vi "Autonomous Independent.vi"   [LabVIEW 2017]
doc: "This VI is called when autonomous begins, and will automatically be terminated when autonomous ends. You can carry out timed or sensor driven robot movement independently without needing to return to the caller."
uses:
  <vilib>/Rock Robotics/WPI/Solenoid/WPI_SolenoidValue.ctl
  <vilib>/Rock Robotics/Network Tables/NT Read String.vi
  Globals/Robot Global Data.vi
  <vilib>/Rock Robotics/WPI/Utilities/WPI_GetSetVariantRefNum.vi
  <vilib>/Rock Robotics/Network Tables/NT Write String.vi
  <vilib>/Rock Robotics/WPI/RobotDrive/WPI_RobotDriveArcadeDrive_Standard(NoSaturation).vi
  <vilib>/addons/control/pid/pid.llb/PID (DBL).vi
  <vilib>/addons/control/pid/NI_PID_pid.lvlib
panel:
  # "Be sure to right-click and choose Data Operations>>Make Current Value default if you want to save the array values with the VI"
types:
  T1 = typedef "WPI_SolenoidValue.ctl" = enum16{"Off", "On", "Forward", "Reverse"}
  T2 = typedef "WPI_RobotDriveDevRef.ctl" = cluster{"DevStatus":errorcluster, "Motors[]":T3[], "Square Inputs":bool, "Max Output":dbl}
  T3 = typedef "WPI_MotorControlDeviceRef.ctl" = cluster{"DeviceStatus":errorcluster, "Type":T4, "PWM":cluster{"PWM Channel":T5, "DeadBand":T6}, "CAN":cluster{"Device Number":u8, "SetOutput VI Ref":variant, "GetOutput VI Ref":variant, "Enable VI Ref":variant, "Disable VI Ref":variant, "Data":variant}, "Invert":bool, "DIO PWM":cluster{"PWM \"Enable\" Channel":T5, "DIOChannel":T7, "PWM Rate":dbl}}
  T4 = typedef "WPI_MotorControlType.ctl" = enum16{"PWM", "CAN", "DIO PWM"}
  T5 = typedef "FPGA_DIOPWMChannel.ctl" = enum8{"PWM 0", "PWM 1", "PWM 2", "PWM 3", "PWM 4", "PWM 5", "PWM 6", "PWM 7", "PWM 8", "PWM 9", "PWM MXP 0", "PWM MXP 1", "PWM MXP 2", "PWM MXP 3", "PWM MXP 4", "PWM MXP 5", "PWM MXP 6", "PWM MXP 7", "PWM MXP 8", "PWM MXP 9", "Invalid"}
  T6 = typedef "WPI_PWMDeadband.ctl" = cluster{"Name":string, "maxPositivePwm":i32, "minPositivePwm":i32, "centerPwm":i32, "maxNegativePwm":i32, "minNegativePwm":i32, "angularRange":u16}
  T7 = typedef "FPGA_DIOChannel.ctl" = enum8{"DIO 0", "DIO 1", "DIO 2", "DIO 3", "DIO 4", "DIO 5", "DIO 6", "DIO 7", "DIO 8", "DIO 9", "DIO MXP 0", "DIO MXP 1", "DIO MXP 2", "DIO MXP 3", "DIO MXP 4", "DIO MXP 5", "DIO MXP 6", "DIO MXP 7", "DIO MXP 8", "DIO MXP 9", "DIO MXP 10", "DIO MXP 11", "DIO MXP 12", "DIO MXP 13", "DIO MXP 14", "DIO MXP 15", "SPI Port CS1", "SPI Port CS2", "SPI Port CS3", "SPI Port MISO", "SPI Port MOSI", "Invalid"}
  T8 = cluster{"proportional gain (Kc)":dbl, "integral time (Ti, min)":dbl, "derivative time (Td, min)":dbl}
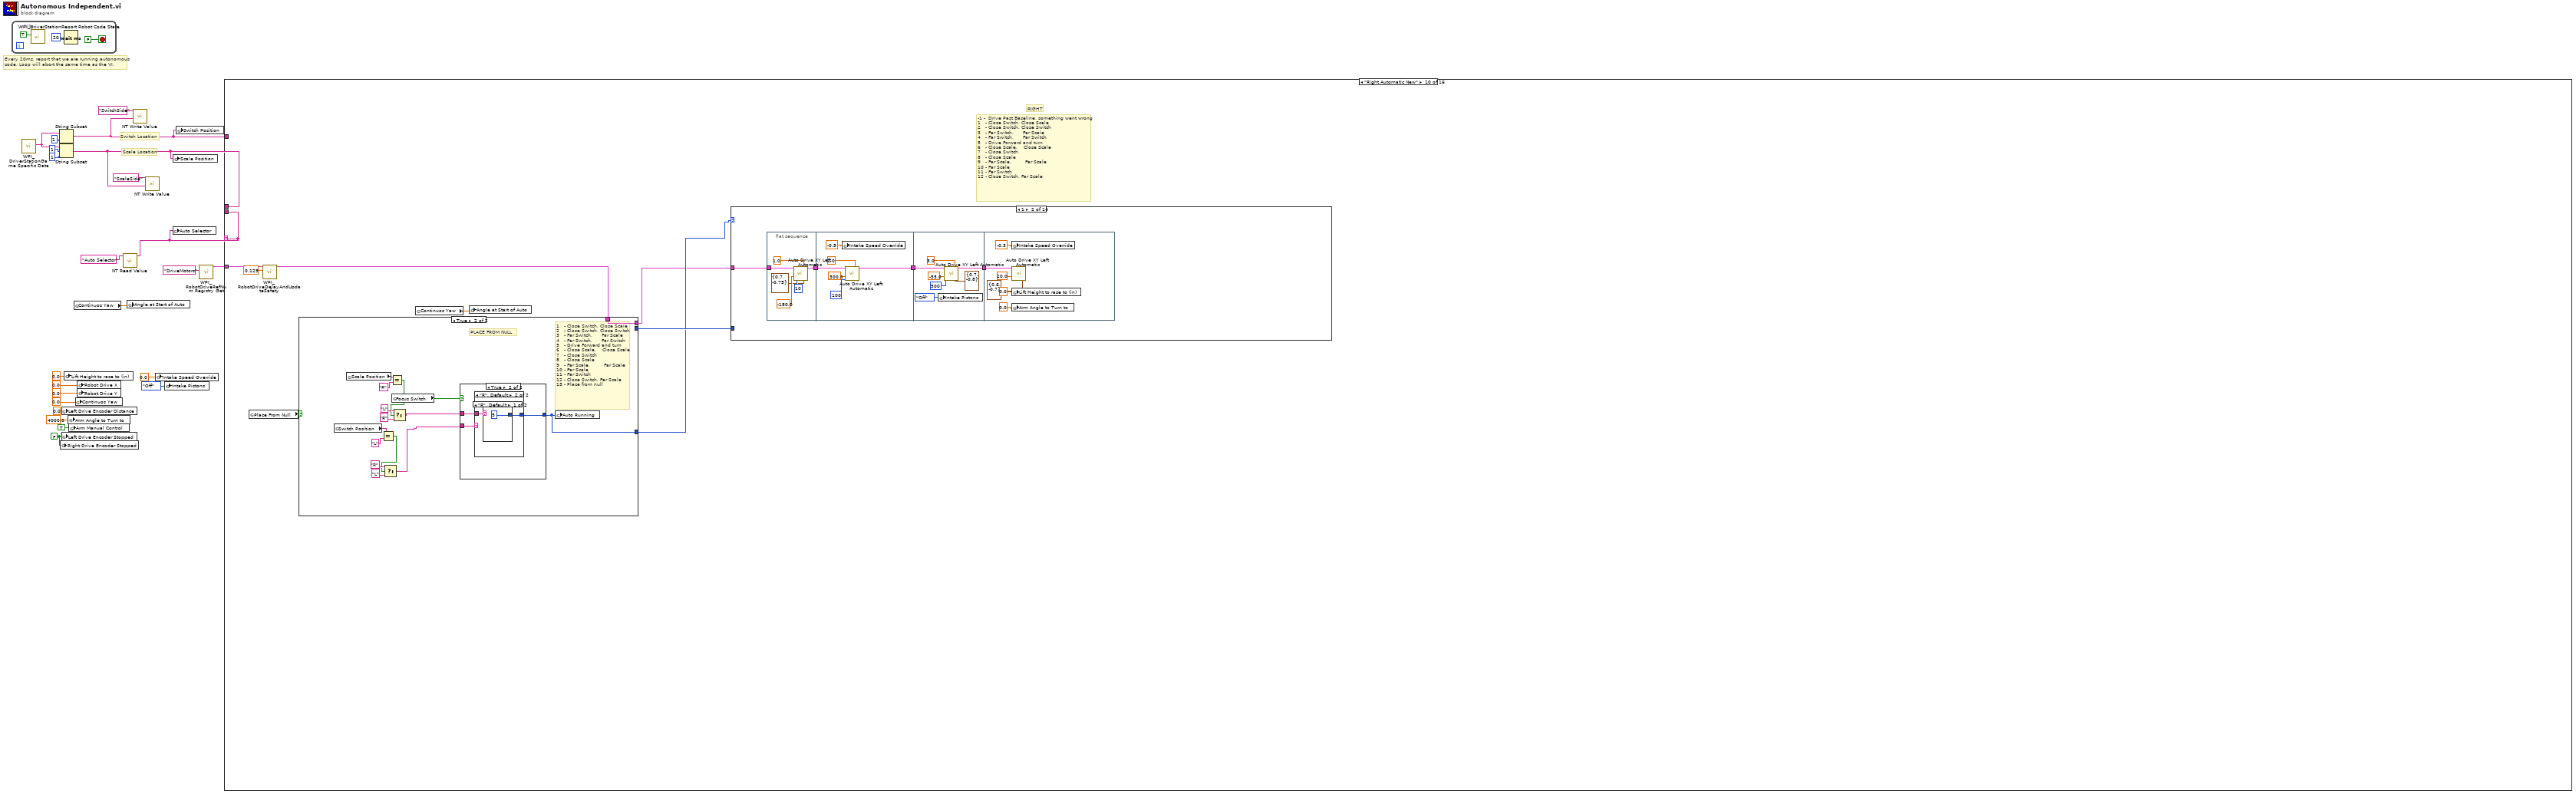
[diagram p0: block diagram]
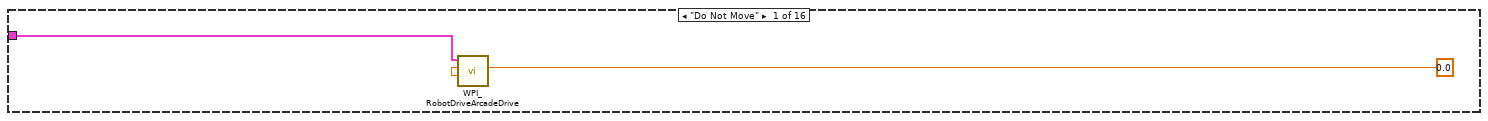
[diagram p2: hidden frame]
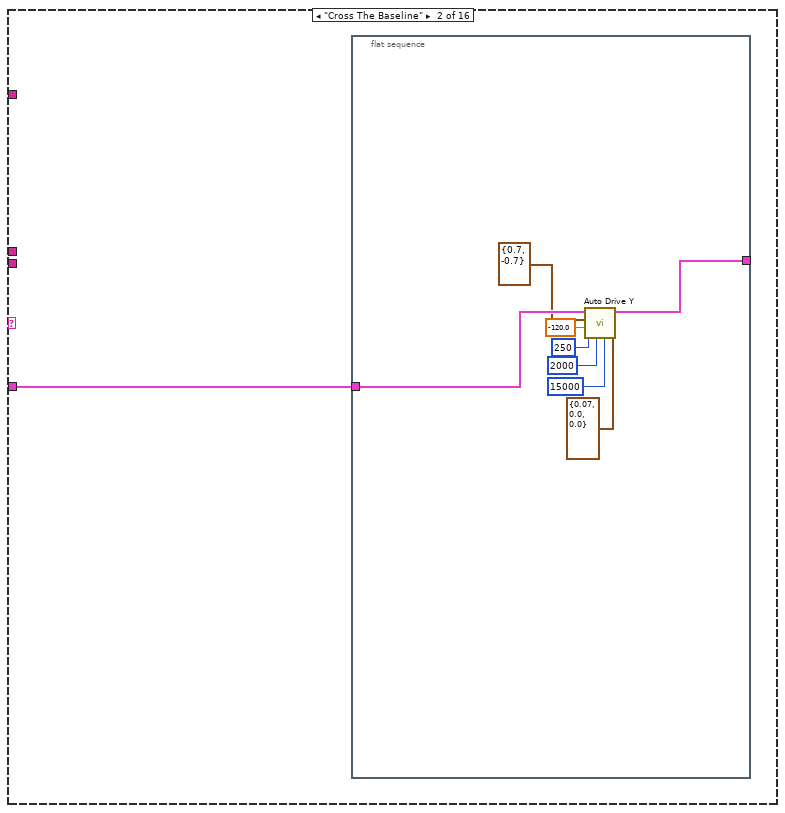
[diagram p3: hidden frame]
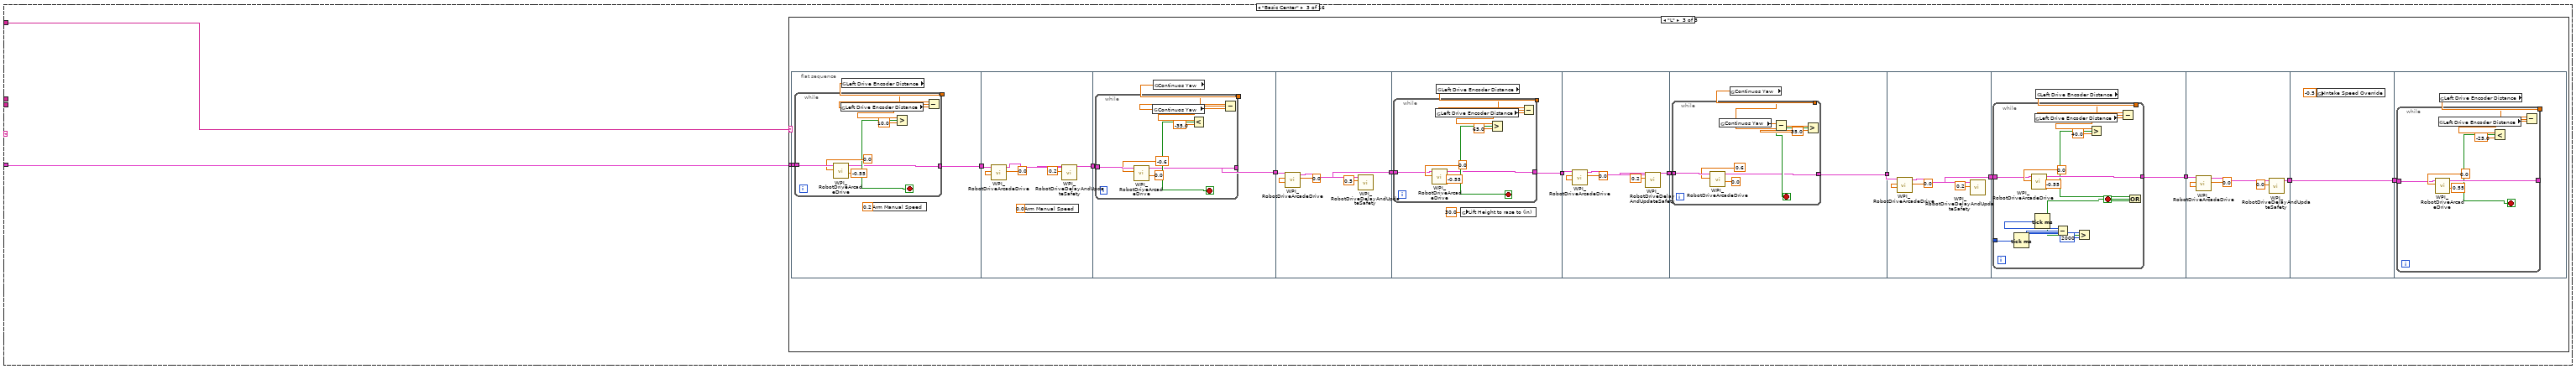
[diagram p4: hidden frame]
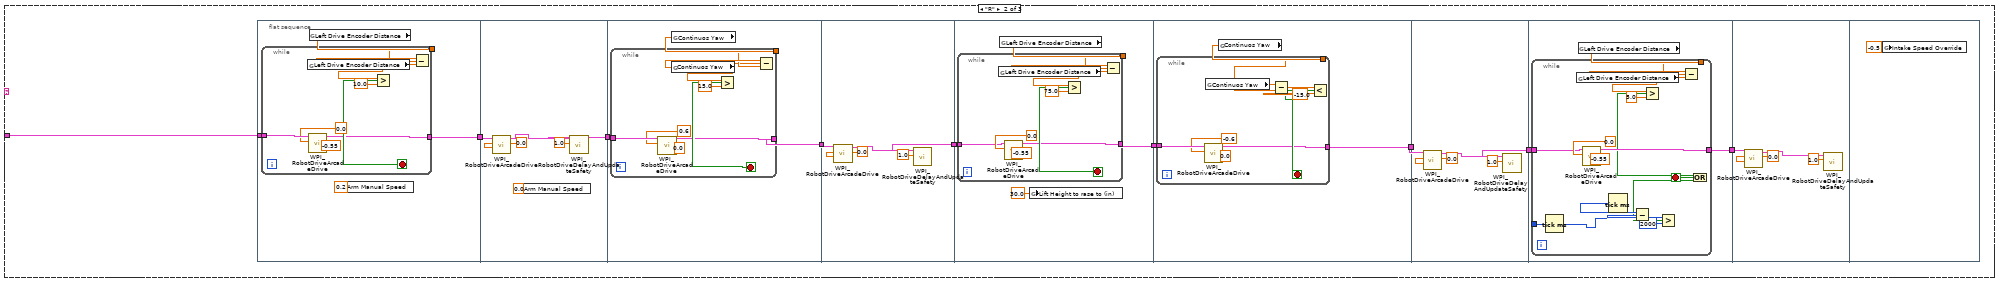
[diagram p6: hidden frame]
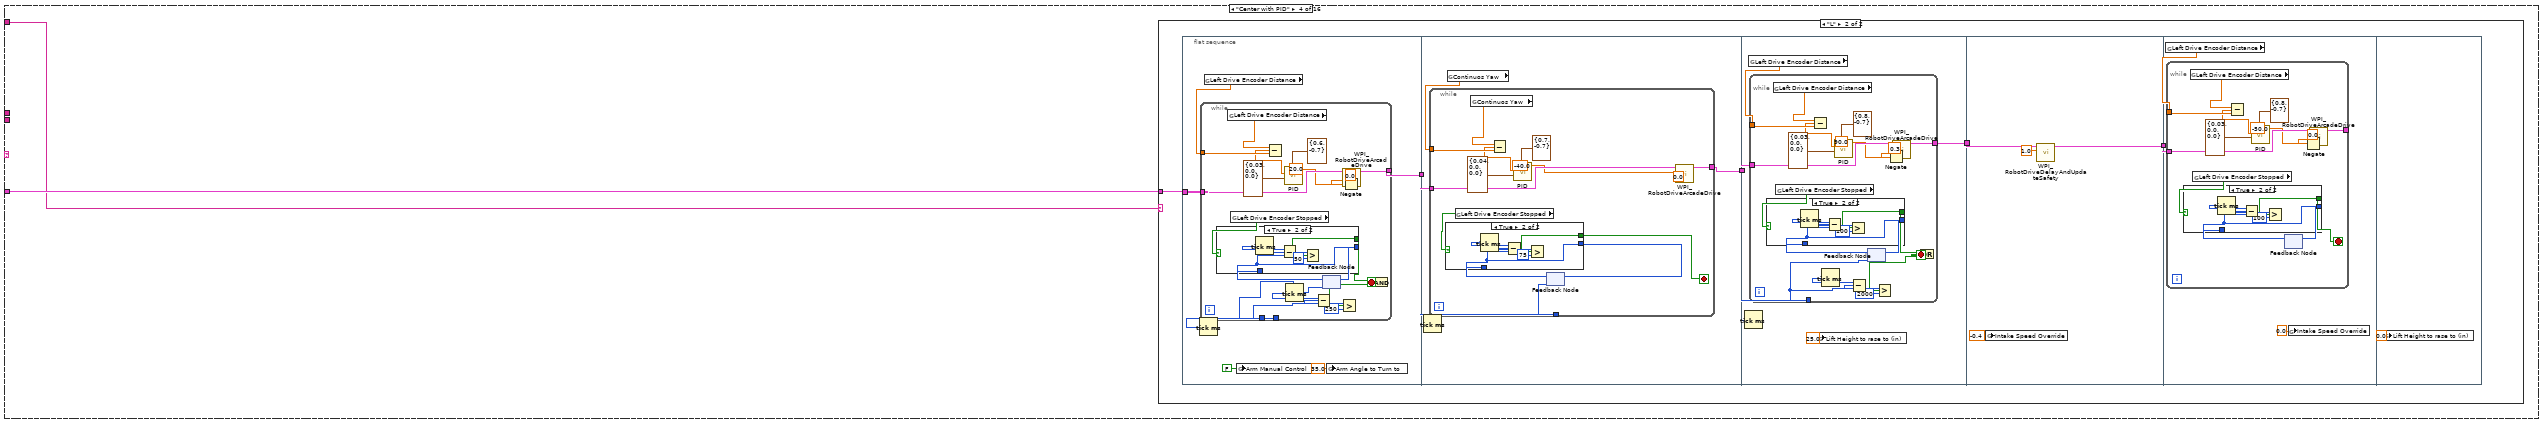
[diagram p7: hidden frame]
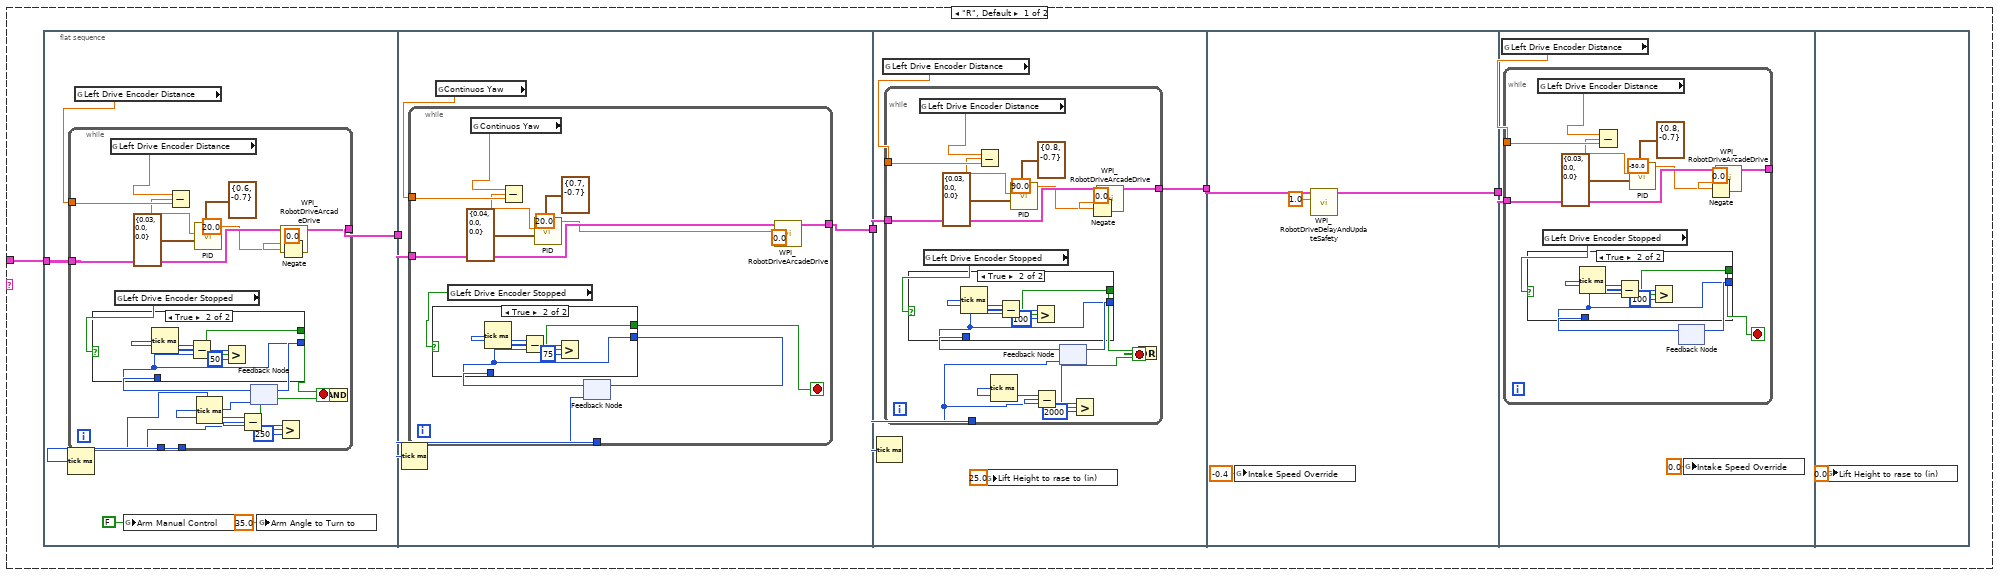
[diagram p8: hidden frame]
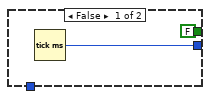
[diagram p9: hidden frame]
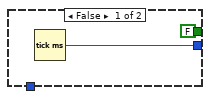
[diagram p10: hidden frame]
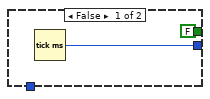
[diagram p11: hidden frame]
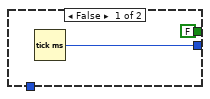
[diagram p12: hidden frame]
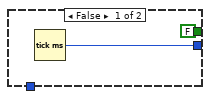
[diagram p13: hidden frame]
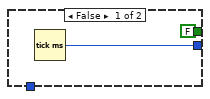
[diagram p14: hidden frame]
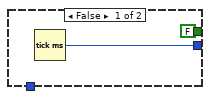
[diagram p15: hidden frame]
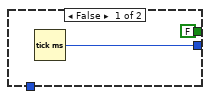
[diagram p16: hidden frame]
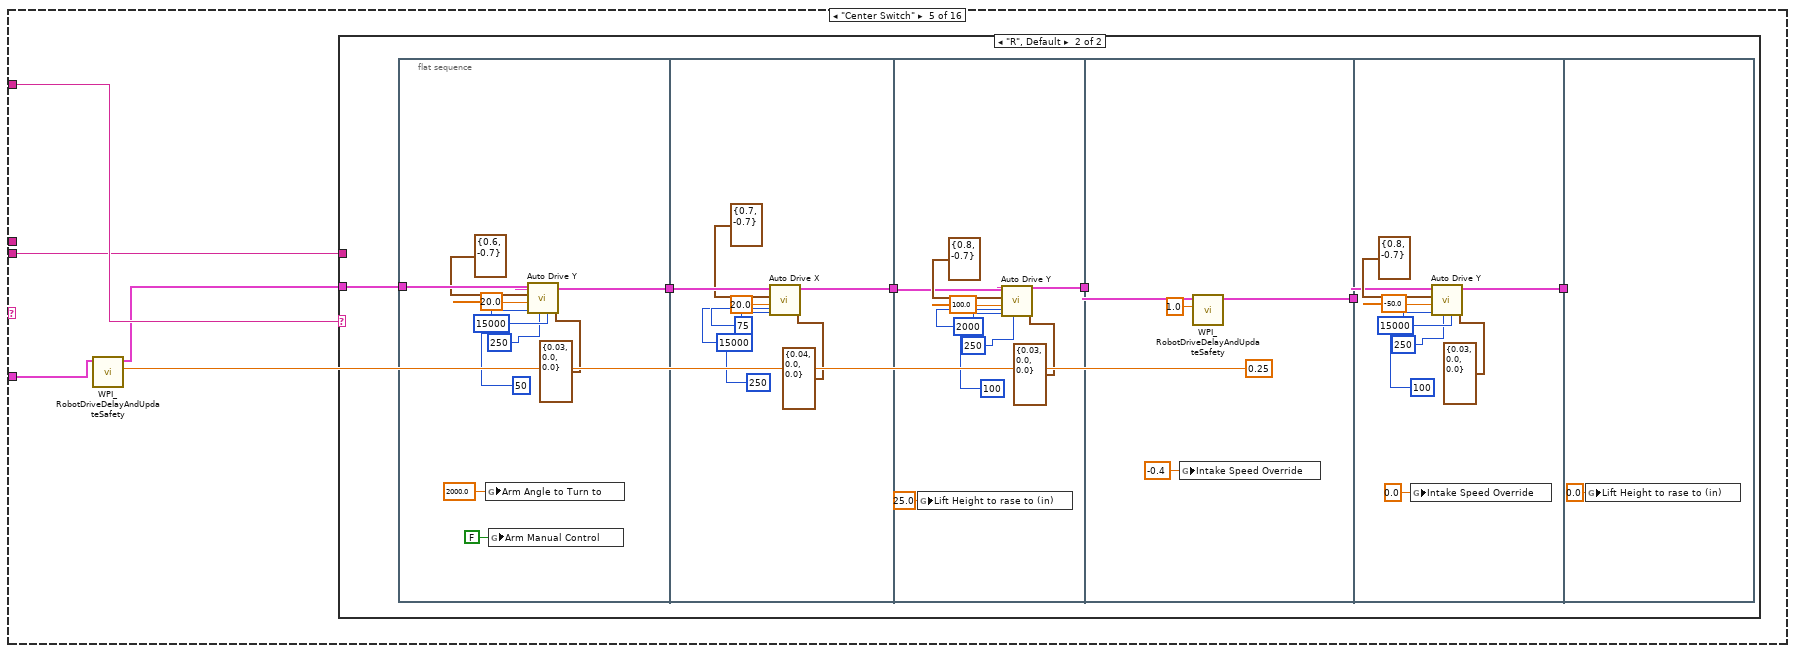
[diagram p17: hidden frame]
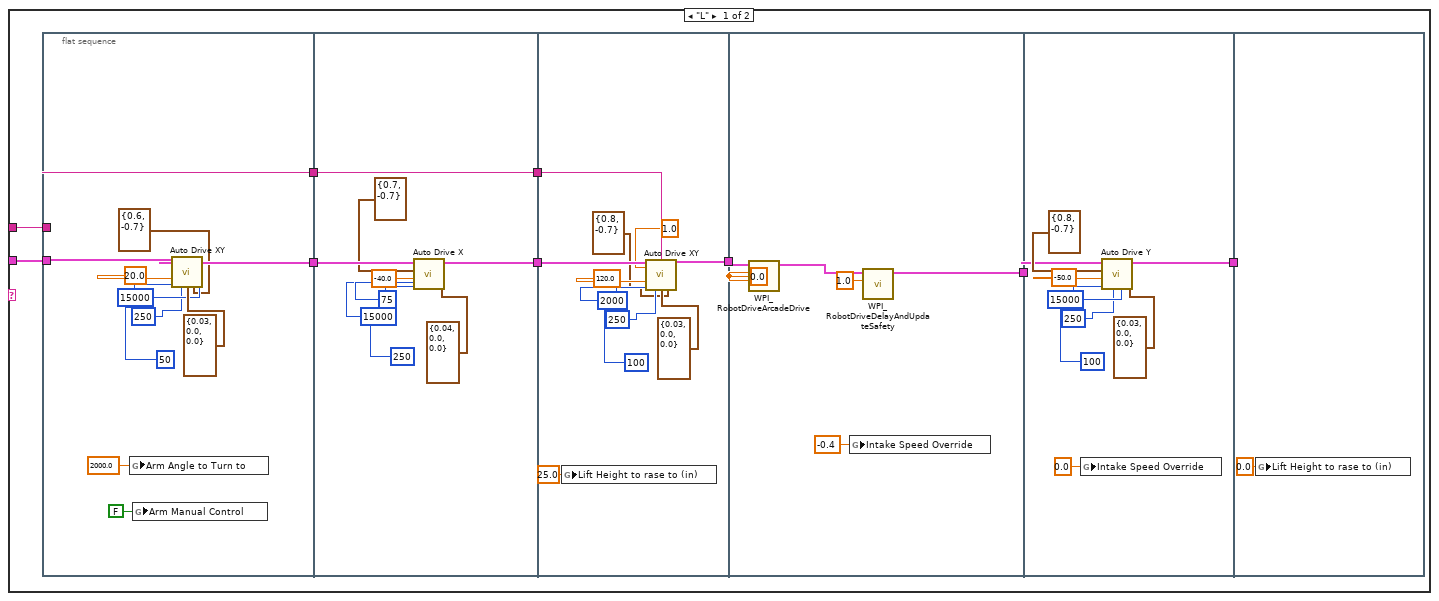
[diagram p18: hidden frame]
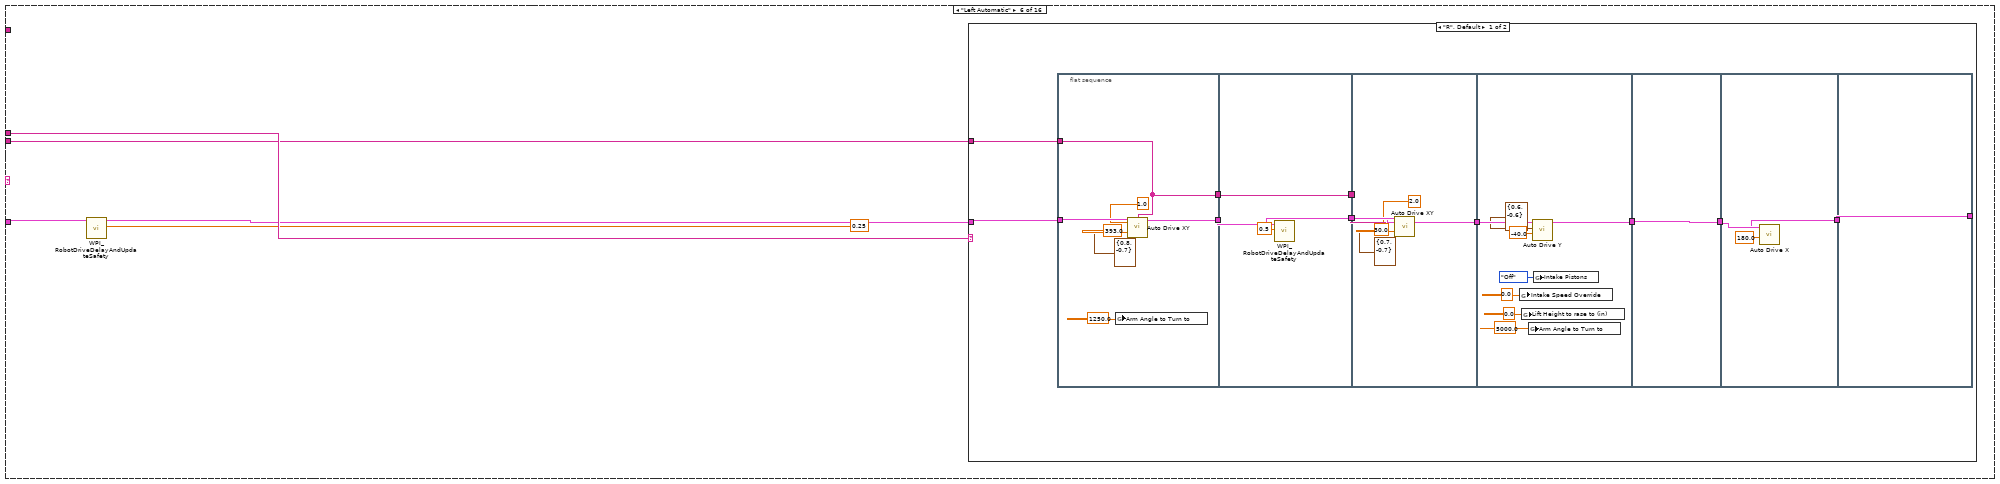
[diagram p19: hidden frame]
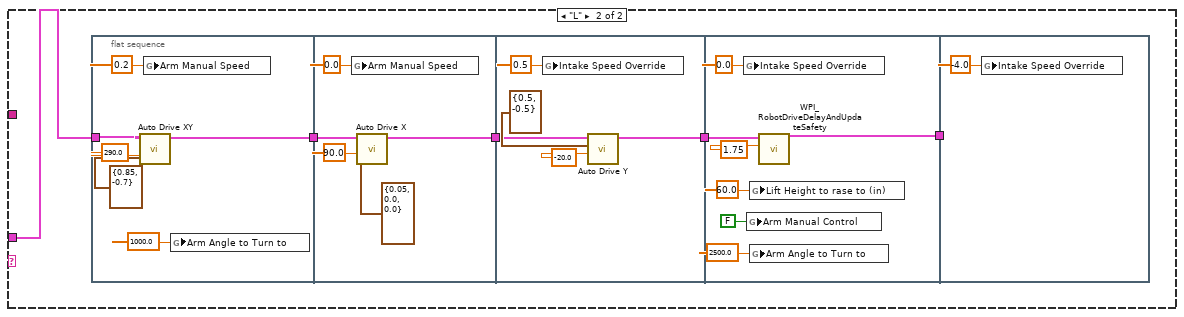
[diagram p20: hidden frame]
diagram:
  w6 = FALSE ("Left Drive Encoder Stopped")
  # "Scale Location"
  # "Switch Location"
  # "Every 20ms, report that we are running autonomous\ncode. Loop will abort the same time as the VI."
  n1 = while {
    stop <- FALSE stop-if-true
    n2 = call <vilib>:"WPI_DriverStationReport Robot Code State.vi"("Autonomous"=TRUE) -> ()  [unwired: 10 in, 1 out]
    n3 = Wait (ms)(milliseconds to wait=u32 20) -> ()  [unwired: 1 out]
  }
  n4 = call <vilib>:"WPI_DriverStationGame Specific Data.vi"() -> ("Game Specific Data"=w20:string)  [unwired: 11 in]
  n5 = String Subset(string=w20, length (rest)=1 ("length (rest)")) -> (substring=w4:string)  [unwired: 1 in]
  n6 = String Subset(string=w20, offset (0)=1, length (rest)=1 ("length (rest)")) -> (substring=w3:string)
  n7 = global write "Robot Global Data.vi" "Right Drive Encoder Stopped"(w6) -> ()
  n8 = global write "Robot Global Data.vi" "Left Drive Encoder Distance"(0.0 ("Lift Height to rase to (in)")) -> ()
  n9 = global write "Robot Global Data.vi" "Left Drive Encoder Stopped"(w6) -> ()
  n10 = global write "Robot Global Data.vi" "Lift Height to rase to (in)"(0.0 ("Lift Height to rase to (in)")) -> ()
  n11 = global write "Robot Global Data.vi" "Arm Angle to Turn to"(4000.0 ("Lift Height to rase to (in)")) -> ()
  n12 = global write "Robot Global Data.vi" "Arm Manual Control"(TRUE ("Arm Manual Control")) -> ()
  n13 = global read "Robot Global Data.vi" "Continuos Yaw"() -> (w1:dbl)
  n14 = global write "Robot Global Data.vi" "Continuos Yaw"(0.0 ("Lift Height to rase to (in)")) -> ()
  n15 = global write "Robot Global Data.vi" "Robot Drive X"(0.0 ("Lift Height to rase to (in)")) -> ()
  n16 = global write "Robot Global Data.vi" "Robot Drive Y"(0.0 ("Lift Height to rase to (in)")) -> ()
  n17 = call-poly <vilib>:"NT Read Value.vi"("Name"="Auto Selector") -> ("String"=w2:string)  [unwired: 9 in, 1 out]
  n18 = global write "Robot Global Data.vi" "Angle at Start of Auto"(w1) -> ()
  n19 = call-poly <vilib>:"NT Write Value.vi"("String"=w4, "Name"="SwitchSide") -> ()  [unwired: 9 in, 1 out]
  n20 = call-poly <vilib>:"NT Write Value.vi"("String"=w3, "Name"="ScaleSide") -> ()  [unwired: 9 in, 1 out]
  n21 = global write "Robot Global Data.vi" "Intake Speed Override"(0.0 ("Lift Height to rase to (in)")) -> ()
  n22 = global write "Robot Global Data.vi" "Intake Pistons"(WPI_SolenoidValue."Off" ("Intake Pistons")) -> ()
  n23 = global write "Robot Global Data.vi" "Auto Selector"(w2) -> ()
  n24 = global write "Robot Global Data.vi" "Scale Position"(w3) -> ()
  n25 = global write "Robot Global Data.vi" "Switch Position"(w4) -> ()
  n26 = call <vilib>:"WPI_RobotDriveRefNum Registry Get.vi"("refnum name"="DriveMotors") -> ("RobotDriveDevRef"=w16:T2)  [unwired: 9 in, 1 out]
  n27 = case shown="\"Right Automatic New\"" w2 {
    tunnel: w4 -> [_ _ w39 w259 w523 _ _ w775 _ _ _ w2264 w2303 _ _ _]
    tunnel: w3 -> [_ _ _ _ _ w631 w705 w780 _ _ _ _ _ w2403 w2569 w2646]
    tunnel: w16 -> [w28 w29 w38 w260 w522 w628 w702 w778 w859 w1340 w1854 w2265 w2301 w2404 w2570 w2647]
    tunnel: w2 -> [_ _ _ _ w519 w630 w704 w779 _ _ _ _ _ _ _ _]
    frame "Do Not Move" {
      w27 = 0.0 ("X axis value")
      n28 = call-poly <vilib>:"WPI_RobotDriveArcadeDrive.vi"("Y axis value"=w27, "X axis value"=w27, "RobotDriveDevRef"=w28) -> ()  [unwired: 6 in, 3 out]
    }
    frame "Cross The Baseline" {
      n29 = flat-sequence {
        tunnel: w29 -> [w37]
        tunnel: [w36] -> _
        frame #0 {
          n30 = call "Auto Drive Y.vi"("PID Gains"=T8 {"proportional gain (Kc)"=0.07, "integral time (Ti, min)"=0.0, "derivative time (Td, min)"=0.0}, "Max Time (ms)"=u32 15000, "Min Time (ms)"=u32 2000, "Time to Settle (ms)"=u32 250, "Distance (in)"=-120.0, "Motor Output Range"=cluster{"output high":dbl, "output low":dbl} {"output high"=0.7, "output low"=-0.7}, "RobotDriveDevRef In"=w37) -> ("RobotDriveDevRef Out"=w36:T2)  [unwired: 4 in]
        }
      }
    }
    frame "Basic Center" {
      n31 = case shown="\"L\"" w39 {
        tunnel: w38 -> [_ w48 w150]
        frame "Unknown Value", Default {
        }
        frame "R" {
          n32 = flat-sequence {
            tunnel: w48 -> [w52]
            tunnel: [w50] -> w47
            tunnel: w47 -> [w65]
            tunnel: [w67] -> w46
            tunnel: [w68] -> w45
            tunnel: w46 -> [w70]
            tunnel: w45 -> [w81]
            tunnel: [w83] -> w44
            tunnel: w44 -> [w87]
            tunnel: [w85] -> w43
            tunnel: w43 -> [w99]
            tunnel: [w98] -> w42
            tunnel: w42 -> [w111]
            tunnel: [w110] -> w41
            tunnel: w41 -> [w117]
            tunnel: [w116] -> w40
            tunnel: w40 -> [w134]
            frame #0 {
              n33 = global read "Robot Global Data.vi" "Left Drive Encoder Distance"() -> (w51:dbl)
              n34 = while {
                tunnel: w52 -> [w60]
                tunnel: [w56] -> w50
                tunnel: w51 -> [w54]
                stop <- w57 stop-if-true
                n35 = global read "Robot Global Data.vi" "Left Drive Encoder Distance"() -> (w55:dbl)
                n36 = call-poly <vilib>:"WPI_RobotDriveArcadeDrive.vi"("Y axis value"=-0.55, "X axis value"=0.0, "RobotDriveDevRef"=w60) -> ("RobotDriveDevRef"=w56:T2)  [unwired: 6 in, 2 out]
                n37 = Subtract(x=w55, y=w54) -> (x-y=w53:dbl)
                n38 = Greater?(x=w53, y=10.0) -> (0:w57:bool)
              }
              n39 = global write "Robot Global Data.vi" "Arm Manual Speed"(0.2 ("Left Drive Encoder Distance")) -> ()
            }
            frame #1 {
              w63 = 0.0 ("X axis value")
              n40 = call-poly <vilib>:"WPI_RobotDriveArcadeDrive.vi"("Y axis value"=w63, "X axis value"=w63, "RobotDriveDevRef"=w65) -> ("RobotDriveDevRef"=w64:T2)  [unwired: 6 in, 2 out]
              n41 = global write "Robot Global Data.vi" "Arm Manual Speed"(0.0 ("Left Drive Encoder Distance")) -> ()
              n42 = call <vilib>:"WPI_RobotDriveDelayAndUpdateSafety.vi"("Delay (s)"=1.0, "RobotDriveDevRef"=w64) -> ("RobotDriveDevRef 2"=w67:T2)  [unwired: 8 in, 1 out]
            }
            frame #2 {
              n43 = global read "Robot Global Data.vi" "Continuos Yaw"() -> (w69:dbl)
              n44 = while {
                tunnel: w70 -> [w78]
                tunnel: [w75] -> w68
                tunnel: w69 -> [w73]
                stop <- w76 stop-if-true
                n45 = call-poly <vilib>:"WPI_RobotDriveArcadeDrive.vi"("Y axis value"=0.0, "X axis value"=0.6, "RobotDriveDevRef"=w78) -> ("RobotDriveDevRef"=w75:T2)  [unwired: 6 in, 2 out]
                n46 = global read "Robot Global Data.vi" "Continuos Yaw"() -> (w74:dbl)
                n47 = Subtract(x=w74, y=w73) -> (x-y=w72:dbl)
                n48 = Greater?(x=w72, y=15.0) -> (0:w76:bool)
              }
            }
            frame #3 {
              w82 = 0.0 ("X axis value")
              n49 = call-poly <vilib>:"WPI_RobotDriveArcadeDrive.vi"("Y axis value"=w82, "X axis value"=w82, "RobotDriveDevRef"=w81) -> ("RobotDriveDevRef"=w80:T2)  [unwired: 6 in, 2 out]
              n50 = call <vilib>:"WPI_RobotDriveDelayAndUpdateSafety.vi"("Delay (s)"=1.0, "RobotDriveDevRef"=w80) -> ("RobotDriveDevRef 2"=w83:T2)  [unwired: 8 in, 1 out]
            }
            frame #4 {
              n51 = global read "Robot Global Data.vi" "Left Drive Encoder Distance"() -> (w88:dbl)
              n52 = while {
                tunnel: [w93] -> w85
                tunnel: w88 -> [w91]
                tunnel: w87 -> [w89]
                stop <- w94 stop-if-true
                n53 = global read "Robot Global Data.vi" "Left Drive Encoder Distance"() -> (w92:dbl)
                n54 = call-poly <vilib>:"WPI_RobotDriveArcadeDrive.vi"("Y axis value"=-0.55, "X axis value"=0.0, "RobotDriveDevRef"=w89) -> ("RobotDriveDevRef"=w93:T2)  [unwired: 6 in, 2 out]
                n55 = Subtract(x=w92, y=w91) -> (x-y=w90:dbl)
                n56 = Greater?(x=w90, y=75.0) -> (0:w94:bool)
              }
              n57 = global write "Robot Global Data.vi" "Lift Height to rase to (in)"(30.0 ("Lift Height to rase to (in)")) -> ()
            }
            frame #5 {
              n58 = global read "Robot Global Data.vi" "Continuos Yaw"() -> (w100:dbl)
              n59 = while {
                tunnel: w99 -> [w108]
                tunnel: [w105] -> w98
                tunnel: w100 -> [w103]
                stop <- w106 stop-if-true
                n60 = call-poly <vilib>:"WPI_RobotDriveArcadeDrive.vi"("Y axis value"=0.0, "X axis value"=-0.6, "RobotDriveDevRef"=w108) -> ("RobotDriveDevRef"=w105:T2)  [unwired: 6 in, 2 out]
                n61 = global read "Robot Global Data.vi" "Continuos Yaw"() -> (w104:dbl)
                n62 = Subtract(x=w104, y=w103) -> (x-y=w102:dbl)
                n63 = Less?(x=w102, y=-15.0) -> (x < y?=w106:bool)
              }
            }
            frame #6 {
              w113 = 0.0 ("X axis value")
              n64 = call-poly <vilib>:"WPI_RobotDriveArcadeDrive.vi"("Y axis value"=w113, "X axis value"=w113, "RobotDriveDevRef"=w111) -> ("RobotDriveDevRef"=w114:T2)  [unwired: 6 in, 2 out]
              n65 = call <vilib>:"WPI_RobotDriveDelayAndUpdateSafety.vi"("Delay (s)"=1.0, "RobotDriveDevRef"=w114) -> ("RobotDriveDevRef 2"=w110:T2)  [unwired: 8 in, 1 out]
            }
            frame #7 {
              n66 = Tick Count (ms)() -> (millisecond timer value=w115:u32)
              n67 = global read "Robot Global Data.vi" "Left Drive Encoder Distance"() -> (w118:dbl)
              n68 = while {
                tunnel: [w130] -> w116
                tunnel: w118 -> [w128]
                tunnel: w117 -> [w126]
                tunnel: w115 -> [w122]
                stop <- w121 stop-if-true
                n69 = global read "Robot Global Data.vi" "Left Drive Encoder Distance"() -> (w129:dbl)
                n70 = call-poly <vilib>:"WPI_RobotDriveArcadeDrive.vi"("Y axis value"=-0.55, "X axis value"=0.0, "RobotDriveDevRef"=w126) -> ("RobotDriveDevRef"=w130:T2)  [unwired: 6 in, 2 out]
                n71 = Tick Count (ms)() -> (millisecond timer value=w125:u32)
                n72 = Subtract(x=w125, y=w122) -> (x-y=w124:u32)
                n73 = Greater?(x=w124, y=u32 2000) -> (0:w119:bool)
                n74 = Subtract(x=w129, y=w128) -> (x-y=w127:dbl)
                n75 = Greater?(x=w127, y=5.0) -> (0:w120:bool)
                n76 = Or(x=w120, y=w119) -> (x .or. y?=w121:bool)
              }
            }
            frame #8 {
              w136 = 0.0 ("X axis value")
              n77 = call-poly <vilib>:"WPI_RobotDriveArcadeDrive.vi"("Y axis value"=w136, "X axis value"=w136, "RobotDriveDevRef"=w134) -> ("RobotDriveDevRef"=w135:T2)  [unwired: 6 in, 2 out]
              n78 = call <vilib>:"WPI_RobotDriveDelayAndUpdateSafety.vi"("Delay (s)"=1.0, "RobotDriveDevRef"=w135) -> ()  [unwired: 8 in, 2 out]
            }
            frame #9 {
              n79 = global write "Robot Global Data.vi" "Intake Speed Override"(-0.5 ("Intake Speed Override")) -> ()
            }
          }
        }
        frame "L" {
          n80 = flat-sequence {
            tunnel: w150 -> [w154]
            tunnel: [w152] -> w149
            tunnel: w149 -> [w167]
            tunnel: [w169] -> w148
            tunnel: [w170] -> w147
            tunnel: w148 -> [w172]
            tunnel: w147 -> [w183]
            tunnel: [w185] -> w146
            tunnel: w146 -> [w189]
            tunnel: [w187] -> w142
            tunnel: w142 -> [w201]
            tunnel: [w200] -> w141
            tunnel: [w205] -> w145
            tunnel: w141 -> [w206]
            tunnel: w145 -> [w218]
            tunnel: [w217] -> w144
            tunnel: w144 -> [w224]
            tunnel: [w223] -> w143
            tunnel: w143 -> [w242]
            tunnel: [w241] -> w139
            tunnel: [w246] -> w140
            tunnel: w139 -> [w246]
            tunnel: w140 -> [w248]
            frame #0 {
              n81 = global read "Robot Global Data.vi" "Left Drive Encoder Distance"() -> (w153:dbl)
              n82 = while {
                tunnel: w154 -> [w162]
                tunnel: [w158] -> w152
                tunnel: w153 -> [w156]
                stop <- w159 stop-if-true
                n83 = call-poly <vilib>:"WPI_RobotDriveArcadeDrive.vi"("Y axis value"=-0.55, "X axis value"=0.0, "RobotDriveDevRef"=w162) -> ("RobotDriveDevRef"=w158:T2)  [unwired: 6 in, 2 out]
                n84 = global read "Robot Global Data.vi" "Left Drive Encoder Distance"() -> (w157:dbl)
                n85 = Subtract(x=w157, y=w156) -> (x-y=w155:dbl)
                n86 = Greater?(x=w155, y=10.0) -> (0:w159:bool)
              }
              n87 = global write "Robot Global Data.vi" "Arm Manual Speed"(0.2 ("Left Drive Encoder Distance")) -> ()
            }
            frame #1 {
              w165 = 0.0 ("X axis value")
              n88 = call-poly <vilib>:"WPI_RobotDriveArcadeDrive.vi"("Y axis value"=w165, "X axis value"=w165, "RobotDriveDevRef"=w167) -> ("RobotDriveDevRef"=w166:T2)  [unwired: 6 in, 2 out]
              n89 = global write "Robot Global Data.vi" "Arm Manual Speed"(0.0 ("Left Drive Encoder Distance")) -> ()
              n90 = call <vilib>:"WPI_RobotDriveDelayAndUpdateSafety.vi"("Delay (s)"=0.2, "RobotDriveDevRef"=w166) -> ("RobotDriveDevRef 2"=w169:T2)  [unwired: 8 in, 1 out]
            }
            frame #2 {
              n91 = global read "Robot Global Data.vi" "Continuos Yaw"() -> (w171:dbl)
              n92 = while {
                tunnel: w172 -> [w180]
                tunnel: [w177] -> w170
                tunnel: w171 -> [w175]
                stop <- w178 stop-if-true
                n93 = call-poly <vilib>:"WPI_RobotDriveArcadeDrive.vi"("Y axis value"=0.0, "X axis value"=-0.6, "RobotDriveDevRef"=w180) -> ("RobotDriveDevRef"=w177:T2)  [unwired: 6 in, 2 out]
                n94 = global read "Robot Global Data.vi" "Continuos Yaw"() -> (w176:dbl)
                n95 = Subtract(x=w176, y=w175) -> (x-y=w174:dbl)
                n96 = Less?(x=w174, y=-35.0) -> (x < y?=w178:bool)
              }
            }
            frame #3 {
              w184 = 0.0 ("X axis value")
              n97 = call-poly <vilib>:"WPI_RobotDriveArcadeDrive.vi"("Y axis value"=w184, "X axis value"=w184, "RobotDriveDevRef"=w183) -> ("RobotDriveDevRef"=w182:T2)  [unwired: 6 in, 2 out]
              n98 = call <vilib>:"WPI_RobotDriveDelayAndUpdateSafety.vi"("Delay (s)"=0.5, "RobotDriveDevRef"=w182) -> ("RobotDriveDevRef 2"=w185:T2)  [unwired: 8 in, 1 out]
            }
            frame #4 {
              n99 = global read "Robot Global Data.vi" "Left Drive Encoder Distance"() -> (w190:dbl)
              n100 = while {
                tunnel: [w195] -> w187
                tunnel: w190 -> [w193]
                tunnel: w189 -> [w191]
                stop <- w196 stop-if-true
                n101 = call-poly <vilib>:"WPI_RobotDriveArcadeDrive.vi"("Y axis value"=-0.55, "X axis value"=0.0, "RobotDriveDevRef"=w191) -> ("RobotDriveDevRef"=w195:T2)  [unwired: 6 in, 2 out]
                n102 = global read "Robot Global Data.vi" "Left Drive Encoder Distance"() -> (w194:dbl)
                n103 = Subtract(x=w194, y=w193) -> (x-y=w192:dbl)
                n104 = Greater?(x=w192, y=65.0) -> (0:w196:bool)
              }
              n105 = global write "Robot Global Data.vi" "Lift Height to rase to (in)"(30.0 ("Lift Height to rase to (in)")) -> ()
            }
            frame #5 {
              w203 = 0.0 ("X axis value")
              n106 = call-poly <vilib>:"WPI_RobotDriveArcadeDrive.vi"("Y axis value"=w203, "X axis value"=w203, "RobotDriveDevRef"=w201) -> ("RobotDriveDevRef"=w202:T2)  [unwired: 6 in, 2 out]
              n107 = call <vilib>:"WPI_RobotDriveDelayAndUpdateSafety.vi"("Delay (s)"=0.2, "RobotDriveDevRef"=w202) -> ("RobotDriveDevRef 2"=w200:T2)  [unwired: 8 in, 1 out]
            }
            frame #6 {
              n108 = global read "Robot Global Data.vi" "Continuos Yaw"() -> (w207:dbl)
              n109 = while {
                tunnel: w206 -> [w215]
                tunnel: [w212] -> w205
                tunnel: w207 -> [w210]
                stop <- w213 stop-if-true
                n110 = call-poly <vilib>:"WPI_RobotDriveArcadeDrive.vi"("Y axis value"=0.0, "X axis value"=0.6, "RobotDriveDevRef"=w215) -> ("RobotDriveDevRef"=w212:T2)  [unwired: 6 in, 2 out]
                n111 = global read "Robot Global Data.vi" "Continuos Yaw"() -> (w211:dbl)
                n112 = Subtract(x=w211, y=w210) -> (x-y=w209:dbl)
                n113 = Greater?(x=w209, y=35.0) -> (0:w213:bool)
              }
            }
            frame #7 {
              w220 = 0.0 ("X axis value")
              n114 = call-poly <vilib>:"WPI_RobotDriveArcadeDrive.vi"("Y axis value"=w220, "X axis value"=w220, "RobotDriveDevRef"=w218) -> ("RobotDriveDevRef"=w221:T2)  [unwired: 6 in, 2 out]
              n115 = call <vilib>:"WPI_RobotDriveDelayAndUpdateSafety.vi"("Delay (s)"=0.2, "RobotDriveDevRef"=w221) -> ("RobotDriveDevRef 2"=w217:T2)  [unwired: 8 in, 1 out]
            }
            frame #8 {
              n116 = Tick Count (ms)() -> (millisecond timer value=w222:u32)
              n117 = global read "Robot Global Data.vi" "Left Drive Encoder Distance"() -> (w225:dbl)
              n118 = while {
                tunnel: [w237] -> w223
                tunnel: w225 -> [w235]
                tunnel: w224 -> [w233]
                tunnel: w222 -> [w231]
                stop <- w228 stop-if-true
                n119 = call-poly <vilib>:"WPI_RobotDriveArcadeDrive.vi"("Y axis value"=-0.55, "X axis value"=0.0, "RobotDriveDevRef"=w233) -> ("RobotDriveDevRef"=w237:T2)  [unwired: 6 in, 2 out]
                n120 = global read "Robot Global Data.vi" "Left Drive Encoder Distance"() -> (w236:dbl)
                n121 = Tick Count (ms)() -> (millisecond timer value=w232:u32)
                n122 = Subtract(x=w232, y=w231) -> (x-y=w230:u32)
                n123 = Greater?(x=w230, y=u32 2000) -> (0:w226:bool)
                n124 = Subtract(x=w236, y=w235) -> (x-y=w234:dbl)
                n125 = Greater?(x=w234, y=40.0) -> (0:w227:bool)
                n126 = Or(x=w227, y=w226) -> (x .or. y?=w228:bool)
              }
            }
            frame #9 {
              w244 = 0.0 ("X axis value")
              n127 = call-poly <vilib>:"WPI_RobotDriveArcadeDrive.vi"("Y axis value"=w244, "X axis value"=w244, "RobotDriveDevRef"=w242) -> ("RobotDriveDevRef"=w243:T2)  [unwired: 6 in, 2 out]
              n128 = call <vilib>:"WPI_RobotDriveDelayAndUpdateSafety.vi"("Delay (s)"=0.0, "RobotDriveDevRef"=w243) -> ("RobotDriveDevRef 2"=w241:T2)  [unwired: 8 in, 1 out]
            }
            frame #10 {
              n129 = global write "Robot Global Data.vi" "Intake Speed Override"(-0.5 ("Intake Speed Override")) -> ()
            }
            frame #11 {
              n130 = global read "Robot Global Data.vi" "Left Drive Encoder Distance"() -> (w249:dbl)
              n131 = while {
                tunnel: [w255] -> _
                tunnel: w249 -> [w253]
                tunnel: w248 -> [w251]
                stop <- w250 stop-if-true
                n132 = call-poly <vilib>:"WPI_RobotDriveArcadeDrive.vi"("Y axis value"=0.55, "X axis value"=0.0, "RobotDriveDevRef"=w251) -> ("RobotDriveDevRef"=w255:T2)  [unwired: 6 in, 2 out]
                n133 = global read "Robot Global Data.vi" "Left Drive Encoder Distance"() -> (w254:dbl)
                n134 = Subtract(x=w254, y=w253) -> (x-y=w252:dbl)
                n135 = Less?(x=w252, y=-25.0) -> (x < y?=w250:bool)
              }
            }
          }
        }
      }
    }
    frame "Center with PID" {
      n136 = case shown="\"L\"" w259 {
        tunnel: w260 -> [w261 w390]
        frame "R", Default {
          n137 = flat-sequence {
            tunnel: w261 -> [w269]
            tunnel: [w268] -> w265
            tunnel: w265 -> [w302]
            tunnel: [w301] -> w264
            tunnel: w264 -> [w329]
            tunnel: [w328] -> w263
            tunnel: w263 -> [w362]
            tunnel: [w360] -> w262
            tunnel: w262 -> [w364]
            frame #0 {
              n138 = Tick Count (ms)() -> (millisecond timer value=w266:u32)
              n139 = global read "Robot Global Data.vi" "Left Drive Encoder Distance"() -> (w271:dbl)
              n140 = while {
                tunnel: w269 -> [w290]
                tunnel: w271 -> [w282]
                tunnel: w266 -> [w280]
                tunnel: [w279] -> w268
                tunnel: w266 -> [w275]
                stop <- w274 stop-if-true
                n141 = global read "Robot Global Data.vi" "Left Drive Encoder Distance"() -> (w283:dbl)
                n142 = global read "Robot Global Data.vi" "Left Drive Encoder Stopped"() -> (w286:bool)
                n143 = Subtract(x=w283, y=w282) -> (x-y=w281:dbl)
                n144 = call-poly <vilib>:"PID.vi"("output range"=cluster{"output high":dbl, "output low":dbl} {"output high"=0.6, "output low"=-0.7}, "PID gains"=T8 {"proportional gain (Kc)"=0.03, "integral time (Ti, min)"=0.0, "derivative time (Td, min)"=0.0}, "process variable"=w281, "setpoint"=20.0) -> ("output"=w287:dbl)  [unwired: 6 in, 1 out]
                n145 = Tick Count (ms)() -> (millisecond timer value=w278:u32)
                n146 = Subtract(x=w278, y=w275) -> (x-y=w277:u32)
                n147 = feedback #1(w280) -> (w284:u32)
                n148 = case shown="True" w286 {
                  tunnel: w284 -> [_ w299]
                  tunnel: [w295 w299] -> w285
                  tunnel: [FALSE w296] -> w273
                  frame False {
                    n149 = Tick Count (ms)() -> (millisecond timer value=w295:u32)
                  }
                  frame True {
                    n150 = Tick Count (ms)() -> (millisecond timer value=w300:u32)
                    n151 = Subtract(x=w300, y=w299) -> (x-y=w298:u32)
                    n152 = Greater?(x=w298, y=u32 50) -> (0:w296:bool)
                  }
                }
                n153 = feedback-in #1(w285) -> ()
                n154 = Greater?(x=w277, y=u32 250) -> (0:w272:bool)
                n155 = Negate(x=w287) -> (-x=w288:dbl)
                n156 = call-poly <vilib>:"WPI_RobotDriveArcadeDrive.vi"("Y axis value"=w288, "X axis value"=0.0, "RobotDriveDevRef"=w290) -> ("RobotDriveDevRef"=w279:T2)  [unwired: 6 in, 2 out]
                n157 = And(x=w273, y=w272) -> (x .and. y?=w274:bool)
              }
              n158 = global write "Robot Global Data.vi" "Arm Manual Control"(FALSE ("Arm Manual Control")) -> ()
              n159 = global write "Robot Global Data.vi" "Arm Angle to Turn to"(35.0 ("Arm Manual Speed")) -> ()
            }
            frame #1 {
              n160 = Tick Count (ms)() -> (millisecond timer value=w303:u32)
              n161 = global read "Robot Global Data.vi" "Continuos Yaw"() -> (w304:dbl)
              n162 = while {
                tunnel: w302 -> [w316]
                tunnel: w304 -> [w310]
                tunnel: w303 -> [w308]
                tunnel: [w307] -> w301
                stop <- w312 stop-if-true
                n163 = global read "Robot Global Data.vi" "Left Drive Encoder Stopped"() -> (w315:bool)
                n164 = global read "Robot Global Data.vi" "Continuos Yaw"() -> (w311:dbl)
                n165 = Subtract(x=w311, y=w310) -> (x-y=w309:dbl)
                n166 = call-poly <vilib>:"PID.vi"("output range"=cluster{"output high":dbl, "output low":dbl} {"output high"=0.7, "output low"=-0.7}, "PID gains"=T8 {"proportional gain (Kc)"=0.04, "integral time (Ti, min)"=0.0, "derivative time (Td, min)"=0.0}, "process variable"=w309, "setpoint"=20.0) -> ("output"=w306:dbl)  [unwired: 6 in, 1 out]
                n167 = feedback #2(w308) -> (w313:u32)
                n168 = case shown="True" w315 {
                  tunnel: w313 -> [_ w325]
                  tunnel: [w321 w325] -> w314
                  tunnel: [FALSE w322] -> w312
                  frame False {
                    n169 = Tick Count (ms)() -> (millisecond timer value=w321:u32)
                  }
                  frame True {
                    n170 = Tick Count (ms)() -> (millisecond timer value=w326:u32)
                    n171 = Subtract(x=w326, y=w325) -> (x-y=w324:u32)
                    n172 = Greater?(x=w324, y=u32 75) -> (0:w322:bool)
                  }
                }
                n173 = feedback-in #2(w314) -> ()
                n174 = call-poly <vilib>:"WPI_RobotDriveArcadeDrive.vi"("Y axis value"=0.0, "X axis value"=w306, "RobotDriveDevRef"=w316) -> ("RobotDriveDevRef"=w307:T2)  [unwired: 6 in, 2 out]
              }
            }
            frame #2 {
              n175 = Tick Count (ms)() -> (millisecond timer value=w330:u32)
              n176 = global read "Robot Global Data.vi" "Left Drive Encoder Distance"() -> (w331:dbl)
              n177 = while {
                tunnel: w329 -> [w349]
                tunnel: w331 -> [w341]
                tunnel: w330 -> [w332]
                tunnel: [w339] -> w328
                stop <- w333 stop-if-true
                n178 = global read "Robot Global Data.vi" "Left Drive Encoder Distance"() -> (w342:dbl)
                n179 = global read "Robot Global Data.vi" "Left Drive Encoder Stopped"() -> (w345:bool)
                n180 = Subtract(x=w342, y=w341) -> (x-y=w340:dbl)
                n181 = Tick Count (ms)() -> (millisecond timer value=w338:u32)
                n182 = call-poly <vilib>:"PID.vi"("output range"=cluster{"output high":dbl, "output low":dbl} {"output high"=0.8, "output low"=-0.7}, "PID gains"=T8 {"proportional gain (Kc)"=0.03, "integral time (Ti, min)"=0.0, "derivative time (Td, min)"=0.0}, "process variable"=w340, "setpoint"=90.0) -> ("output"=w346:dbl)  [unwired: 6 in, 1 out]
                n183 = Subtract(x=w338, y=w332) -> (x-y=w337:u32)
                n184 = feedback #3(w332) -> (w343:u32)
                n185 = case shown="True" w345 {
                  tunnel: w343 -> [_ w358]
                  tunnel: [w354 w358] -> w344
                  tunnel: [FALSE w355] -> w335
                  frame False {
                    n186 = Tick Count (ms)() -> (millisecond timer value=w354:u32)
                  }
                  frame True {
                    n187 = Tick Count (ms)() -> (millisecond timer value=w359:u32)
                    n188 = Subtract(x=w359, y=w358) -> (x-y=w357:u32)
                    n189 = Greater?(x=w357, y=u32 100) -> (0:w355:bool)
                  }
                }
                n190 = feedback-in #3(w344) -> ()
                n191 = Greater?(x=w337, y=u32 2000) -> (0:w334:bool)
                n192 = Negate(x=w346) -> (-x=w347:dbl)
                n193 = call-poly <vilib>:"WPI_RobotDriveArcadeDrive.vi"("Y axis value"=w347, "X axis value"=0.0, "RobotDriveDevRef"=w349) -> ("RobotDriveDevRef"=w339:T2)  [unwired: 6 in, 2 out]
                n194 = Or(x=w335, y=w334) -> (x .or. y?=w333:bool)
              }
              n195 = global write "Robot Global Data.vi" "Lift Height to rase to (in)"(25.0 ("Arm Manual Speed")) -> ()
            }
            frame #3 {
              n196 = global write "Robot Global Data.vi" "Intake Speed Override"(-0.4 ("Arm Manual Speed")) -> ()
              n197 = call <vilib>:"WPI_RobotDriveDelayAndUpdateSafety.vi"("Delay (s)"=1.0, "RobotDriveDevRef"=w362) -> ("RobotDriveDevRef 2"=w360:T2)  [unwired: 8 in, 1 out]
            }
            frame #4 {
              n198 = global read "Robot Global Data.vi" "Left Drive Encoder Distance"() -> (w365:dbl)
              n199 = while {
                tunnel: w364 -> [w378]
                tunnel: w365 -> [w370]
                tunnel: [w368] -> _
                stop <- w367 stop-if-true
                n200 = global read "Robot Global Data.vi" "Left Drive Encoder Distance"() -> (w371:dbl)
                n201 = global read "Robot Global Data.vi" "Left Drive Encoder Stopped"() -> (w374:bool)
                n202 = Subtract(x=w371, y=w370) -> (x-y=w369:dbl)
                n203 = call-poly <vilib>:"PID.vi"("output range"=cluster{"output high":dbl, "output low":dbl} {"output high"=0.8, "output low"=-0.7}, "PID gains"=T8 {"proportional gain (Kc)"=0.03, "integral time (Ti, min)"=0.0, "derivative time (Td, min)"=0.0}, "process variable"=w369, "setpoint"=-50.0) -> ("output"=w375:dbl)  [unwired: 6 in, 1 out]
                n204 = feedback #4() -> (w372:u32)  [unwired: 1 in]
                n205 = case shown="True" w374 {
                  tunnel: w372 -> [_ w387]
                  tunnel: [w383 w387] -> w373
                  tunnel: [FALSE w384] -> w367
                  frame False {
                    n206 = Tick Count (ms)() -> (millisecond timer value=w383:u32)
                  }
                  frame True {
                    n207 = Tick Count (ms)() -> (millisecond timer value=w388:u32)
                    n208 = Subtract(x=w388, y=w387) -> (x-y=w386:u32)
                    n209 = Greater?(x=w386, y=u32 100) -> (0:w384:bool)
                  }
                }
                n210 = feedback-in #4(w373) -> ()
                n211 = Negate(x=w375) -> (-x=w376:dbl)
                n212 = call-poly <vilib>:"WPI_RobotDriveArcadeDrive.vi"("Y axis value"=w376, "X axis value"=0.0, "RobotDriveDevRef"=w378) -> ("RobotDriveDevRef"=w368:T2)  [unwired: 6 in, 2 out]
              }
              n213 = global write "Robot Global Data.vi" "Intake Speed Override"(0.0 ("Arm Manual Speed")) -> ()
            }
            frame #5 {
              n214 = global write "Robot Global Data.vi" "Lift Height to rase to (in)"(0.0 ("Arm Manual Speed")) -> ()
            }
          }
        }
        frame "L" {
          n215 = flat-sequence {
            tunnel: w390 -> [w398]
            tunnel: [w397] -> w394
            tunnel: w394 -> [w431]
            tunnel: [w430] -> w393
            tunnel: w393 -> [w458]
            tunnel: [w457] -> w392
            tunnel: w392 -> [w491]
            tunnel: [w489] -> w391
            tunnel: w391 -> [w493]
            frame #0 {
              n216 = Tick Count (ms)() -> (millisecond timer value=w395:u32)
              n217 = global read "Robot Global Data.vi" "Left Drive Encoder Distance"() -> (w400:dbl)
              n218 = while {
                tunnel: w398 -> [w419]
                tunnel: w400 -> [w411]
                tunnel: w395 -> [w409]
                tunnel: [w408] -> w397
                tunnel: w395 -> [w404]
                stop <- w403 stop-if-true
                n219 = global read "Robot Global Data.vi" "Left Drive Encoder Distance"() -> (w412:dbl)
                n220 = global read "Robot Global Data.vi" "Left Drive Encoder Stopped"() -> (w415:bool)
                n221 = Subtract(x=w412, y=w411) -> (x-y=w410:dbl)
                n222 = call-poly <vilib>:"PID.vi"("output range"=cluster{"output high":dbl, "output low":dbl} {"output high"=0.6, "output low"=-0.7}, "PID gains"=T8 {"proportional gain (Kc)"=0.03, "integral time (Ti, min)"=0.0, "derivative time (Td, min)"=0.0}, "process variable"=w410, "setpoint"=20.0) -> ("output"=w416:dbl)  [unwired: 6 in, 1 out]
                n223 = Tick Count (ms)() -> (millisecond timer value=w407:u32)
                n224 = Subtract(x=w407, y=w404) -> (x-y=w406:u32)
                n225 = feedback #5(w409) -> (w413:u32)
                n226 = case shown="True" w415 {
                  tunnel: w413 -> [_ w428]
                  tunnel: [w424 w428] -> w414
                  tunnel: [FALSE w425] -> w402
                  frame False {
                    n227 = Tick Count (ms)() -> (millisecond timer value=w424:u32)
                  }
                  frame True {
                    n228 = Tick Count (ms)() -> (millisecond timer value=w429:u32)
                    n229 = Subtract(x=w429, y=w428) -> (x-y=w427:u32)
                    n230 = Greater?(x=w427, y=u32 50) -> (0:w425:bool)
                  }
                }
                n231 = feedback-in #5(w414) -> ()
                n232 = Greater?(x=w406, y=u32 250) -> (0:w401:bool)
                n233 = Negate(x=w416) -> (-x=w417:dbl)
                n234 = call-poly <vilib>:"WPI_RobotDriveArcadeDrive.vi"("Y axis value"=w417, "X axis value"=0.0, "RobotDriveDevRef"=w419) -> ("RobotDriveDevRef"=w408:T2)  [unwired: 6 in, 2 out]
                n235 = And(x=w402, y=w401) -> (x .and. y?=w403:bool)
              }
              n236 = global write "Robot Global Data.vi" "Arm Manual Control"(FALSE ("Arm Manual Control")) -> ()
              n237 = global write "Robot Global Data.vi" "Arm Angle to Turn to"(35.0 ("Arm Manual Speed")) -> ()
            }
            frame #1 {
              n238 = Tick Count (ms)() -> (millisecond timer value=w432:u32)
              n239 = global read "Robot Global Data.vi" "Continuos Yaw"() -> (w433:dbl)
              n240 = while {
                tunnel: w431 -> [w445]
                tunnel: w433 -> [w439]
                tunnel: w432 -> [w437]
                tunnel: [w436] -> w430
                stop <- w441 stop-if-true
                n241 = global read "Robot Global Data.vi" "Left Drive Encoder Stopped"() -> (w444:bool)
                n242 = global read "Robot Global Data.vi" "Continuos Yaw"() -> (w440:dbl)
                n243 = Subtract(x=w440, y=w439) -> (x-y=w438:dbl)
                n244 = call-poly <vilib>:"PID.vi"("output range"=cluster{"output high":dbl, "output low":dbl} {"output high"=0.7, "output low"=-0.7}, "PID gains"=T8 {"proportional gain (Kc)"=0.04, "integral time (Ti, min)"=0.0, "derivative time (Td, min)"=0.0}, "process variable"=w438, "setpoint"=-40.0) -> ("output"=w435:dbl)  [unwired: 6 in, 1 out]
                n245 = feedback #6(w437) -> (w442:u32)
                n246 = case shown="True" w444 {
                  tunnel: w442 -> [_ w454]
                  tunnel: [w450 w454] -> w443
                  tunnel: [FALSE w451] -> w441
                  frame False {
                    n247 = Tick Count (ms)() -> (millisecond timer value=w450:u32)
                  }
                  frame True {
                    n248 = Tick Count (ms)() -> (millisecond timer value=w455:u32)
                    n249 = Subtract(x=w455, y=w454) -> (x-y=w453:u32)
                    n250 = Greater?(x=w453, y=u32 75) -> (0:w451:bool)
                  }
                }
                n251 = feedback-in #6(w443) -> ()
                n252 = call-poly <vilib>:"WPI_RobotDriveArcadeDrive.vi"("Y axis value"=0.0, "X axis value"=w435, "RobotDriveDevRef"=w445) -> ("RobotDriveDevRef"=w436:T2)  [unwired: 6 in, 2 out]
              }
            }
            frame #2 {
              n253 = Tick Count (ms)() -> (millisecond timer value=w459:u32)
              n254 = global read "Robot Global Data.vi" "Left Drive Encoder Distance"() -> (w460:dbl)
              n255 = while {
                tunnel: w458 -> [w478]
                tunnel: w460 -> [w470]
                tunnel: w459 -> [w461]
                tunnel: [w468] -> w457
                stop <- w462 stop-if-true
                n256 = global read "Robot Global Data.vi" "Left Drive Encoder Distance"() -> (w471:dbl)
                n257 = global read "Robot Global Data.vi" "Left Drive Encoder Stopped"() -> (w474:bool)
                n258 = Subtract(x=w471, y=w470) -> (x-y=w469:dbl)
                n259 = Tick Count (ms)() -> (millisecond timer value=w467:u32)
                n260 = call-poly <vilib>:"PID.vi"("output range"=cluster{"output high":dbl, "output low":dbl} {"output high"=0.8, "output low"=-0.7}, "PID gains"=T8 {"proportional gain (Kc)"=0.03, "integral time (Ti, min)"=0.0, "derivative time (Td, min)"=0.0}, "process variable"=w469, "setpoint"=90.0) -> ("output"=w475:dbl)  [unwired: 6 in, 1 out]
                n261 = Subtract(x=w467, y=w461) -> (x-y=w466:u32)
                n262 = feedback #7(w461) -> (w472:u32)
                n263 = case shown="True" w474 {
                  tunnel: w472 -> [_ w487]
                  tunnel: [w483 w487] -> w473
                  tunnel: [FALSE w484] -> w464
                  frame False {
                    n264 = Tick Count (ms)() -> (millisecond timer value=w483:u32)
                  }
                  frame True {
                    n265 = Tick Count (ms)() -> (millisecond timer value=w488:u32)
                    n266 = Subtract(x=w488, y=w487) -> (x-y=w486:u32)
                    n267 = Greater?(x=w486, y=u32 100) -> (0:w484:bool)
                  }
                }
                n268 = feedback-in #7(w473) -> ()
                n269 = Greater?(x=w466, y=u32 2000) -> (0:w463:bool)
                n270 = Negate(x=w475) -> (-x=w476:dbl)
                n271 = call-poly <vilib>:"WPI_RobotDriveArcadeDrive.vi"("Y axis value"=w476, "X axis value"=0.3, "RobotDriveDevRef"=w478) -> ("RobotDriveDevRef"=w468:T2)  [unwired: 6 in, 2 out]
                n272 = Or(x=w464, y=w463) -> (x .or. y?=w462:bool)
              }
              n273 = global write "Robot Global Data.vi" "Lift Height to rase to (in)"(25.0 ("Arm Manual Speed")) -> ()
            }
            frame #3 {
              n274 = global write "Robot Global Data.vi" "Intake Speed Override"(-0.4 ("Arm Manual Speed")) -> ()
              n275 = call <vilib>:"WPI_RobotDriveDelayAndUpdateSafety.vi"("Delay (s)"=1.0, "RobotDriveDevRef"=w491) -> ("RobotDriveDevRef 2"=w489:T2)  [unwired: 8 in, 1 out]
            }
            frame #4 {
              n276 = global read "Robot Global Data.vi" "Left Drive Encoder Distance"() -> (w494:dbl)
              n277 = while {
                tunnel: w493 -> [w507]
                tunnel: w494 -> [w499]
                tunnel: [w497] -> _
                stop <- w496 stop-if-true
                n278 = global read "Robot Global Data.vi" "Left Drive Encoder Distance"() -> (w500:dbl)
                n279 = global read "Robot Global Data.vi" "Left Drive Encoder Stopped"() -> (w503:bool)
                n280 = Subtract(x=w500, y=w499) -> (x-y=w498:dbl)
                n281 = call-poly <vilib>:"PID.vi"("output range"=cluster{"output high":dbl, "output low":dbl} {"output high"=0.8, "output low"=-0.7}, "PID gains"=T8 {"proportional gain (Kc)"=0.03, "integral time (Ti, min)"=0.0, "derivative time (Td, min)"=0.0}, "process variable"=w498, "setpoint"=-50.0) -> ("output"=w504:dbl)  [unwired: 6 in, 1 out]
                n282 = feedback #8() -> (w501:u32)  [unwired: 1 in]
                n283 = case shown="True" w503 {
                  tunnel: w501 -> [_ w516]
                  tunnel: [w512 w516] -> w502
                  tunnel: [FALSE w513] -> w496
                  frame False {
                    n284 = Tick Count (ms)() -> (millisecond timer value=w512:u32)
                  }
                  frame True {
                    n285 = Tick Count (ms)() -> (millisecond timer value=w517:u32)
                    n286 = Subtract(x=w517, y=w516) -> (x-y=w515:u32)
                    n287 = Greater?(x=w515, y=u32 100) -> (0:w513:bool)
                  }
                }
                n288 = feedback-in #8(w502) -> ()
                n289 = Negate(x=w504) -> (-x=w505:dbl)
                n290 = call-poly <vilib>:"WPI_RobotDriveArcadeDrive.vi"("Y axis value"=w505, "X axis value"=0.0, "RobotDriveDevRef"=w507) -> ("RobotDriveDevRef"=w497:T2)  [unwired: 6 in, 2 out]
              }
              n291 = global write "Robot Global Data.vi" "Intake Speed Override"(0.0 ("Arm Manual Speed")) -> ()
            }
            frame #5 {
              n292 = global write "Robot Global Data.vi" "Lift Height to rase to (in)"(0.0 ("Arm Manual Speed")) -> ()
            }
          }
        }
      }
    }
    frame "Center Switch" {
      n293 = call <vilib>:"WPI_RobotDriveDelayAndUpdateSafety.vi"("Delay (s)"=0.25, "RobotDriveDevRef"=w522) -> ("RobotDriveDevRef 2"=w521:T2)  [unwired: 8 in, 1 out]
      n294 = case shown="\"R\", Default" w523 {
        tunnel: w521 -> [w527 w580]
        tunnel: w519 -> [w526 _]
        frame "L" {
          n295 = flat-sequence {
            tunnel: w527 -> [w543]
            tunnel: [w537] -> w532
            tunnel: w526 -> [w533]
            tunnel: [w533] -> w524
            tunnel: w532 -> [w552]
            tunnel: [w551] -> w531
            tunnel: [w544] -> w525
            tunnel: w524 -> [w544]
            tunnel: w531 -> [w558]
            tunnel: [w557] -> w530
            tunnel: w525 -> [w554]
            tunnel: w530 -> [w566]
            tunnel: [w569] -> w529
            tunnel: w529 -> [w572]
            tunnel: [w571] -> w528
            tunnel: w528 -> [_]
            frame #0 {
              n296 = global write "Robot Global Data.vi" "Arm Angle to Turn to"(2000.0 ("Intake Speed Override")) -> ()
              n297 = global write "Robot Global Data.vi" "Arm Manual Control"(FALSE ("Arm Manual Control")) -> ()
              n298 = call "Auto Drive XY.vi"("RobotDriveDevRef In"=w543, "Distance (in)"=20.0, "Time to Settle (ms)"=u32 50, "Min Time (ms)"=u32 250, "PID Gains Y"=T8 {"proportional gain (Kc)"=0.03, "integral time (Ti, min)"=0.0, "derivative time (Td, min)"=0.0} ("PID Gains"), "Motor Output Range Y"=cluster{"output high":dbl, "output low":dbl} {"output high"=0.6, "output low"=-0.7} ("Motor Output Range"), "Max Time (ms)"=u32 15000) -> ("RobotDriveDevRef Out"=w537:T2)  [unwired: 8 in]
            }
            frame #1 {
              n299 = call "Auto Drive X.vi"("PID Gains"=T8 {"proportional gain (Kc)"=0.04, "integral time (Ti, min)"=0.0, "derivative time (Td, min)"=0.0}, "Settling Time (ms)"=u32 75, "Max Time (ms)"=u32 15000, "Min Time (ms)"=u32 250, "Angle to Turn (Deg)"=-40.0, "Motor Output Range"=cluster{"output high":dbl, "output low":dbl} {"output high"=0.7, "output low"=-0.7}, "RobotDriveDevRef In"=w552) -> ("RobotDriveDevRef Out"=w551:T2)  [unwired: 4 in]
            }
            frame #2 {
              n300 = global write "Robot Global Data.vi" "Lift Height to rase to (in)"(25.0 ("Intake Speed Override")) -> ()
              n301 = call "Auto Drive XY.vi"("RobotDriveDevRef In"=w558, "Auto"=w554, "Movement"=1.0, "Distance (in)"=120.0, "Time to Settle (ms)"=u32 100, "Min Time (ms)"=u32 250, "PID Gains Y"=T8 {"proportional gain (Kc)"=0.03, "integral time (Ti, min)"=0.0, "derivative time (Td, min)"=0.0} ("PID Gains"), "Motor Output Range Y"=cluster{"output high":dbl, "output low":dbl} {"output high"=0.8, "output low"=-0.7} ("Motor Output Range"), "Max Time (ms)"=u32 2000) -> ("RobotDriveDevRef Out"=w557:T2)  [unwired: 6 in]
            }
            frame #3 {
              w564 = 0.0 ("X axis value")
              n302 = call-poly <vilib>:"WPI_RobotDriveArcadeDrive.vi"("Y axis value"=w564, "X axis value"=w564, "RobotDriveDevRef"=w566) -> ("RobotDriveDevRef"=w565:T2)  [unwired: 6 in, 2 out]
              n303 = global write "Robot Global Data.vi" "Intake Speed Override"(-0.4 ("Intake Speed Override")) -> ()
              n304 = call <vilib>:"WPI_RobotDriveDelayAndUpdateSafety.vi"("Delay (s)"=1.0, "RobotDriveDevRef"=w565) -> ("RobotDriveDevRef 2"=w569:T2)  [unwired: 8 in, 1 out]
            }
            frame #4 {
              n305 = global write "Robot Global Data.vi" "Intake Speed Override"(0.0 ("Intake Speed Override")) -> ()
              n306 = call "Auto Drive Y.vi"("PID Gains"=T8 {"proportional gain (Kc)"=0.03, "integral time (Ti, min)"=0.0, "derivative time (Td, min)"=0.0}, "Max Time (ms)"=u32 15000, "Min Time (ms)"=u32 250, "Time to Settle (ms)"=u32 100, "Distance (in)"=-50.0, "Motor Output Range"=cluster{"output high":dbl, "output low":dbl} {"output high"=0.8, "output low"=-0.7}, "RobotDriveDevRef In"=w572) -> ("RobotDriveDevRef Out"=w571:T2)  [unwired: 4 in]
            }
            frame #5 {
              n307 = global write "Robot Global Data.vi" "Lift Height to rase to (in)"(0.0 ("Intake Speed Override")) -> ()
            }
          }
        }
        frame "R", Default {
          n308 = flat-sequence {
            tunnel: w580 -> [w595]
            tunnel: [w588] -> w585
            tunnel: w585 -> [w603]
            tunnel: [w602] -> w584
            tunnel: w584 -> [w606]
            tunnel: [w605] -> w583
            tunnel: w583 -> [w616]
            tunnel: [w615] -> w582
            tunnel: w582 -> [w619]
            tunnel: [w618] -> w581
            tunnel: w581 -> [_]
            frame #0 {
              n309 = global write "Robot Global Data.vi" "Arm Angle to Turn to"(2000.0 ("Intake Speed Override")) -> ()
              n310 = global write "Robot Global Data.vi" "Arm Manual Control"(FALSE ("Arm Manual Control")) -> ()
              n311 = call "Auto Drive Y.vi"("PID Gains"=T8 {"proportional gain (Kc)"=0.03, "integral time (Ti, min)"=0.0, "derivative time (Td, min)"=0.0}, "Max Time (ms)"=u32 15000, "Min Time (ms)"=u32 250, "Time to Settle (ms)"=u32 50, "Distance (in)"=20.0, "Motor Output Range"=cluster{"output high":dbl, "output low":dbl} {"output high"=0.6, "output low"=-0.7}, "RobotDriveDevRef In"=w595) -> ("RobotDriveDevRef Out"=w588:T2)  [unwired: 4 in]
            }
            frame #1 {
              n312 = call "Auto Drive X.vi"("PID Gains"=T8 {"proportional gain (Kc)"=0.04, "integral time (Ti, min)"=0.0, "derivative time (Td, min)"=0.0}, "Settling Time (ms)"=u32 75, "Max Time (ms)"=u32 15000, "Min Time (ms)"=u32 250, "Angle to Turn (Deg)"=20.0, "Motor Output Range"=cluster{"output high":dbl, "output low":dbl} {"output high"=0.7, "output low"=-0.7}, "RobotDriveDevRef In"=w603) -> ("RobotDriveDevRef Out"=w602:T2)  [unwired: 4 in]
            }
            frame #2 {
              n313 = global write "Robot Global Data.vi" "Lift Height to rase to (in)"(25.0 ("Intake Speed Override")) -> ()
              n314 = call "Auto Drive Y.vi"("PID Gains"=T8 {"proportional gain (Kc)"=0.03, "integral time (Ti, min)"=0.0, "derivative time (Td, min)"=0.0}, "Max Time (ms)"=u32 2000, "Min Time (ms)"=u32 250, "Time to Settle (ms)"=u32 100, "Distance (in)"=100.0, "Motor Output Range"=cluster{"output high":dbl, "output low":dbl} {"output high"=0.8, "output low"=-0.7}, "RobotDriveDevRef In"=w606) -> ("RobotDriveDevRef Out"=w605:T2)  [unwired: 4 in]
            }
            frame #3 {
              n315 = global write "Robot Global Data.vi" "Intake Speed Override"(-0.4 ("Intake Speed Override")) -> ()
              n316 = call <vilib>:"WPI_RobotDriveDelayAndUpdateSafety.vi"("Delay (s)"=1.0, "RobotDriveDevRef"=w616) -> ("RobotDriveDevRef 2"=w615:T2)  [unwired: 8 in, 1 out]
            }
            frame #4 {
              n317 = global write "Robot Global Data.vi" "Intake Speed Override"(0.0 ("Intake Speed Override")) -> ()
              n318 = call "Auto Drive Y.vi"("PID Gains"=T8 {"proportional gain (Kc)"=0.03, "integral time (Ti, min)"=0.0, "derivative time (Td, min)"=0.0}, "Max Time (ms)"=u32 15000, "Min Time (ms)"=u32 250, "Time to Settle (ms)"=u32 100, "Distance (in)"=-50.0, "Motor Output Range"=cluster{"output high":dbl, "output low":dbl} {"output high"=0.8, "output low"=-0.7}, "RobotDriveDevRef In"=w619) -> ("RobotDriveDevRef Out"=w618:T2)  [unwired: 4 in]
            }
            frame #5 {
              n319 = global write "Robot Global Data.vi" "Lift Height to rase to (in)"(0.0 ("Intake Speed Override")) -> ()
            }
          }
        }
      }
    }
    frame "Left Automatic" {
      n320 = call <vilib>:"WPI_RobotDriveDelayAndUpdateSafety.vi"("Delay (s)"=0.25, "RobotDriveDevRef"=w628) -> ("RobotDriveDevRef 2"=w629:T2)  [unwired: 8 in, 1 out]
      n321 = case shown="\"R\", Default" w631 {
        tunnel: w629 -> [w641 w672]
        tunnel: w630 -> [w634 _]
        frame "R", Default {
          n322 = flat-sequence {
            tunnel: w641 -> [w648]
            tunnel: [w646] -> w640
            tunnel: w634 -> [w642]
            tunnel: [w642] -> w633
            tunnel: w640 -> [w650]
            tunnel: [w649] -> w639
            tunnel: w633 -> [w652]
            tunnel: [w652] -> w632
            tunnel: w639 -> [w657]
            tunnel: [w656] -> w638
            tunnel: w632 -> [w654]
            tunnel: w638 -> [w665]
            tunnel: [w664] -> w637
            tunnel: w637 -> [w667]
            tunnel: [w667] -> w636
            tunnel: w636 -> [w670]
            tunnel: [w669] -> w635
            tunnel: w635 -> [w671]
            tunnel: [w671] -> _
            frame #0 {
              n323 = global write "Robot Global Data.vi" "Arm Angle to Turn to"(1250.0 ("Intake Speed Override")) -> ()
              n324 = call "Auto Drive XY.vi"("RobotDriveDevRef In"=w648, "Auto"=w642, "Movement"=1.0, "Distance (in)"=393.0, "Motor Output Range Y"=cluster{"output high":dbl, "output low":dbl} {"output high"=0.8, "output low"=-0.7}) -> ("RobotDriveDevRef Out"=w646:T2)  [unwired: 10 in]
            }
            frame #1 {
              n325 = call <vilib>:"WPI_RobotDriveDelayAndUpdateSafety.vi"("Delay (s)"=0.5, "RobotDriveDevRef"=w650) -> ("RobotDriveDevRef 2"=w649:T2)  [unwired: 8 in, 1 out]
            }
            frame #2 {
              n326 = call "Auto Drive XY.vi"("RobotDriveDevRef In"=w657, "Auto"=w654, "Movement"=2.0, "Distance (in)"=30.0, "Motor Output Range Y"=cluster{"output high":dbl, "output low":dbl} {"output high"=0.7, "output low"=-0.7}) -> ("RobotDriveDevRef Out"=w656:T2)  [unwired: 10 in]
            }
            frame #3 {
              n327 = global write "Robot Global Data.vi" "Intake Speed Override"(0.0 ("Intake Speed Override")) -> ()
              n328 = global write "Robot Global Data.vi" "Lift Height to rase to (in)"(0.0 ("Intake Speed Override")) -> ()
              n329 = global write "Robot Global Data.vi" "Arm Angle to Turn to"(5000.0 ("Intake Speed Override")) -> ()
              n330 = call "Auto Drive Y.vi"("Distance (in)"=-40.0 ("Angle to Turn (Deg)"), "Motor Output Range"=cluster{"output high":dbl, "output low":dbl} {"output high"=0.6, "output low"=-0.6}, "RobotDriveDevRef In"=w665) -> ("RobotDriveDevRef Out"=w664:T2)  [unwired: 8 in]
              n331 = global write "Robot Global Data.vi" "Intake Pistons"(WPI_SolenoidValue."Off" ("Intake Pistons")) -> ()
            }
            frame #4 {
            }
            frame #5 {
              n332 = call "Auto Drive X.vi"("Angle to Turn (Deg)"=180.0, "RobotDriveDevRef In"=w670) -> ("RobotDriveDevRef Out"=w669:T2)  [unwired: 9 in]
            }
            frame #6 {
            }
          }
        }
        frame "L" {
          n333 = flat-sequence {
            tunnel: [w681] -> w676
            tunnel: w672 -> [w679]
            tunnel: w676 -> [w686]
            tunnel: [w685] -> w675
            tunnel: w675 -> [w688]
            tunnel: [w689] -> w674
            tunnel: w674 -> [w694]
            tunnel: [w693] -> w673
            tunnel: w673 -> [_]
            frame #0 {
              n334 = call "Auto Drive XY.vi"("RobotDriveDevRef In"=w679, "Distance (in)"=290.0, "Motor Output Range Y"=cluster{"output high":dbl, "output low":dbl} {"output high"=0.85, "output low"=-0.7}) -> ("RobotDriveDevRef Out"=w681:T2)  [unwired: 12 in]
              n335 = global write "Robot Global Data.vi" "Arm Manual Speed"(0.2 ("Arm Manual Speed")) -> ()
              n336 = global write "Robot Global Data.vi" "Arm Angle to Turn to"(1000.0 ("Intake Speed Override")) -> ()
            }
            frame #1 {
              n337 = global write "Robot Global Data.vi" "Arm Manual Speed"(0.0 ("Arm Manual Speed")) -> ()
              n338 = call "Auto Drive X.vi"("PID Gains"=T8 {"proportional gain (Kc)"=0.05, "integral time (Ti, min)"=0.0, "derivative time (Td, min)"=0.0}, "Angle to Turn (Deg)"=90.0, "RobotDriveDevRef In"=w686) -> ("RobotDriveDevRef Out"=w685:T2)  [unwired: 8 in]
            }
            frame #2 {
              n339 = global write "Robot Global Data.vi" "Intake Speed Override"(0.5 ("Intake Speed Override")) -> ()
              n340 = call "Auto Drive Y.vi"("Distance (in)"=-20.0, "Motor Output Range"=cluster{"output high":dbl, "output low":dbl} {"output high"=0.5, "output low"=-0.5}, "RobotDriveDevRef In"=w688) -> ("RobotDriveDevRef Out"=w689:T2)  [unwired: 8 in]
            }
            frame #3 {
              n341 = global write "Robot Global Data.vi" "Intake Speed Override"(0.0 ("Intake Speed Override")) -> ()
              n342 = global write "Robot Global Data.vi" "Arm Manual Control"(FALSE ("Arm Manual Control")) -> ()
              n343 = global write "Robot Global Data.vi" "Lift Height to rase to (in)"(60.0 ("Intake Speed Override")) -> ()
              n344 = global write "Robot Global Data.vi" "Arm Angle to Turn to"(2500.0 ("Intake Speed Override")) -> ()
              n345 = call <vilib>:"WPI_RobotDriveDelayAndUpdateSafety.vi"("Delay (s)"=1.75, "RobotDriveDevRef"=w694) -> ("RobotDriveDevRef 2"=w693:T2)  [unwired: 8 in, 1 out]
            }
            frame #4 {
              n346 = global write "Robot Global Data.vi" "Intake Speed Override"(-4.0 ("Intake Speed Override")) -> ()
            }
          }
        }
      }
    }
    frame "Right Automatic" {
      n347 = call <vilib>:"WPI_RobotDriveDelayAndUpdateSafety.vi"("Delay (s)"=0.25, "RobotDriveDevRef"=w702) -> ("RobotDriveDevRef 2"=w703:T2)  [unwired: 8 in, 1 out]
      n348 = case shown="\"L\", Default" w705 {
        tunnel: w703 -> [w715 w746]
        tunnel: w704 -> [w708 _]
        frame "L", Default {
          n349 = flat-sequence {
            tunnel: w715 -> [w722]
            tunnel: [w720] -> w714
            tunnel: w708 -> [w716]
            tunnel: [w716] -> w707
            tunnel: w714 -> [w724]
            tunnel: [w723] -> w713
            tunnel: w707 -> [w726]
            tunnel: [w726] -> w706
            tunnel: w713 -> [w731]
            tunnel: [w730] -> w712
            tunnel: w706 -> [w728]
            tunnel: w712 -> [w739]
            tunnel: [w738] -> w711
            tunnel: w711 -> [w741]
            tunnel: [w741] -> w710
            tunnel: w710 -> [w744]
            tunnel: [w743] -> w709
            tunnel: w709 -> [w745]
            tunnel: [w745] -> _
            frame #0 {
              n350 = global write "Robot Global Data.vi" "Arm Angle to Turn to"(1250.0 ("Intake Speed Override")) -> ()
              n351 = call "Auto Drive XY.vi"("RobotDriveDevRef In"=w722, "Auto"=w716, "Movement"=1.0, "Distance (in)"=430.0, "Motor Output Range Y"=cluster{"output high":dbl, "output low":dbl} {"output high"=0.8, "output low"=-0.7}) -> ("RobotDriveDevRef Out"=w720:T2)  [unwired: 10 in]
            }
            frame #1 {
              n352 = call <vilib>:"WPI_RobotDriveDelayAndUpdateSafety.vi"("Delay (s)"=0.5, "RobotDriveDevRef"=w724) -> ("RobotDriveDevRef 2"=w723:T2)  [unwired: 8 in, 1 out]
            }
            frame #2 {
              n353 = call "Auto Drive XY.vi"("RobotDriveDevRef In"=w731, "Auto"=w728, "Movement"=2.0, "Distance (in)"=15.0, "Motor Output Range Y"=cluster{"output high":dbl, "output low":dbl} {"output high"=0.7, "output low"=-0.7}) -> ("RobotDriveDevRef Out"=w730:T2)  [unwired: 10 in]
            }
            frame #3 {
              n354 = global write "Robot Global Data.vi" "Intake Speed Override"(0.0 ("Intake Speed Override")) -> ()
              n355 = global write "Robot Global Data.vi" "Lift Height to rase to (in)"(0.0 ("Intake Speed Override")) -> ()
              n356 = global write "Robot Global Data.vi" "Arm Angle to Turn to"(5000.0 ("Intake Speed Override")) -> ()
              n357 = call "Auto Drive Y.vi"("Distance (in)"=-40.0 ("Angle to Turn (Deg)"), "Motor Output Range"=cluster{"output high":dbl, "output low":dbl} {"output high"=0.6, "output low"=-0.6}, "RobotDriveDevRef In"=w739) -> ("RobotDriveDevRef Out"=w738:T2)  [unwired: 8 in]
              n358 = global write "Robot Global Data.vi" "Intake Pistons"(WPI_SolenoidValue."Off" ("Intake Pistons")) -> ()
            }
            frame #4 {
            }
            frame #5 {
              n359 = call "Auto Drive X.vi"("Angle to Turn (Deg)"=180.0, "RobotDriveDevRef In"=w744) -> ("RobotDriveDevRef Out"=w743:T2)  [unwired: 9 in]
            }
            frame #6 {
            }
          }
        }
        frame "R" {
          n360 = flat-sequence {
            tunnel: [w755] -> w750
            tunnel: w746 -> [w753]
            tunnel: w750 -> [w760]
            tunnel: [w759] -> w749
            tunnel: w749 -> [w762]
            tunnel: [w763] -> w748
            tunnel: w748 -> [w768]
            tunnel: [w767] -> w747
            tunnel: w747 -> [_]
            frame #0 {
              n361 = call "Auto Drive XY.vi"("RobotDriveDevRef In"=w753, "Distance (in)"=300.0, "Motor Output Range Y"=cluster{"output high":dbl, "output low":dbl} {"output high"=0.85, "output low"=-0.7}) -> ("RobotDriveDevRef Out"=w755:T2)  [unwired: 12 in]
              n362 = global write "Robot Global Data.vi" "Arm Manual Speed"(0.2 ("Arm Manual Speed")) -> ()
              n363 = global write "Robot Global Data.vi" "Arm Angle to Turn to"(1000.0 ("Intake Speed Override")) -> ()
            }
            frame #1 {
              n364 = global write "Robot Global Data.vi" "Arm Manual Speed"(0.0 ("Arm Manual Speed")) -> ()
              n365 = call "Auto Drive X.vi"("PID Gains"=T8 {"proportional gain (Kc)"=0.05, "integral time (Ti, min)"=0.0, "derivative time (Td, min)"=0.0}, "Angle to Turn (Deg)"=-90.0, "RobotDriveDevRef In"=w760) -> ("RobotDriveDevRef Out"=w759:T2)  [unwired: 8 in]
            }
            frame #2 {
              n366 = global write "Robot Global Data.vi" "Intake Speed Override"(0.5 ("Intake Speed Override")) -> ()
              n367 = call "Auto Drive Y.vi"("Distance (in)"=0.0, "Motor Output Range"=cluster{"output high":dbl, "output low":dbl} {"output high"=0.5, "output low"=-0.5}, "RobotDriveDevRef In"=w762) -> ("RobotDriveDevRef Out"=w763:T2)  [unwired: 8 in]
            }
            frame #3 {
              n368 = global write "Robot Global Data.vi" "Intake Speed Override"(0.0 ("Intake Speed Override")) -> ()
              n369 = global write "Robot Global Data.vi" "Arm Manual Control"(FALSE ("Arm Manual Control")) -> ()
              n370 = global write "Robot Global Data.vi" "Lift Height to rase to (in)"(60.0 ("Intake Speed Override")) -> ()
              n371 = global write "Robot Global Data.vi" "Arm Angle to Turn to"(2500.0 ("Intake Speed Override")) -> ()
              n372 = call <vilib>:"WPI_RobotDriveDelayAndUpdateSafety.vi"("Delay (s)"=1.75, "RobotDriveDevRef"=w768) -> ("RobotDriveDevRef 2"=w767:T2)  [unwired: 8 in, 1 out]
            }
            frame #4 {
              n373 = global write "Robot Global Data.vi" "Intake Speed Override"(-4.0 ("Intake Speed Override")) -> ()
            }
          }
        }
      }
    }
    frame "Left Automatic 2 Cube Scale" {
      n374 = call <vilib>:"WPI_RobotDriveDelayAndUpdateSafety.vi"("Delay (s)"=0.25, "RobotDriveDevRef"=w778) -> ("RobotDriveDevRef 2"=w777:T2)  [unwired: 8 in, 1 out]
      n375 = case shown="\"R\", Default" w780 {
        tunnel: w777 -> [w782 w819]
        tunnel: w779 -> [_ w818]
        tunnel: w775 -> [w781 _]
        frame "R", Default {
          n376 = case shown="\"L\"" w781 {
            tunnel: w782 -> [w784 w785]
            frame "R", Default {
              n377 = call "Auto Drive Y.vi"("Distance (in)"=-150.0, "RobotDriveDevRef In"=w784) -> ()  [unwired: 9 in, 1 out]
            }
            frame "L" {
              n378 = flat-sequence {
                tunnel: w785 -> [w795]
                tunnel: [w794] -> w790
                tunnel: w790 -> [w798]
                tunnel: [w797] -> w789
                tunnel: w789 -> [w802]
                tunnel: [w801] -> w788
                tunnel: w788 -> [w805]
                tunnel: [w804] -> w787
                tunnel: w787 -> [w809]
                tunnel: [w808] -> w786
                tunnel: [w812] -> _
                tunnel: w786 -> [w812]
                frame #0 {
                  n379 = global write "Robot Global Data.vi" "Lift Height to rase to (in)"(30.0 ("Lift Height to rase to (in)")) -> ()
                  n380 = call "Auto Drive Y.vi"("Distance (in)"=-150.0, "RobotDriveDevRef In"=w795) -> ("RobotDriveDevRef Out"=w794:T2)  [unwired: 9 in]
                  n381 = global write "Robot Global Data.vi" "Arm Angle to Turn to"(2000.0 ("Lift Height to rase to (in)")) -> ()
                }
                frame #1 {
                  n382 = call "Auto Drive X.vi"("Angle to Turn (Deg)"=-90.0, "RobotDriveDevRef In"=w798) -> ("RobotDriveDevRef Out"=w797:T2)  [unwired: 9 in]
                }
                frame #2 {
                  n383 = call "Auto Drive Y.vi"("Max Time (ms)"=u32 2000, "Distance (in)"=20.0, "RobotDriveDevRef In"=w802) -> ("RobotDriveDevRef Out"=w801:T2)  [unwired: 8 in]
                }
                frame #3 {
                  n384 = call <vilib>:"WPI_RobotDriveDelayAndUpdateSafety.vi"("Delay (s)"=1.0, "RobotDriveDevRef"=w805) -> ("RobotDriveDevRef 2"=w804:T2)  [unwired: 8 in, 1 out]
                  n385 = global write "Robot Global Data.vi" "Intake Speed Override"(-0.5 ("Lift Height to rase to (in)")) -> ()
                }
                frame #4 {
                  n386 = call "Auto Drive Y.vi"("Distance (in)"=-30.0, "RobotDriveDevRef In"=w809) -> ("RobotDriveDevRef Out"=w808:T2)  [unwired: 9 in]
                }
                frame #5 {
                  n387 = global write "Robot Global Data.vi" "Lift Height to rase to (in)"(0.0 ("Lift Height to rase to (in)")) -> ()
                  n388 = global write "Robot Global Data.vi" "Arm Angle to Turn to"(0.0 ("Lift Height to rase to (in)")) -> ()
                }
              }
            }
          }
        }
        frame "L" {
          n389 = flat-sequence {
            tunnel: w819 -> [w826]
            tunnel: w818 -> [w822]
            tunnel: [w823] -> w817
            tunnel: [w822] -> w816
            tunnel: w817 -> [w837]
            tunnel: w816 -> [w830]
            tunnel: [w831] -> w815
            tunnel: [w830] -> w814
            tunnel: w815 -> [w846]
            tunnel: w814 -> [w845]
            tunnel: [w838] -> w813
            tunnel: w813 -> [w852]
            tunnel: [w851] -> _
            frame #0 {
              # "-258"
              n390 = call "Auto Drive XY.vi"("RobotDriveDevRef In"=w826, "Auto"=w822, "Movement"=1.0, "PID Gains X"=T8 {"proportional gain (Kc)"=0.1, "integral time (Ti, min)"=0.0, "derivative time (Td, min)"=0.0}, "Distance (in)"=-265.0, "Min Time (ms)"=u32 3000) -> ("RobotDriveDevRef Out"=w823:T2)  [unwired: 9 in]
            }
            frame #1 {
              # "-90"
              n391 = global write "Robot Global Data.vi" "Lift Height to rase to (in)"(0.0 ("Intake Speed Override")) -> ()
              n392 = global write "Robot Global Data.vi" "Arm Angle to Turn to"(0.0 ("Intake Speed Override")) -> ()
              n393 = global write "Robot Global Data.vi" "Intake Speed Override"(-1.0 ("Intake Speed Override")) -> ()
              n394 = global write "Robot Global Data.vi" "Arm Auto Min Speed"(TRUE ("Arm Auto Min Speed")) -> ()
              n395 = call "Auto Drive XY.vi"("RobotDriveDevRef In"=w837, "Angle Offset"=-115.0, "Auto"=w830, "Movement"=2.0, "Distance (in)"=150.0, "Min Time (ms)"=u32 1000) -> ("RobotDriveDevRef Out"=w831:T2)  [unwired: 9 in]
            }
            frame #2 {
              # "30"
              n396 = global write "Robot Global Data.vi" "Lift Height to rase to (in)"(60.0 ("Intake Speed Override")) -> ()
              n397 = global write "Robot Global Data.vi" "Arm Angle to Turn to"(6000.0 ("Intake Speed Override")) -> ()
              n398 = global write "Robot Global Data.vi" "Intake Pistons"(WPI_SolenoidValue."Off" ("Intake Pistons")) -> ()
              n399 = call "Auto Drive XY.vi"("RobotDriveDevRef In"=w846, "Angle Offset"=15.0, "Auto"=w845, "Movement"=3.0, "Distance (in)"=-56.0) -> ("RobotDriveDevRef Out"=w838:T2)  [unwired: 10 in]
            }
            frame #3 {
              n400 = global write "Robot Global Data.vi" "Lift Height to rase to (in)"(0.0 ("Intake Speed Override")) -> ()
              n401 = global write "Robot Global Data.vi" "Arm Angle to Turn to"(0.0 ("Intake Speed Override")) -> ()
              n402 = call "Auto Drive XY.vi"("RobotDriveDevRef In"=w852, "Distance (in)"=30.0) -> ("RobotDriveDevRef Out"=w851:T2)  [unwired: 13 in]
              n403 = global write "Robot Global Data.vi" "Intake Pistons"(WPI_SolenoidValue."Off" ("Intake Pistons")) -> ()
            }
          }
        }
      }
    }
    frame "Left Automatic New", Default {
      # "LEFT"
      # "-1 -  Drive Past Baseline, something went wrong\n1   - Close Switch, Close Scale\n2   - Close Switch, Close Switch\n3   - Far Switch,      Far Scale\n4   - Far Switch,      Far Switch\n5   - Drive Forward and turn\n6   - Close Scale,    Close Scale\n7   - Close Switch\n8   - Close Scale\n9   - Far Scale,         Far Scale\n10 - Far Scale\n11 - Far Switch\n12 - Close Switch, Far Scale"
      n404 = global read "Robot Global Data.vi" "Place From Null"() -> (w857:bool)
      n405 = call <vilib>:"WPI_RobotDriveDelayAndUpdateSafety.vi"("Delay (s)"=0.125, "RobotDriveDevRef"=w859) -> ("RobotDriveDevRef 2"=w854:T2)  [unwired: 8 in, 1 out]
      n406 = case shown="False" w857 {
        tunnel: [w861 w983] -> w856
        tunnel: [_ 0] -> w855
        tunnel: w854 -> [w860 w981]
        tunnel: [w860 w981] -> w853
        frame False {
          # "Normal"
          # "1   - Close Switch, Close Scale\n2   - Close Switch, Close Switch\n3   - Far Switch,      Far Scale\n4   - Far Switch,      Far Switch\n5   - Drive Forward and turn\n6   - Close Scale,    Close Scale\n7   - Close Switch\n8   - Close Scale\n9   - Far Scale,         Far Scale\n10 - Far Scale\n11 - Far Switch\n12 - Close Switch, Far Scale"
          n407 = global read "Robot Global Data.vi" "Do Not Cross Field"() -> (w864:bool)
          n408 = global read "Robot Global Data.vi" "Attempt 2 Cube"() -> (w865:bool)
          n409 = global read "Robot Global Data.vi" "Switch Position"() -> (w863:string)
          n410 = global read "Robot Global Data.vi" "Scale Position"() -> (w862:string)
          n411 = global read "Robot Global Data.vi" "Focus Switch"() -> (w866:bool)
          n412 = case shown="True" w866 {
            tunnel: w865 -> [w871 w928]
            tunnel: w864 -> [w870 w927]
            tunnel: w863 -> [w869 w926]
            tunnel: w862 -> [w868 w925]
            tunnel: [w867 w924] -> w861
            frame True {
              n413 = case shown="False" w871 {
                tunnel: w870 -> [w875 w901]
                tunnel: w869 -> [w874 w900]
                tunnel: w868 -> [w873 w899]
                tunnel: [w872 w898] -> w867
                frame True {
                  n414 = case shown="False" w875 {
                    tunnel: w874 -> [w878 w889]
                    tunnel: w873 -> [w877 w888]
                    tunnel: [w876 w887] -> w872
                    frame True {
                      n415 = case shown="\"L\"" w878 {
                        tunnel: w877 -> [w880 w884]
                        tunnel: [w879 w883] -> w876
                        frame "L" {
                          n416 = case shown="\"R\", Default" w880 {
                            tunnel: [7 1] -> w879
                            frame "R", Default {
                              # "2"
                            }
                            frame "L" {
                            }
                          }
                        }
                        frame "R", Default {
                          n417 = case shown="\"L\"" w884 {
                            tunnel: [5 6] -> w883
                            frame "R", Default {
                            }
                            frame "L" {
                            }
                          }
                        }
                      }
                    }
                    frame False {
                      n418 = case shown="\"R\", Default" w889 {
                        tunnel: w888 -> [w891 w895]
                        tunnel: [w890 w894] -> w887
                        frame "L" {
                          n419 = case shown="\"L\"" w891 {
                            tunnel: [12 1] -> w890
                            frame "R", Default {
                            }
                            frame "L" {
                            }
                          }
                        }
                        frame "R", Default {
                          n420 = case shown="\"L\"" w895 {
                            tunnel: [3 11] -> w894
                            frame "R", Default {
                            }
                            frame "L" {
                              # "4"
                            }
                          }
                        }
                      }
                    }
                  }
                }
                frame False {
                  n421 = case shown="False" w901 {
                    tunnel: w900 -> [w904 w915]
                    tunnel: w899 -> [w903 w914]
                    tunnel: [w902 w913] -> w898
                    frame True {
                      n422 = case shown="\"L\"" w904 {
                        tunnel: w903 -> [w906 w910]
                        tunnel: [w905 w909] -> w902
                        frame "L" {
                          n423 = case shown="\"R\", Default" w906 {
                            tunnel: [7 7] -> w905
                            frame "R", Default {
                            }
                            frame "L" {
                            }
                          }
                        }
                        frame "R", Default {
                          n424 = case shown="\"R\", Default" w910 {
                            tunnel: [5 8] -> w909
                            frame "R", Default {
                            }
                            frame "L" {
                            }
                          }
                        }
                      }
                    }
                    frame False {
                      n425 = case shown="\"R\", Default" w915 {
                        tunnel: w914 -> [w917 w921]
                        tunnel: [w916 w920] -> w913
                        frame "L" {
                          n426 = case shown="\"L\"" w917 {
                            tunnel: [7 7] -> w916
                            frame "R", Default {
                            }
                            frame "L" {
                            }
                          }
                        }
                        frame "R", Default {
                          n427 = case shown="\"R\", Default" w921 {
                            tunnel: [11 11] -> w920
                            frame "R", Default {
                            }
                            frame "L" {
                            }
                          }
                        }
                      }
                    }
                  }
                }
              }
            }
            frame False {
              n428 = case shown="False" w928 {
                tunnel: w927 -> [w932 w958]
                tunnel: w926 -> [w931 w957]
                tunnel: w925 -> [w930 w956]
                tunnel: [w929 w955] -> w924
                frame True {
                  n429 = case shown="False" w932 {
                    tunnel: w931 -> [w935 w946]
                    tunnel: w930 -> [w934 w945]
                    tunnel: [w933 w944] -> w929
                    frame True {
                      n430 = case shown="\"L\"" w935 {
                        tunnel: w934 -> [w937 w941]
                        tunnel: [w936 w940] -> w933
                        frame "L" {
                          n431 = case shown="\"R\", Default" w937 {
                            tunnel: [7 6] -> w936
                            frame "R", Default {
                              # "2"
                            }
                            frame "L" {
                            }
                          }
                        }
                        frame "R", Default {
                          n432 = case shown="\"L\"" w941 {
                            tunnel: [5 6] -> w940
                            frame "R", Default {
                            }
                            frame "L" {
                            }
                          }
                        }
                      }
                    }
                    frame False {
                      n433 = case shown="\"R\", Default" w946 {
                        tunnel: w945 -> [w948 w952]
                        tunnel: [w947 w951] -> w944
                        frame "L" {
                          n434 = case shown="\"R\", Default" w948 {
                            tunnel: [9 6] -> w947
                            frame "R", Default {
                            }
                            frame "L" {
                            }
                          }
                        }
                        frame "R", Default {
                          n435 = case shown="\"R\", Default" w952 {
                            tunnel: [9 6] -> w951
                            frame "R", Default {
                            }
                            frame "L" {
                            }
                          }
                        }
                      }
                    }
                  }
                }
                frame False {
                  n436 = case shown="False" w958 {
                    tunnel: w957 -> [w961 w972]
                    tunnel: w956 -> [w960 w971]
                    tunnel: [w959 w970] -> w955
                    frame True {
                      n437 = case shown="\"R\", Default" w961 {
                        tunnel: w960 -> [w963 w967]
                        tunnel: [w962 w966] -> w959
                        frame "L" {
                          n438 = case shown="\"L\"" w963 {
                            tunnel: [7 8] -> w962
                            frame "R", Default {
                            }
                            frame "L" {
                            }
                          }
                        }
                        frame "R", Default {
                          n439 = case shown="\"L\"" w967 {
                            tunnel: [5 8] -> w966
                            frame "R", Default {
                            }
                            frame "L" {
                            }
                          }
                        }
                      }
                    }
                    frame False {
                      n440 = case shown="\"L\"" w972 {
                        tunnel: w971 -> [w974 w978]
                        tunnel: [w973 w977] -> w970
                        frame "L" {
                          n441 = case shown="\"R\", Default" w974 {
                            tunnel: [10 8] -> w973
                            frame "R", Default {
                            }
                            frame "L" {
                            }
                          }
                        }
                        frame "R", Default {
                          n442 = case shown="\"R\", Default" w978 {
                            tunnel: [10 8] -> w977
                            frame "R", Default {
                            }
                            frame "L" {
                            }
                          }
                        }
                      }
                    }
                  }
                }
              }
            }
          }
          n443 = global write "Robot Global Data.vi" "Auto Running"(w861) -> ()
        }
        frame True {
          # "PLACE FROM NULL"
          # "1   - Close Switch, Close Scale\n2   - Close Switch, Close Switch\n3   - Far Switch,      Far Scale\n4   - Far Switch,      Far Switch\n5   - Drive Forward and turn\n6   - Close Scale,    Close Scale\n7   - Close Switch\n8   - Close Scale\n9   - Far Scale,         Far Scale\n10 - Far Scale\n11 - Far Switch\n12 - Close Switch, Far Scale\n13 - Place from null"
          n444 = global read "Robot Global Data.vi" "Switch Position"() -> (w986:string)
          n445 = global read "Robot Global Data.vi" "Scale Position"() -> (w985:string)
          n446 = global read "Robot Global Data.vi" "Focus Switch"() -> (w984:bool)
          n447 = case shown="True" w984 {
            tunnel: w986 -> [w989 w1000]
            tunnel: w985 -> [w988 w999]
            tunnel: [w987 w998] -> w983
            frame False {
              n448 = case shown="\"L\"" w989 {
                tunnel: w988 -> [w991 w995]
                tunnel: [w990 w994] -> w987
                frame "L" {
                  n449 = case shown="\"L\"" w991 {
                    tunnel: [7 13] -> w990
                    frame "R", Default {
                    }
                    frame "L" {
                    }
                  }
                }
                frame "R", Default {
                  n450 = case shown="\"L\"" w995 {
                    tunnel: [5 13] -> w994
                    frame "R", Default {
                    }
                    frame "L" {
                    }
                  }
                }
              }
            }
            frame True {
              n451 = case shown="\"R\", Default" w1000 {
                tunnel: w999 -> [w1002 w1006]
                tunnel: [w1001 w1005] -> w998
                frame "L" {
                  n452 = case shown="\"L\"" w1002 {
                    tunnel: [7 7] -> w1001
                    frame "R", Default {
                    }
                    frame "L" {
                    }
                  }
                }
                frame "R", Default {
                  n453 = case shown="\"R\", Default" w1006 {
                    tunnel: [5 13] -> w1005
                    frame "R", Default {
                    }
                    frame "L" {
                    }
                  }
                }
              }
            }
          }
          n454 = global write "Robot Global Data.vi" "Auto Running"(w983) -> ()
        }
      }
      n455 = case shown="1" w856 {
        tunnel: w853 -> [w1010 w1014 w1045 w1084 w1111 w1138 w1147 w1180 w1202 w1217 w1250 w1262 w1282 w1306]
        tunnel: w855 -> [_ _ _ _ _ _ _ _ _ _ _ _ _ _]
        frame -1, Default {
          n456 = call "Auto Drive XY Left Automatic.vi"("RobotDriveDevRef In"=w1010, "Distance (in)"=-150.0) -> ()  [unwired: 13 in, 1 out]
        }
        frame 1 {
          n457 = flat-sequence {
            tunnel: w1014 -> [w1020]
            tunnel: [w1017] -> w1013
            tunnel: w1013 -> [w1026]
            tunnel: [w1022] -> w1012
            tunnel: w1012 -> [w1031]
            tunnel: [w1030] -> w1011
            tunnel: w1011 -> [w1038]
            frame #0 {
              n458 = call "Auto Drive XY Left Automatic.vi"("RobotDriveDevRef In"=w1020, "Movement"=1.0, "Distance (in)"=-180.0, "Time to Settle (ms)"=u32 10, "Motor Output Range Y"=cluster{"output high":dbl, "output low":dbl} {"output high"=0.7, "output low"=-0.75}) -> ("RobotDriveDevRef Out"=w1017:T2)  [unwired: 10 in]
            }
            frame #1 {
              n459 = global write "Robot Global Data.vi" "Intake Speed Override"(-0.5 ("Intake Speed Override")) -> ()
              n460 = call "Auto Drive XY Left Automatic.vi"("RobotDriveDevRef In"=w1026, "Movement"=2.0, "Distance (in)"=300.0, "Time to Settle (ms)"=u32 100) -> ("RobotDriveDevRef Out"=w1022:T2)  [unwired: 11 in]
            }
            frame #2 {
              n461 = global write "Robot Global Data.vi" "Intake Pistons"(WPI_SolenoidValue."Off" ("Intake Pistons")) -> ()
              n462 = call "Auto Drive XY Left Automatic.vi"("RobotDriveDevRef In"=w1031, "Movement"=3.0, "Distance (in)"=-55.0, "Time to Settle (ms)"=u32 500, "Motor Output Range Y"=cluster{"output high":dbl, "output low":dbl} {"output high"=0.7, "output low"=-0.8}) -> ("RobotDriveDevRef Out"=w1030:T2)  [unwired: 10 in]
            }
            frame #3 {
              n463 = global write "Robot Global Data.vi" "Intake Speed Override"(-0.3 ("Arm Angle to Turn to")) -> ()
              n464 = call "Auto Drive XY Left Automatic.vi"("RobotDriveDevRef In"=w1038, "Distance (in)"=20.0) -> ()  [unwired: 13 in, 1 out]
              n465 = global write "Robot Global Data.vi" "Lift Height to rase to (in)"(0.0 ("Arm Angle to Turn to")) -> ()
              n466 = global write "Robot Global Data.vi" "Arm Angle to Turn to"(0.0 ("Arm Angle to Turn to")) -> ()
            }
          }
        }
        frame 2 {
          n467 = flat-sequence {
            tunnel: w1045 -> [w1051]
            tunnel: [w1048] -> w1044
            tunnel: w1044 -> [w1057]
            tunnel: [w1053] -> w1043
            tunnel: w1043 -> [w1063]
            tunnel: [w1062] -> w1041
            tunnel: w1041 -> [w1067]
            tunnel: [w1066] -> w1040
            tunnel: w1040 -> [w1069]
            tunnel: [w1068] -> w1039
            tunnel: w1039 -> [w1072]
            tunnel: [w1073] -> w1042
            tunnel: w1042 -> [w1078]
            frame #0 {
              n468 = call "Auto Drive XY Left Automatic.vi"("RobotDriveDevRef In"=w1051, "Movement"=1.0, "Distance (in)"=-170.0, "Time to Settle (ms)"=u32 10, "Motor Output Range Y"=cluster{"output high":dbl, "output low":dbl} {"output high"=0.7, "output low"=-0.75}) -> ("RobotDriveDevRef Out"=w1048:T2)  [unwired: 10 in]
            }
            frame #1 {
              n469 = global write "Robot Global Data.vi" "Intake Speed Override"(-0.5 ("Intake Speed Override")) -> ()
              n470 = call "Auto Drive XY Left Automatic.vi"("RobotDriveDevRef In"=w1057, "Movement"=2.0, "Distance (in)"=300.0, "Time to Settle (ms)"=u32 100) -> ("RobotDriveDevRef Out"=w1053:T2)  [unwired: 11 in]
            }
            frame #2 {
              n471 = call <vilib>:"WPI_RobotDriveDelayAndUpdateSafety.vi"("Delay (s)"=1.0, "RobotDriveDevRef"=w1063) -> ("RobotDriveDevRef 2"=w1062:T2)  [unwired: 8 in, 1 out]
              n472 = global write "Robot Global Data.vi" "Lift Height to rase to (in)"(40.0 ("Arm Angle to Turn to")) -> ()
              n473 = global write "Robot Global Data.vi" "Arm Angle to Turn to"(500.0 ("Arm Angle to Turn to")) -> ()
              n474 = global write "Robot Global Data.vi" "Intake Pistons"(WPI_SolenoidValue."Off" ("Intake Pistons")) -> ()
            }
            frame #3 {
              n475 = call-poly <vilib>:"WPI_RobotDriveArcadeDrive.vi"("Y axis value"=0.6, "X axis value"=0.0, "RobotDriveDevRef"=w1067) -> ("RobotDriveDevRef"=w1066:T2)  [unwired: 6 in, 2 out]
            }
            frame #4 {
              n476 = call <vilib>:"WPI_RobotDriveDelayAndUpdateSafety.vi"("Delay (s)"=0.25, "RobotDriveDevRef"=w1069) -> ("RobotDriveDevRef 2"=w1068:T2)  [unwired: 8 in, 1 out]
            }
            frame #5 {
              n477 = call <vilib>:"WPI_RobotDriveDelayAndUpdateSafety.vi"("Delay (s)"=1.0, "RobotDriveDevRef"=w1072) -> ("RobotDriveDevRef 2"=w1073:T2)  [unwired: 8 in, 1 out]
              n478 = global write "Robot Global Data.vi" "Intake Speed Override"(-0.8 ("Arm Angle to Turn to")) -> ()
            }
            frame #6 {
              n479 = global write "Robot Global Data.vi" "Intake Speed Override"(0.0 ("Intake Speed Override")) -> ()
              n480 = global write "Robot Global Data.vi" "Lift Height to rase to (in)"(0.0 ("Arm Angle to Turn to")) -> ()
              n481 = global write "Robot Global Data.vi" "Arm Angle to Turn to"(0.0 ("Arm Angle to Turn to")) -> ()
              n482 = call "Auto Drive XY Left Automatic.vi"("RobotDriveDevRef In"=w1078, "Movement"=3.0, "Distance (in)"=-30.0) -> ()  [unwired: 12 in, 1 out]
            }
          }
        }
        frame 3 {
          n483 = flat-sequence {
            tunnel: w1084 -> [w1089]
            tunnel: [w1086] -> w1083
            tunnel: w1083 -> [w1096]
            tunnel: [w1093] -> w1082
            tunnel: w1082 -> [w1099]
            tunnel: [w1098] -> w1081
            tunnel: w1081 -> [w1105]
            frame #0 {
              n484 = call "Auto Drive XY Left Automatic.vi"("RobotDriveDevRef In"=w1089, "Movement"=1.0, "Distance (in)"=-600.0, "Motor Output Range Y"=cluster{"output high":dbl, "output low":dbl} {"output high"=0.85, "output low"=-0.95}) -> ("RobotDriveDevRef Out"=w1086:T2)  [unwired: 11 in]
            }
            frame #1 {
              n485 = global write "Robot Global Data.vi" "Intake Speed Override"(-0.5 ("Arm Angle to Turn to")) -> ()
              n486 = call "Auto Drive XY Left Automatic.vi"("RobotDriveDevRef In"=w1096, "Movement"=2.0, "Distance (in)"=150.0, "Time to Settle (ms)"=u32 150, "Motor Output Range Y"=cluster{"output high":dbl, "output low":dbl} {"output high"=0.75, "output low"=-0.7}) -> ("RobotDriveDevRef Out"=w1093:T2)  [unwired: 10 in]
            }
            frame #2 {
              n487 = call "Auto Drive XY Left Automatic.vi"("RobotDriveDevRef In"=w1099, "Movement"=3.0, "Distance (in)"=-60.0) -> ("RobotDriveDevRef Out"=w1098:T2)  [unwired: 12 in]
              n488 = global write "Robot Global Data.vi" "Intake Pistons"(WPI_SolenoidValue."Off" ("Intake Pistons")) -> ()
            }
            frame #3 {
              n489 = call "Auto Drive XY Left Automatic.vi"("RobotDriveDevRef In"=w1105, "Distance (in)"=25.0) -> ()  [unwired: 13 in, 1 out]
              n490 = global write "Robot Global Data.vi" "Intake Speed Override"(0.0 ("Arm Angle to Turn to")) -> ()
              n491 = global write "Robot Global Data.vi" "Lift Height to rase to (in)"(0.0 ("Arm Angle to Turn to")) -> ()
              n492 = global write "Robot Global Data.vi" "Arm Angle to Turn to"(0.0 ("Arm Angle to Turn to")) -> ()
            }
          }
        }
        frame 4 {
          n493 = flat-sequence {
            tunnel: w1111 -> [w1116]
            tunnel: [w1113] -> w1110
            tunnel: w1110 -> [w1123]
            tunnel: [w1120] -> w1109
            tunnel: w1109 -> [w1129]
            tunnel: [w1128] -> w1108
            tunnel: w1108 -> [w1133]
            tunnel: [w1132] -> w1107
            tunnel: w1107 -> [w1136]
            frame #0 {
              n494 = call "Auto Drive XY Left Automatic.vi"("RobotDriveDevRef In"=w1116, "Movement"=1.0, "Distance (in)"=-600.0, "Motor Output Range Y"=cluster{"output high":dbl, "output low":dbl} {"output high"=0.85, "output low"=-0.95}) -> ("RobotDriveDevRef Out"=w1113:T2)  [unwired: 11 in]
            }
            frame #1 {
              n495 = global write "Robot Global Data.vi" "Intake Speed Override"(-0.5 ("Arm Angle to Turn to")) -> ()
              n496 = call "Auto Drive XY Left Automatic.vi"("RobotDriveDevRef In"=w1123, "Movement"=2.0, "Distance (in)"=150.0, "Time to Settle (ms)"=u32 150, "Motor Output Range Y"=cluster{"output high":dbl, "output low":dbl} {"output high"=0.75, "output low"=-0.7}) -> ("RobotDriveDevRef Out"=w1120:T2)  [unwired: 10 in]
            }
            frame #2 {
              n497 = call <vilib>:"WPI_RobotDriveDelayAndUpdateSafety.vi"("Delay (s)"=0.5, "RobotDriveDevRef"=w1129) -> ("RobotDriveDevRef 2"=w1128:T2)  [unwired: 8 in, 1 out]
              n498 = global write "Robot Global Data.vi" "Lift Height to rase to (in)"(30.0 ("Arm Angle to Turn to")) -> ()
              n499 = global write "Robot Global Data.vi" "Arm Angle to Turn to"(500.0 ("Arm Angle to Turn to")) -> ()
              n500 = global write "Robot Global Data.vi" "Intake Pistons"(WPI_SolenoidValue."Off" ("Intake Pistons")) -> ()
            }
            frame #3 {
              n501 = call <vilib>:"WPI_RobotDriveDelayAndUpdateSafety.vi"("Delay (s)"=1.0, "RobotDriveDevRef"=w1133) -> ("RobotDriveDevRef 2"=w1132:T2)  [unwired: 8 in, 1 out]
              n502 = global write "Robot Global Data.vi" "Intake Speed Override"(1.0 ("Arm Angle to Turn to")) -> ()
            }
            frame #4 {
              n503 = global write "Robot Global Data.vi" "Arm Angle to Turn to"(0.0 ("Arm Angle to Turn to")) -> ()
              n504 = global write "Robot Global Data.vi" "Lift Height to rase to (in)"(0.0 ("Arm Angle to Turn to")) -> ()
              n505 = call "Auto Drive XY Left Automatic.vi"("RobotDriveDevRef In"=w1136, "Distance (in)"=30.0) -> ()  [unwired: 13 in, 1 out]
            }
          }
        }
        frame 5 {
          n506 = flat-sequence {
            tunnel: w1138 -> [w1141]
            frame #0 {
              n507 = call "Auto Drive XY Left Automatic.vi"("RobotDriveDevRef In"=w1141, "Movement"=1.0, "Distance (in)"=-250.0) -> ()  [unwired: 12 in, 1 out]
            }
            frame #1 {
              n508 = global write "Robot Global Data.vi" "Lift Height to rase to (in)"(0.0 ("Arm Angle to Turn to")) -> ()
              n509 = global write "Robot Global Data.vi" "Arm Angle to Turn to"(0.0 ("Arm Angle to Turn to")) -> ()
            }
          }
        }
        frame 6 {
          n510 = flat-sequence {
            tunnel: w1147 -> [w1153]
            tunnel: [w1150] -> w1146
            tunnel: w1146 -> [w1164]
            tunnel: [w1159] -> w1145
            tunnel: w1145 -> [w1170]
            tunnel: [w1165] -> w1144
            tunnel: w1144 -> [w1177]
            frame #0 {
              n511 = call "Auto Drive XY Left Automatic.vi"("RobotDriveDevRef In"=w1153, "Movement"=1.0, "Motor Output Range X"=cluster{"output high":dbl, "output low":dbl} {"output high"=0.8, "output low"=-0.8}, "Distance (in)"=-273.0, "Motor Output Range Y"=cluster{"output high":dbl, "output low":dbl} {"output high"=0.7, "output low"=-0.8}) -> ("RobotDriveDevRef Out"=w1150:T2)  [unwired: 10 in]
            }
            frame #1 {
              n512 = global write "Robot Global Data.vi" "Lift Height to rase to (in)"(0.0 ("Arm Angle to Turn to")) -> ()
              n513 = global write "Robot Global Data.vi" "Intake Speed Override"(-0.5 ("Arm Angle to Turn to")) -> ()
              n514 = global write "Robot Global Data.vi" "Arm Angle to Turn to"(0.0 ("Arm Angle to Turn to")) -> ()
              n515 = global write "Robot Global Data.vi" "Auto Arm Fast"(TRUE ("Lift Down Fast")) -> ()
              n516 = global write "Robot Global Data.vi" "Lift Down Fast"(TRUE ("Lift Down Fast")) -> ()
              n517 = call "Auto Drive XY Left Automatic.vi"("RobotDriveDevRef In"=w1164, "Angle Offset"=-10.0, "Movement"=2.0, "Distance (in)"=77.0, "Motor Output Range Y"=cluster{"output high":dbl, "output low":dbl} {"output high"=0.6, "output low"=-0.7}) -> ("RobotDriveDevRef Out"=w1159:T2)  [unwired: 10 in]
            }
            frame #2 {
              n518 = global write "Robot Global Data.vi" "Auto Arm Fast"(FALSE ("Lift Down Fast")) -> ()
              n519 = global write "Robot Global Data.vi" "Lift Down Fast"(FALSE ("Lift Down Fast")) -> ()
              n520 = call "Auto Drive XY Left Automatic.vi"("RobotDriveDevRef In"=w1170, "Movement"=3.0, "Distance (in)"=-65.0) -> ("RobotDriveDevRef Out"=w1165:T2)  [unwired: 12 in]
              n521 = global write "Robot Global Data.vi" "Intake Pistons"(WPI_SolenoidValue."Off" ("Intake Pistons")) -> ()
            }
            frame #3 {
              n522 = global write "Robot Global Data.vi" "Intake Speed Override"(-0.3 ("Intake Speed Override")) -> ()
              n523 = global write "Robot Global Data.vi" "Intake Pistons"(WPI_SolenoidValue."Off" ("Intake Pistons")) -> ()
              n524 = call "Auto Drive XY Left Automatic.vi"("RobotDriveDevRef In"=w1177, "Movement"=4.0, "Distance (in)"=70.0, "Motor Output Range Y"=cluster{"output high":dbl, "output low":dbl} {"output high"=0.6, "output low"=-0.6}) -> ()  [unwired: 11 in, 1 out]
            }
          }
        }
        frame 7 {
          n525 = flat-sequence {
            tunnel: [w1183] -> w1181
            tunnel: w1180 -> [w1182]
            tunnel: w1181 -> [w1189]
            tunnel: [w1188] -> w1179
            tunnel: w1179 -> [w1198]
            tunnel: [w1197] -> w1178
            tunnel: [w1200] -> _
            tunnel: w1178 -> [w1200]
            frame #0 {
              n526 = call "Auto Drive XY Left Automatic.vi"("RobotDriveDevRef In"=w1182, "Movement"=1.0, "Distance (in)"=-170.0, "Time to Settle (ms)"=u32 10, "Motor Output Range Y"=cluster{"output high":dbl, "output low":dbl} {"output high"=0.7, "output low"=-0.75}) -> ("RobotDriveDevRef Out"=w1183:T2)  [unwired: 10 in]
            }
            frame #1 {
              n527 = global write "Robot Global Data.vi" "Intake Speed Override"(-0.5 ("Intake Speed Override")) -> ()
              n528 = call "Auto Drive XY Left Automatic.vi"("RobotDriveDevRef In"=w1189, "Movement"=2.0, "Distance (in)"=300.0, "Time to Settle (ms)"=u32 100) -> ("RobotDriveDevRef Out"=w1188:T2)  [unwired: 11 in]
            }
            frame #2 {
              n529 = call "Auto Drive XY Left Automatic.vi"("RobotDriveDevRef In"=w1198, "Angle Offset"=-90.0, "Distance (in)"=-70.0) -> ("RobotDriveDevRef Out"=w1197:T2)  [unwired: 12 in]
              n530 = global write "Robot Global Data.vi" "Intake Pistons"(WPI_SolenoidValue."Off" ("Intake Pistons")) -> ()
            }
            frame #3 {
              n531 = global write "Robot Global Data.vi" "Intake Speed Override"(0.0 ("Intake Speed Override")) -> ()
            }
          }
        }
        frame 8 {
          n532 = flat-sequence {
            tunnel: w1202 -> [w1203]
            tunnel: [w1204] -> w1201
            tunnel: w1201 -> [w1209]
            frame #0 {
              n533 = call "Auto Drive XY Left Automatic.vi"("RobotDriveDevRef In"=w1203, "Movement"=1.0, "Motor Output Range X"=cluster{"output high":dbl, "output low":dbl} {"output high"=0.8, "output low"=-0.8}, "Distance (in)"=-273.0, "Motor Output Range Y"=cluster{"output high":dbl, "output low":dbl} {"output high"=0.7, "output low"=-0.8}) -> ("RobotDriveDevRef Out"=w1204:T2)  [unwired: 10 in]
            }
            frame #1 {
              n534 = global write "Robot Global Data.vi" "Arm Angle to Turn to"(0.0 ("Arm Angle to Turn to")) -> ()
              n535 = global write "Robot Global Data.vi" "Lift Height to rase to (in)"(0.0 ("Arm Angle to Turn to")) -> ()
              n536 = call "Auto Drive XY Left Automatic.vi"("RobotDriveDevRef In"=w1209, "Distance (in)"=30.0) -> ()  [unwired: 13 in, 1 out]
            }
          }
        }
        frame 9 {
          n537 = flat-sequence {
            tunnel: w1217 -> [w1222]
            tunnel: [w1219] -> w1216
            tunnel: w1216 -> [w1227]
            tunnel: [w1226] -> w1215
            tunnel: w1215 -> [w1235]
            tunnel: [w1234] -> w1214
            tunnel: w1214 -> [w1241]
            tunnel: [w1240] -> w1213
            tunnel: w1213 -> [w1247]
            frame #0 {
              # "-406"
              n538 = call "Auto Drive XY Left Automatic.vi"("RobotDriveDevRef In"=w1222, "Movement"=1.0, "Distance (in)"=-387.0, "Motor Output Range Y"=cluster{"output high":dbl, "output low":dbl} {"output high"=0.7, "output low"=-0.9}) -> ("RobotDriveDevRef Out"=w1219:T2)  [unwired: 11 in]
            }
            frame #1 {
              n539 = global write "Robot Global Data.vi" "Intake Speed Override"(-0.4 ("Arm Angle to Turn to")) -> ()
              n540 = call "Auto Drive XY Left Automatic.vi"("RobotDriveDevRef In"=w1227, "Angle Offset"=25.0, "Movement"=2.0, "Distance (in)"=80.0, "Motor Output Range Y"=cluster{"output high":dbl, "output low":dbl} {"output high"=0.5, "output low"=-0.7}) -> ("RobotDriveDevRef Out"=w1226:T2)  [unwired: 10 in]
            }
            frame #2 {
              n541 = global write "Robot Global Data.vi" "Intake Pistons"(WPI_SolenoidValue."Off" ("Intake Pistons")) -> ()
              n542 = global write "Robot Global Data.vi" "Auto Arm Fast"(FALSE ("Lift Down Fast")) -> ()
              n543 = call "Auto Drive XY Left Automatic.vi"("RobotDriveDevRef In"=w1235, "Angle Offset"=0.0, "Movement"=3.0, "Distance (in)"=-60.0, "Motor Output Range Y"=cluster{"output high":dbl, "output low":dbl} {"output high"=0.6, "output low"=-0.6}) -> ("RobotDriveDevRef Out"=w1234:T2)  [unwired: 10 in]
            }
            frame #3 {
              n544 = global write "Robot Global Data.vi" "Auto Arm Fast"(TRUE ("Lift Down Fast")) -> ()
              n545 = call <vilib>:"WPI_RobotDriveDelayAndUpdateSafety.vi"("Delay (s)"=0.5, "RobotDriveDevRef"=w1241) -> ("RobotDriveDevRef 2"=w1240:T2)  [unwired: 8 in, 1 out]
            }
            frame #4 {
              n546 = global write "Robot Global Data.vi" "Intake Speed Override"(1.0 ("Arm Angle to Turn to")) -> ()
              n547 = call "Auto Drive XY Left Automatic.vi"("RobotDriveDevRef In"=w1247, "Angle Offset"=30.0, "Distance (in)"=70.0) -> ()  [unwired: 12 in, 1 out]
              n548 = global write "Robot Global Data.vi" "Intake Pistons"(WPI_SolenoidValue."On" ("Intake Pistons")) -> ()
              n549 = global write "Robot Global Data.vi" "Arm Angle to Turn to"(0.0 ("Arm Angle to Turn to")) -> ()
              n550 = global write "Robot Global Data.vi" "Lift Height to rase to (in)"(0.0 ("Arm Angle to Turn to")) -> ()
            }
          }
        }
        frame 10 {
          n551 = flat-sequence {
            tunnel: w1250 -> [w1252]
            tunnel: [w1251] -> w1249
            tunnel: w1249 -> [w1256]
            frame #0 {
              n552 = call "Auto Drive XY Left Automatic.vi"("RobotDriveDevRef In"=w1252, "Movement"=1.0, "Distance (in)"=-416.0, "Motor Output Range Y"=cluster{"output high":dbl, "output low":dbl} {"output high"=0.7, "output low"=-0.9}) -> ("RobotDriveDevRef Out"=w1251:T2)  [unwired: 11 in]
            }
            frame #1 {
              n553 = global write "Robot Global Data.vi" "Arm Angle to Turn to"(0.0 ("Arm Angle to Turn to")) -> ()
              n554 = global write "Robot Global Data.vi" "Lift Height to rase to (in)"(0.0 ("Arm Angle to Turn to")) -> ()
              n555 = call "Auto Drive XY Left Automatic.vi"("RobotDriveDevRef In"=w1256, "Distance (in)"=30.0) -> ()  [unwired: 13 in, 1 out]
            }
          }
        }
        frame 11 {
          n556 = flat-sequence {
            tunnel: w1262 -> [w1267]
            tunnel: [w1264] -> w1261
            tunnel: w1261 -> [w1274]
            tunnel: [w1268] -> w1260
            tunnel: w1260 -> [w1276]
            frame #0 {
              n557 = call "Auto Drive XY Left Automatic.vi"("RobotDriveDevRef In"=w1267, "Movement"=1.0, "Distance (in)"=-600.0, "Motor Output Range Y"=cluster{"output high":dbl, "output low":dbl} {"output high"=0.85, "output low"=-0.95}) -> ("RobotDriveDevRef Out"=w1264:T2)  [unwired: 11 in]
            }
            frame #1 {
              n558 = global write "Robot Global Data.vi" "Intake Speed Override"(-0.5 ("Arm Angle to Turn to")) -> ()
              n559 = call "Auto Drive XY Left Automatic.vi"("RobotDriveDevRef In"=w1274, "Movement"=2.0, "Distance (in)"=150.0, "Time to Settle (ms)"=u32 150, "Motor Output Range Y"=cluster{"output high":dbl, "output low":dbl} {"output high"=0.75, "output low"=-0.7}) -> ("RobotDriveDevRef Out"=w1268:T2)  [unwired: 10 in]
            }
            frame #2 {
              n560 = global write "Robot Global Data.vi" "Arm Angle to Turn to"(0.0 ("Arm Angle to Turn to")) -> ()
              n561 = global write "Robot Global Data.vi" "Lift Height to rase to (in)"(0.0 ("Arm Angle to Turn to")) -> ()
              n562 = call "Auto Drive XY Left Automatic.vi"("RobotDriveDevRef In"=w1276, "Distance (in)"=-20.0) -> ()  [unwired: 13 in, 1 out]
              n563 = global write "Robot Global Data.vi" "Intake Pistons"(WPI_SolenoidValue."Off" ("Intake Pistons")) -> ()
            }
          }
        }
        frame 12 {
          n564 = flat-sequence {
            tunnel: w1282 -> [w1288]
            tunnel: [w1285] -> w1281
            tunnel: w1281 -> [w1294]
            tunnel: [w1290] -> w1280
            tunnel: w1280 -> [w1299]
            frame #0 {
              n565 = call "Auto Drive XY Left Automatic.vi"("RobotDriveDevRef In"=w1288, "Movement"=1.0, "Distance (in)"=-170.0, "Time to Settle (ms)"=u32 10, "Motor Output Range Y"=cluster{"output high":dbl, "output low":dbl} {"output high"=0.7, "output low"=-0.95}) -> ("RobotDriveDevRef Out"=w1285:T2)  [unwired: 10 in]
            }
            frame #1 {
              n566 = global write "Robot Global Data.vi" "Intake Speed Override"(-0.5 ("Intake Speed Override")) -> ()
              n567 = call "Auto Drive XY Left Automatic.vi"("RobotDriveDevRef In"=w1294, "Movement"=2.0, "Distance (in)"=300.0, "Time to Settle (ms)"=u32 100) -> ("RobotDriveDevRef Out"=w1290:T2)  [unwired: 11 in]
            }
            frame #2 {
              n568 = global write "Robot Global Data.vi" "Intake Pistons"(WPI_SolenoidValue."Off" ("Intake Pistons")) -> ()
              n569 = call "Auto Drive XY Left Automatic.vi"("RobotDriveDevRef In"=w1299, "Angle Offset"=90.0, "Movement"=3.0, "Motor Output Range X"=cluster{"output high":dbl, "output low":dbl} {"output high"=0.9, "output low"=-0.9}, "Distance (in)"=-160.0, "Motor Output Range Y"=cluster{"output high":dbl, "output low":dbl} {"output high"=0.7, "output low"=-0.9}) -> ()  [unwired: 9 in, 1 out]
            }
          }
        }
        frame 13 {
          n570 = flat-sequence {
            tunnel: w1306 -> [w1312]
            tunnel: [w1309] -> w1305
            tunnel: w1305 -> [w1318]
            tunnel: [w1315] -> w1304
            tunnel: w1304 -> [w1322]
            tunnel: [w1321] -> w1303
            tunnel: w1303 -> [w1330]
            tunnel: [w1324] -> w1302
            tunnel: w1302 -> [_]
            frame #0 {
              n571 = call "Auto Drive XY Left Automatic.vi"("RobotDriveDevRef In"=w1312, "Movement"=1.0, "Motor Output Range X"=cluster{"output high":dbl, "output low":dbl} {"output high"=0.8, "output low"=-0.8}, "Distance (in)"=-310.0, "Motor Output Range Y"=cluster{"output high":dbl, "output low":dbl} {"output high"=0.7, "output low"=-0.8}) -> ("RobotDriveDevRef Out"=w1309:T2)  [unwired: 10 in]
            }
            frame #1 {
              n572 = global write "Robot Global Data.vi" "Lift Height to rase to (in)"(60.0 ("Arm Angle to Turn to")) -> ()
              n573 = global write "Robot Global Data.vi" "Intake Speed Override"(0.0 ("Arm Angle to Turn to")) -> ()
              n574 = global write "Robot Global Data.vi" "Arm Angle to Turn to"(7000.0 ("Arm Angle to Turn to")) -> ()
              n575 = call "Auto Drive X.vi"("Angle to Turn (Deg)"=90.0 ("Distance (in)"), "RobotDriveDevRef In"=w1318) -> ("RobotDriveDevRef Out"=w1315:T2)  [unwired: 9 in]
            }
            frame #2 {
              n576 = global write "Robot Global Data.vi" "Intake Pistons"(WPI_SolenoidValue."Off" ("Intake Pistons")) -> ()
              n577 = call "Auto Drive XY Left Automatic.vi"("RobotDriveDevRef In"=w1322, "Distance (in)"=-20.0, "Motor Output Range Y"=cluster{"output high":dbl, "output low":dbl} {"output high"=0.6, "output low"=-0.6}) -> ("RobotDriveDevRef Out"=w1321:T2)  [unwired: 12 in]
            }
            frame #3 {
              n578 = global write "Robot Global Data.vi" "Intake Speed Override"(-0.6 ("Intake Speed Override")) -> ()
              n579 = global write "Robot Global Data.vi" "Intake Pistons"(WPI_SolenoidValue."Off" ("Intake Pistons")) -> ()
              n580 = call "Auto Drive XY Left Automatic.vi"("RobotDriveDevRef In"=w1330, "Movement"=3.0, "Distance (in)"=8.0, "Motor Output Range Y"=cluster{"output high":dbl, "output low":dbl} {"output high"=0.6, "output low"=-0.6}) -> ("RobotDriveDevRef Out"=w1324:T2)  [unwired: 11 in]
            }
            frame #4 {
              n581 = global write "Robot Global Data.vi" "Lift Height to rase to (in)"(0.0 ("Arm Angle to Turn to")) -> ()
              n582 = global write "Robot Global Data.vi" "Arm Angle to Turn to"(5000.0 ("Arm Angle to Turn to")) -> ()
            }
          }
        }
      }
    }
    frame "Right Automatic New" {
      # "RIGHT"
      # "-1 -  Drive Past Baseline, something went wrong\n1   - Close Switch, Close Scale\n2   - Close Switch, Close Switch\n3   - Far Switch,      Far Scale\n4   - Far Switch,      Far Switch\n5   - Drive Forward and turn\n6   - Close Scale,    Close Scale\n7   - Close Switch\n8   - Close Scale\n9   - Far Scale,         Far Scale\n10 - Far Scale\n11 - Far Switch\n12 - Close Switch, Far Scale"
      n583 = global read "Robot Global Data.vi" "Place From Null"() -> (w1338:bool)
      n584 = call <vilib>:"WPI_RobotDriveDelayAndUpdateSafety.vi"("Delay (s)"=0.125, "RobotDriveDevRef"=w1340) -> ("RobotDriveDevRef 2"=w1334:T2)  [unwired: 8 in, 1 out]
      n585 = case shown="True" w1338 {
        tunnel: [0 _] -> w1336
        tunnel: [w1667 w1799] -> w1335
        tunnel: w1334 -> [w1666 w1798]
        tunnel: [w1666 w1798] -> w1333
        frame False {
          # "Normal"
          # "1   - Close Switch, Close Scale\n2   - Close Switch, Close Switch\n3   - Far Switch,      Far Scale\n4   - Far Switch,      Far Switch\n5   - Drive Forward and turn\n6   - Close Scale,    Close Scale\n7   - Close Switch\n8   - Close Scale\n9   - Far Scale,         Far Scale\n10 - Far Scale\n11 - Far Switch\n12 - Close Switch, Far Scale"
          n586 = global read "Robot Global Data.vi" "Switch Position"() -> (w1672:string)
          n587 = global read "Robot Global Data.vi" "Scale Position"() -> (w1680:string)
          n588 = Equal?(x=w1672, y="R") -> (x = y?=w1671:bool)
          n589 = Select(t="L" ("y"), s=w1671, f="R" ("y")) -> (s? t:f=w1669:string)
          n590 = Equal?(x=w1680, y="R") -> (x = y?=w1678:bool)
          n591 = Select(t="L" ("y"), s=w1678, f="R" ("y")) -> (s? t:f=w1670:string)
          n592 = global read "Robot Global Data.vi" "Do Not Cross Field"() -> (w1681:bool)
          n593 = global read "Robot Global Data.vi" "Attempt 2 Cube"() -> (w1682:bool)
          n594 = global read "Robot Global Data.vi" "Focus Switch"() -> (w1683:bool)
          n595 = case shown="True" w1683 {
            tunnel: w1682 -> [w1688 w1745]
            tunnel: w1681 -> [w1687 w1744]
            tunnel: w1669 -> [w1686 w1743]
            tunnel: w1670 -> [w1685 w1742]
            tunnel: [w1684 w1741] -> w1667
            frame True {
              n596 = case shown="True" w1688 {
                tunnel: w1687 -> [w1692 w1718]
                tunnel: w1686 -> [w1691 w1717]
                tunnel: w1685 -> [w1690 w1716]
                tunnel: [w1689 w1715] -> w1684
                frame True {
                  n597 = case shown="False" w1692 {
                    tunnel: w1691 -> [w1695 w1706]
                    tunnel: w1690 -> [w1694 w1705]
                    tunnel: [w1693 w1704] -> w1689
                    frame True {
                      n598 = case shown="\"L\"" w1695 {
                        tunnel: w1694 -> [w1697 w1701]
                        tunnel: [w1696 w1700] -> w1693
                        frame "L" {
                          n599 = case shown="\"R\", Default" w1697 {
                            tunnel: [7 1] -> w1696
                            frame "R", Default {
                              # "2"
                            }
                            frame "L" {
                            }
                          }
                        }
                        frame "R", Default {
                          n600 = case shown="\"L\"" w1701 {
                            tunnel: [5 6] -> w1700
                            frame "R", Default {
                            }
                            frame "L" {
                            }
                          }
                        }
                      }
                    }
                    frame False {
                      n601 = case shown="\"L\"" w1706 {
                        tunnel: w1705 -> [w1708 w1712]
                        tunnel: [w1707 w1711] -> w1704
                        frame "L" {
                          n602 = case shown="\"L\"" w1708 {
                            tunnel: [12 1] -> w1707
                            frame "R", Default {
                            }
                            frame "L" {
                            }
                          }
                        }
                        frame "R", Default {
                          n603 = case shown="\"R\", Default" w1712 {
                            tunnel: [3 11] -> w1711
                            frame "R", Default {
                            }
                            frame "L" {
                              # "4"
                            }
                          }
                        }
                      }
                    }
                  }
                }
                frame False {
                  n604 = case shown="False" w1718 {
                    tunnel: w1717 -> [w1721 w1732]
                    tunnel: w1716 -> [w1720 w1731]
                    tunnel: [w1719 w1730] -> w1715
                    frame True {
                      n605 = case shown="\"L\"" w1721 {
                        tunnel: w1720 -> [w1723 w1727]
                        tunnel: [w1722 w1726] -> w1719
                        frame "L" {
                          n606 = case shown="\"R\", Default" w1723 {
                            tunnel: [7 7] -> w1722
                            frame "R", Default {
                            }
                            frame "L" {
                            }
                          }
                        }
                        frame "R", Default {
                          n607 = case shown="\"R\", Default" w1727 {
                            tunnel: [5 8] -> w1726
                            frame "R", Default {
                            }
                            frame "L" {
                            }
                          }
                        }
                      }
                    }
                    frame False {
                      n608 = case shown="\"R\", Default" w1732 {
                        tunnel: w1731 -> [w1734 w1738]
                        tunnel: [w1733 w1737] -> w1730
                        frame "L" {
                          n609 = case shown="\"L\"" w1734 {
                            tunnel: [7 7] -> w1733
                            frame "R", Default {
                            }
                            frame "L" {
                            }
                          }
                        }
                        frame "R", Default {
                          n610 = case shown="\"R\", Default" w1738 {
                            tunnel: [11 11] -> w1737
                            frame "R", Default {
                            }
                            frame "L" {
                            }
                          }
                        }
                      }
                    }
                  }
                }
              }
            }
            frame False {
              n611 = case shown="False" w1745 {
                tunnel: w1744 -> [w1749 w1775]
                tunnel: w1743 -> [w1748 w1774]
                tunnel: w1742 -> [w1747 w1773]
                tunnel: [w1746 w1772] -> w1741
                frame True {
                  n612 = case shown="False" w1749 {
                    tunnel: w1748 -> [w1752 w1763]
                    tunnel: w1747 -> [w1751 w1762]
                    tunnel: [w1750 w1761] -> w1746
                    frame True {
                      n613 = case shown="\"L\"" w1752 {
                        tunnel: w1751 -> [w1754 w1758]
                        tunnel: [w1753 w1757] -> w1750
                        frame "L" {
                          n614 = case shown="\"R\", Default" w1754 {
                            tunnel: [7 6] -> w1753
                            frame "R", Default {
                              # "2"
                            }
                            frame "L" {
                            }
                          }
                        }
                        frame "R", Default {
                          n615 = case shown="\"L\"" w1758 {
                            tunnel: [5 6] -> w1757
                            frame "R", Default {
                            }
                            frame "L" {
                            }
                          }
                        }
                      }
                    }
                    frame False {
                      n616 = case shown="\"R\", Default" w1763 {
                        tunnel: w1762 -> [w1765 w1769]
                        tunnel: [w1764 w1768] -> w1761
                        frame "L" {
                          n617 = case shown="\"R\", Default" w1765 {
                            tunnel: [9 6] -> w1764
                            frame "R", Default {
                            }
                            frame "L" {
                            }
                          }
                        }
                        frame "R", Default {
                          n618 = case shown="\"R\", Default" w1769 {
                            tunnel: [9 6] -> w1768
                            frame "R", Default {
                            }
                            frame "L" {
                            }
                          }
                        }
                      }
                    }
                  }
                }
                frame False {
                  n619 = case shown="False" w1775 {
                    tunnel: w1774 -> [w1778 w1789]
                    tunnel: w1773 -> [w1777 w1788]
                    tunnel: [w1776 w1787] -> w1772
                    frame True {
                      n620 = case shown="\"R\", Default" w1778 {
                        tunnel: w1777 -> [w1780 w1784]
                        tunnel: [w1779 w1783] -> w1776
                        frame "L" {
                          n621 = case shown="\"L\"" w1780 {
                            tunnel: [7 8] -> w1779
                            frame "R", Default {
                            }
                            frame "L" {
                            }
                          }
                        }
                        frame "R", Default {
                          n622 = case shown="\"L\"" w1784 {
                            tunnel: [5 8] -> w1783
                            frame "R", Default {
                            }
                            frame "L" {
                            }
                          }
                        }
                      }
                    }
                    frame False {
                      n623 = case shown="\"L\"" w1789 {
                        tunnel: w1788 -> [w1791 w1795]
                        tunnel: [w1790 w1794] -> w1787
                        frame "L" {
                          n624 = case shown="\"R\", Default" w1791 {
                            tunnel: [10 8] -> w1790
                            frame "R", Default {
                            }
                            frame "L" {
                            }
                          }
                        }
                        frame "R", Default {
                          n625 = case shown="\"R\", Default" w1795 {
                            tunnel: [10 8] -> w1794
                            frame "R", Default {
                            }
                            frame "L" {
                            }
                          }
                        }
                      }
                    }
                  }
                }
              }
            }
          }
          n626 = global write "Robot Global Data.vi" "Auto Running"(w1667) -> ()
        }
        frame True {
          # "PLACE FROM NULL"
          # "1   - Close Switch, Close Scale\n2   - Close Switch, Close Switch\n3   - Far Switch,      Far Scale\n4   - Far Switch,      Far Switch\n5   - Drive Forward and turn\n6   - Close Scale,    Close Scale\n7   - Close Switch\n8   - Close Scale\n9   - Far Scale,         Far Scale\n10 - Far Scale\n11 - Far Switch\n12 - Close Switch, Far Scale\n13 - Place from null"
          n627 = global read "Robot Global Data.vi" "Switch Position"() -> (w1803:string)
          n628 = global read "Robot Global Data.vi" "Scale Position"() -> (w1811:string)
          n629 = Equal?(x=w1803, y="L") -> (x = y?=w1802:bool)
          n630 = Select(t="R" ("y"), s=w1802, f="L" ("y")) -> (s? t:f=w1800:string)
          n631 = Equal?(x=w1811, y="R") -> (x = y?=w1809:bool)
          n632 = global read "Robot Global Data.vi" "Focus Switch"() -> (w1812:bool)
          n633 = Select(t="L" ("y"), s=w1809, f="R" ("y")) -> (s? t:f=w1801:string)
          n634 = case shown="True" w1812 {
            tunnel: w1800 -> [w1815 w1826]
            tunnel: w1801 -> [w1814 w1825]
            tunnel: [w1813 w1824] -> w1799
            frame False {
              n635 = case shown="\"L\"" w1815 {
                tunnel: w1814 -> [w1817 w1821]
                tunnel: [w1816 w1820] -> w1813
                frame "L" {
                  n636 = case shown="\"L\"" w1817 {
                    tunnel: [7 13] -> w1816
                    frame "R", Default {
                    }
                    frame "L" {
                    }
                  }
                }
                frame "R", Default {
                  n637 = case shown="\"L\"" w1821 {
                    tunnel: [5 13] -> w1820
                    frame "R", Default {
                    }
                    frame "L" {
                    }
                  }
                }
              }
            }
            frame True {
              n638 = case shown="\"R\", Default" w1826 {
                tunnel: w1825 -> [w1828 w1832]
                tunnel: [w1827 w1831] -> w1824
                frame "L" {
                  n639 = case shown="\"L\"" w1828 {
                    tunnel: [7 7] -> w1827
                    frame "R", Default {
                    }
                    frame "L" {
                    }
                  }
                }
                frame "R", Default {
                  n640 = case shown="\"R\", Default" w1832 {
                    tunnel: [5 13] -> w1831
                    frame "R", Default {
                    }
                    frame "L" {
                    }
                  }
                }
              }
            }
          }
          n641 = global write "Robot Global Data.vi" "Auto Running"(w1799) -> ()
        }
      }
      n642 = global read "Robot Global Data.vi" "Continuos Yaw"() -> (w1337:dbl)
      n643 = global write "Robot Global Data.vi" "Angle at Start of Auto"(w1337) -> ()
      n644 = case shown="1" w1335 {
        tunnel: w1333 -> [w1342 w1346 w1378 w1417 w1444 w1471 w1480 w1513 w1535 w1550 w1583 w1595 w1615 w1639]
        tunnel: w1336 -> [_ _ _ _ _ _ _ _ _ _ _ _ _ _]
        frame -1, Default {
          n645 = call "Auto Drive XY Left Automatic.vi"("RobotDriveDevRef In"=w1342, "Distance (in)"=-150.0) -> ()  [unwired: 13 in, 1 out]
        }
        frame 1 {
          n646 = flat-sequence {
            tunnel: w1346 -> [w1352]
            tunnel: [w1349] -> w1345
            tunnel: w1345 -> [w1358]
            tunnel: [w1354] -> w1344
            tunnel: w1344 -> [w1363]
            tunnel: [w1362] -> w1343
            tunnel: w1343 -> [w1371]
            frame #0 {
              n647 = call "Auto Drive XY Left Automatic.vi"("RobotDriveDevRef In"=w1352, "Movement"=1.0, "Distance (in)"=-180.0, "Time to Settle (ms)"=u32 10, "Motor Output Range Y"=cluster{"output high":dbl, "output low":dbl} {"output high"=0.7, "output low"=-0.75}) -> ("RobotDriveDevRef Out"=w1349:T2)  [unwired: 10 in]
            }
            frame #1 {
              n648 = global write "Robot Global Data.vi" "Intake Speed Override"(-0.5 ("Intake Speed Override")) -> ()
              n649 = call "Auto Drive XY Left Automatic.vi"("RobotDriveDevRef In"=w1358, "Movement"=2.0, "Distance (in)"=300.0, "Time to Settle (ms)"=u32 100) -> ("RobotDriveDevRef Out"=w1354:T2)  [unwired: 11 in]
            }
            frame #2 {
              n650 = global write "Robot Global Data.vi" "Intake Pistons"(WPI_SolenoidValue."Off" ("Intake Pistons")) -> ()
              n651 = call "Auto Drive XY Left Automatic.vi"("RobotDriveDevRef In"=w1363, "Movement"=3.0, "Distance (in)"=-55.0, "Time to Settle (ms)"=u32 500, "Motor Output Range Y"=cluster{"output high":dbl, "output low":dbl} {"output high"=0.7, "output low"=-0.8}) -> ("RobotDriveDevRef Out"=w1362:T2)  [unwired: 10 in]
            }
            frame #3 {
              n652 = global write "Robot Global Data.vi" "Intake Speed Override"(-0.3 ("Arm Angle to Turn to")) -> ()
              n653 = call "Auto Drive XY Left Automatic.vi"("RobotDriveDevRef In"=w1371, "Distance (in)"=20.0, "Motor Output Range Y"=cluster{"output high":dbl, "output low":dbl} {"output high"=0.6, "output low"=-0.7}) -> ()  [unwired: 12 in, 1 out]
              n654 = global write "Robot Global Data.vi" "Lift Height to rase to (in)"(0.0 ("Arm Angle to Turn to")) -> ()
              n655 = global write "Robot Global Data.vi" "Arm Angle to Turn to"(0.0 ("Arm Angle to Turn to")) -> ()
            }
          }
        }
        frame 2 {
          n656 = flat-sequence {
            tunnel: w1378 -> [w1384]
            tunnel: [w1381] -> w1377
            tunnel: w1377 -> [w1390]
            tunnel: [w1386] -> w1376
            tunnel: w1376 -> [w1396]
            tunnel: [w1395] -> w1374
            tunnel: w1374 -> [w1400]
            tunnel: [w1399] -> w1373
            tunnel: w1373 -> [w1402]
            tunnel: [w1401] -> w1372
            tunnel: w1372 -> [w1405]
            tunnel: [w1406] -> w1375
            tunnel: w1375 -> [w1411]
            frame #0 {
              n657 = call "Auto Drive XY Left Automatic.vi"("RobotDriveDevRef In"=w1384, "Movement"=1.0, "Distance (in)"=-170.0, "Time to Settle (ms)"=u32 10, "Motor Output Range Y"=cluster{"output high":dbl, "output low":dbl} {"output high"=0.7, "output low"=-0.75}) -> ("RobotDriveDevRef Out"=w1381:T2)  [unwired: 10 in]
            }
            frame #1 {
              n658 = global write "Robot Global Data.vi" "Intake Speed Override"(-0.5 ("Intake Speed Override")) -> ()
              n659 = call "Auto Drive XY Left Automatic.vi"("RobotDriveDevRef In"=w1390, "Movement"=2.0, "Distance (in)"=300.0, "Time to Settle (ms)"=u32 100) -> ("RobotDriveDevRef Out"=w1386:T2)  [unwired: 11 in]
            }
            frame #2 {
              n660 = call <vilib>:"WPI_RobotDriveDelayAndUpdateSafety.vi"("Delay (s)"=1.0, "RobotDriveDevRef"=w1396) -> ("RobotDriveDevRef 2"=w1395:T2)  [unwired: 8 in, 1 out]
              n661 = global write "Robot Global Data.vi" "Lift Height to rase to (in)"(40.0 ("Arm Angle to Turn to")) -> ()
              n662 = global write "Robot Global Data.vi" "Arm Angle to Turn to"(500.0 ("Arm Angle to Turn to")) -> ()
              n663 = global write "Robot Global Data.vi" "Intake Pistons"(WPI_SolenoidValue."Off" ("Intake Pistons")) -> ()
            }
            frame #3 {
              n664 = call-poly <vilib>:"WPI_RobotDriveArcadeDrive.vi"("Y axis value"=0.6, "X axis value"=0.0, "RobotDriveDevRef"=w1400) -> ("RobotDriveDevRef"=w1399:T2)  [unwired: 6 in, 2 out]
            }
            frame #4 {
              n665 = call <vilib>:"WPI_RobotDriveDelayAndUpdateSafety.vi"("Delay (s)"=0.25, "RobotDriveDevRef"=w1402) -> ("RobotDriveDevRef 2"=w1401:T2)  [unwired: 8 in, 1 out]
            }
            frame #5 {
              n666 = call <vilib>:"WPI_RobotDriveDelayAndUpdateSafety.vi"("Delay (s)"=1.0, "RobotDriveDevRef"=w1405) -> ("RobotDriveDevRef 2"=w1406:T2)  [unwired: 8 in, 1 out]
              n667 = global write "Robot Global Data.vi" "Intake Speed Override"(-0.8 ("Arm Angle to Turn to")) -> ()
            }
            frame #6 {
              n668 = global write "Robot Global Data.vi" "Intake Speed Override"(0.0 ("Intake Speed Override")) -> ()
              n669 = global write "Robot Global Data.vi" "Lift Height to rase to (in)"(0.0 ("Arm Angle to Turn to")) -> ()
              n670 = global write "Robot Global Data.vi" "Arm Angle to Turn to"(0.0 ("Arm Angle to Turn to")) -> ()
              n671 = call "Auto Drive XY Left Automatic.vi"("RobotDriveDevRef In"=w1411, "Movement"=3.0, "Distance (in)"=-30.0) -> ()  [unwired: 12 in, 1 out]
            }
          }
        }
        frame 3 {
          n672 = flat-sequence {
            tunnel: w1417 -> [w1422]
            tunnel: [w1419] -> w1416
            tunnel: w1416 -> [w1429]
            tunnel: [w1426] -> w1415
            tunnel: w1415 -> [w1432]
            tunnel: [w1431] -> w1414
            tunnel: w1414 -> [w1438]
            frame #0 {
              n673 = call "Auto Drive XY Left Automatic.vi"("RobotDriveDevRef In"=w1422, "Movement"=1.0, "Distance (in)"=-600.0, "Motor Output Range Y"=cluster{"output high":dbl, "output low":dbl} {"output high"=0.85, "output low"=-0.95}) -> ("RobotDriveDevRef Out"=w1419:T2)  [unwired: 11 in]
            }
            frame #1 {
              n674 = global write "Robot Global Data.vi" "Intake Speed Override"(-0.5 ("Arm Angle to Turn to")) -> ()
              n675 = call "Auto Drive XY Left Automatic.vi"("RobotDriveDevRef In"=w1429, "Movement"=2.0, "Distance (in)"=150.0, "Time to Settle (ms)"=u32 150, "Motor Output Range Y"=cluster{"output high":dbl, "output low":dbl} {"output high"=0.75, "output low"=-0.7}) -> ("RobotDriveDevRef Out"=w1426:T2)  [unwired: 10 in]
            }
            frame #2 {
              n676 = call "Auto Drive XY Left Automatic.vi"("RobotDriveDevRef In"=w1432, "Movement"=3.0, "Distance (in)"=-60.0) -> ("RobotDriveDevRef Out"=w1431:T2)  [unwired: 12 in]
              n677 = global write "Robot Global Data.vi" "Intake Pistons"(WPI_SolenoidValue."Off" ("Intake Pistons")) -> ()
            }
            frame #3 {
              n678 = call "Auto Drive XY Left Automatic.vi"("RobotDriveDevRef In"=w1438, "Distance (in)"=25.0) -> ()  [unwired: 13 in, 1 out]
              n679 = global write "Robot Global Data.vi" "Intake Speed Override"(0.0 ("Arm Angle to Turn to")) -> ()
              n680 = global write "Robot Global Data.vi" "Lift Height to rase to (in)"(0.0 ("Arm Angle to Turn to")) -> ()
              n681 = global write "Robot Global Data.vi" "Arm Angle to Turn to"(0.0 ("Arm Angle to Turn to")) -> ()
            }
          }
        }
        frame 4 {
          n682 = flat-sequence {
            tunnel: w1444 -> [w1449]
            tunnel: [w1446] -> w1443
            tunnel: w1443 -> [w1456]
            tunnel: [w1453] -> w1442
            tunnel: w1442 -> [w1462]
            tunnel: [w1461] -> w1441
            tunnel: w1441 -> [w1466]
            tunnel: [w1465] -> w1440
            tunnel: w1440 -> [w1469]
            frame #0 {
              n683 = call "Auto Drive XY Left Automatic.vi"("RobotDriveDevRef In"=w1449, "Movement"=1.0, "Distance (in)"=-600.0, "Motor Output Range Y"=cluster{"output high":dbl, "output low":dbl} {"output high"=0.85, "output low"=-0.95}) -> ("RobotDriveDevRef Out"=w1446:T2)  [unwired: 11 in]
            }
            frame #1 {
              n684 = global write "Robot Global Data.vi" "Intake Speed Override"(-0.5 ("Arm Angle to Turn to")) -> ()
              n685 = call "Auto Drive XY Left Automatic.vi"("RobotDriveDevRef In"=w1456, "Movement"=2.0, "Distance (in)"=150.0, "Time to Settle (ms)"=u32 150, "Motor Output Range Y"=cluster{"output high":dbl, "output low":dbl} {"output high"=0.75, "output low"=-0.7}) -> ("RobotDriveDevRef Out"=w1453:T2)  [unwired: 10 in]
            }
            frame #2 {
              n686 = call <vilib>:"WPI_RobotDriveDelayAndUpdateSafety.vi"("Delay (s)"=0.5, "RobotDriveDevRef"=w1462) -> ("RobotDriveDevRef 2"=w1461:T2)  [unwired: 8 in, 1 out]
              n687 = global write "Robot Global Data.vi" "Lift Height to rase to (in)"(30.0 ("Arm Angle to Turn to")) -> ()
              n688 = global write "Robot Global Data.vi" "Arm Angle to Turn to"(500.0 ("Arm Angle to Turn to")) -> ()
              n689 = global write "Robot Global Data.vi" "Intake Pistons"(WPI_SolenoidValue."Off" ("Intake Pistons")) -> ()
            }
            frame #3 {
              n690 = call <vilib>:"WPI_RobotDriveDelayAndUpdateSafety.vi"("Delay (s)"=1.0, "RobotDriveDevRef"=w1466) -> ("RobotDriveDevRef 2"=w1465:T2)  [unwired: 8 in, 1 out]
              n691 = global write "Robot Global Data.vi" "Intake Speed Override"(1.0 ("Arm Angle to Turn to")) -> ()
            }
            frame #4 {
              n692 = global write "Robot Global Data.vi" "Arm Angle to Turn to"(0.0 ("Arm Angle to Turn to")) -> ()
              n693 = global write "Robot Global Data.vi" "Lift Height to rase to (in)"(0.0 ("Arm Angle to Turn to")) -> ()
              n694 = call "Auto Drive XY Left Automatic.vi"("RobotDriveDevRef In"=w1469, "Distance (in)"=30.0) -> ()  [unwired: 13 in, 1 out]
            }
          }
        }
        frame 5 {
          n695 = flat-sequence {
            tunnel: w1471 -> [w1474]
            frame #0 {
              n696 = call "Auto Drive XY Left Automatic.vi"("RobotDriveDevRef In"=w1474, "Movement"=1.0, "Distance (in)"=-250.0) -> ()  [unwired: 12 in, 1 out]
            }
            frame #1 {
              n697 = global write "Robot Global Data.vi" "Lift Height to rase to (in)"(0.0 ("Arm Angle to Turn to")) -> ()
              n698 = global write "Robot Global Data.vi" "Arm Angle to Turn to"(0.0 ("Arm Angle to Turn to")) -> ()
            }
          }
        }
        frame 6 {
          n699 = flat-sequence {
            tunnel: w1480 -> [w1486]
            tunnel: [w1483] -> w1479
            tunnel: w1479 -> [w1497]
            tunnel: [w1492] -> w1478
            tunnel: w1478 -> [w1503]
            tunnel: [w1498] -> w1477
            tunnel: w1477 -> [w1510]
            frame #0 {
              n700 = call "Auto Drive XY Left Automatic.vi"("RobotDriveDevRef In"=w1486, "Movement"=1.0, "Motor Output Range X"=cluster{"output high":dbl, "output low":dbl} {"output high"=0.8, "output low"=-0.8}, "Distance (in)"=-282.0, "Motor Output Range Y"=cluster{"output high":dbl, "output low":dbl} {"output high"=0.7, "output low"=-0.8}) -> ("RobotDriveDevRef Out"=w1483:T2)  [unwired: 10 in]
            }
            frame #1 {
              n701 = global write "Robot Global Data.vi" "Lift Height to rase to (in)"(0.0 ("Arm Angle to Turn to")) -> ()
              n702 = global write "Robot Global Data.vi" "Intake Speed Override"(-0.5 ("Arm Angle to Turn to")) -> ()
              n703 = global write "Robot Global Data.vi" "Arm Angle to Turn to"(0.0 ("Arm Angle to Turn to")) -> ()
              n704 = global write "Robot Global Data.vi" "Auto Arm Fast"(TRUE ("Lift Down Fast")) -> ()
              n705 = global write "Robot Global Data.vi" "Lift Down Fast"(TRUE ("Lift Down Fast")) -> ()
              n706 = call "Auto Drive XY Left Automatic.vi"("RobotDriveDevRef In"=w1497, "Angle Offset"=-10.0, "Movement"=2.0, "Distance (in)"=77.0, "Motor Output Range Y"=cluster{"output high":dbl, "output low":dbl} {"output high"=0.6, "output low"=-0.7}) -> ("RobotDriveDevRef Out"=w1492:T2)  [unwired: 10 in]
            }
            frame #2 {
              n707 = global write "Robot Global Data.vi" "Auto Arm Fast"(FALSE ("Lift Down Fast")) -> ()
              n708 = global write "Robot Global Data.vi" "Lift Down Fast"(FALSE ("Lift Down Fast")) -> ()
              n709 = global write "Robot Global Data.vi" "Intake Pistons"(WPI_SolenoidValue."Off" ("Intake Pistons")) -> ()
              n710 = call "Auto Drive XY Left Automatic.vi"("RobotDriveDevRef In"=w1503, "Movement"=3.0, "Distance (in)"=-57.0) -> ("RobotDriveDevRef Out"=w1498:T2)  [unwired: 12 in]
            }
            frame #3 {
              n711 = global write "Robot Global Data.vi" "Intake Speed Override"(0.0 ("Intake Speed Override")) -> ()
              n712 = global write "Robot Global Data.vi" "Intake Pistons"(WPI_SolenoidValue."On" ("Intake Pistons")) -> ()
              n713 = call "Auto Drive XY Left Automatic.vi"("RobotDriveDevRef In"=w1510, "Movement"=4.0, "Distance (in)"=30.0, "Motor Output Range Y"=cluster{"output high":dbl, "output low":dbl} {"output high"=0.6, "output low"=-0.6}) -> ()  [unwired: 11 in, 1 out]
            }
          }
        }
        frame 7 {
          n714 = flat-sequence {
            tunnel: [w1516] -> w1514
            tunnel: w1513 -> [w1515]
            tunnel: w1514 -> [w1522]
            tunnel: [w1521] -> w1512
            tunnel: w1512 -> [w1531]
            tunnel: [w1530] -> w1511
            tunnel: [w1533] -> _
            tunnel: w1511 -> [w1533]
            frame #0 {
              n715 = call "Auto Drive XY Left Automatic.vi"("RobotDriveDevRef In"=w1515, "Movement"=1.0, "Distance (in)"=-170.0, "Time to Settle (ms)"=u32 10, "Motor Output Range Y"=cluster{"output high":dbl, "output low":dbl} {"output high"=0.7, "output low"=-0.75}) -> ("RobotDriveDevRef Out"=w1516:T2)  [unwired: 10 in]
            }
            frame #1 {
              n716 = global write "Robot Global Data.vi" "Intake Speed Override"(-0.5 ("Intake Speed Override")) -> ()
              n717 = call "Auto Drive XY Left Automatic.vi"("RobotDriveDevRef In"=w1522, "Movement"=2.0, "Distance (in)"=300.0, "Time to Settle (ms)"=u32 100) -> ("RobotDriveDevRef Out"=w1521:T2)  [unwired: 11 in]
            }
            frame #2 {
              n718 = call "Auto Drive XY Left Automatic.vi"("RobotDriveDevRef In"=w1531, "Angle Offset"=-90.0, "Distance (in)"=-70.0) -> ("RobotDriveDevRef Out"=w1530:T2)  [unwired: 12 in]
              n719 = global write "Robot Global Data.vi" "Intake Pistons"(WPI_SolenoidValue."Off" ("Intake Pistons")) -> ()
            }
            frame #3 {
              n720 = global write "Robot Global Data.vi" "Intake Speed Override"(0.0 ("Intake Speed Override")) -> ()
            }
          }
        }
        frame 8 {
          n721 = flat-sequence {
            tunnel: w1535 -> [w1536]
            tunnel: [w1537] -> w1534
            tunnel: w1534 -> [w1542]
            frame #0 {
              n722 = call "Auto Drive XY Left Automatic.vi"("RobotDriveDevRef In"=w1536, "Movement"=1.0, "Motor Output Range X"=cluster{"output high":dbl, "output low":dbl} {"output high"=0.8, "output low"=-0.8}, "Distance (in)"=-273.0, "Motor Output Range Y"=cluster{"output high":dbl, "output low":dbl} {"output high"=0.7, "output low"=-0.8}) -> ("RobotDriveDevRef Out"=w1537:T2)  [unwired: 10 in]
            }
            frame #1 {
              n723 = global write "Robot Global Data.vi" "Arm Angle to Turn to"(0.0 ("Arm Angle to Turn to")) -> ()
              n724 = global write "Robot Global Data.vi" "Lift Height to rase to (in)"(0.0 ("Arm Angle to Turn to")) -> ()
              n725 = call "Auto Drive XY Left Automatic.vi"("RobotDriveDevRef In"=w1542, "Distance (in)"=30.0) -> ()  [unwired: 13 in, 1 out]
            }
          }
        }
        frame 9 {
          n726 = flat-sequence {
            tunnel: w1550 -> [w1555]
            tunnel: [w1552] -> w1549
            tunnel: w1549 -> [w1560]
            tunnel: [w1559] -> w1548
            tunnel: w1548 -> [w1568]
            tunnel: [w1567] -> w1547
            tunnel: w1547 -> [w1574]
            tunnel: [w1573] -> w1546
            tunnel: w1546 -> [w1580]
            frame #0 {
              # "-406"
              n727 = call "Auto Drive XY Left Automatic.vi"("RobotDriveDevRef In"=w1555, "Movement"=1.0, "Distance (in)"=-387.0, "Motor Output Range Y"=cluster{"output high":dbl, "output low":dbl} {"output high"=0.7, "output low"=-0.9}) -> ("RobotDriveDevRef Out"=w1552:T2)  [unwired: 11 in]
            }
            frame #1 {
              n728 = global write "Robot Global Data.vi" "Intake Speed Override"(-0.4 ("Arm Angle to Turn to")) -> ()
              n729 = call "Auto Drive XY Left Automatic.vi"("RobotDriveDevRef In"=w1560, "Angle Offset"=25.0, "Movement"=2.0, "Distance (in)"=80.0, "Motor Output Range Y"=cluster{"output high":dbl, "output low":dbl} {"output high"=0.5, "output low"=-0.7}) -> ("RobotDriveDevRef Out"=w1559:T2)  [unwired: 10 in]
            }
            frame #2 {
              n730 = global write "Robot Global Data.vi" "Intake Pistons"(WPI_SolenoidValue."Off" ("Intake Pistons")) -> ()
              n731 = global write "Robot Global Data.vi" "Auto Arm Fast"(FALSE ("Lift Down Fast")) -> ()
              n732 = call "Auto Drive XY Left Automatic.vi"("RobotDriveDevRef In"=w1568, "Angle Offset"=0.0, "Movement"=3.0, "Distance (in)"=-60.0, "Motor Output Range Y"=cluster{"output high":dbl, "output low":dbl} {"output high"=0.6, "output low"=-0.6}) -> ("RobotDriveDevRef Out"=w1567:T2)  [unwired: 10 in]
            }
            frame #3 {
              n733 = global write "Robot Global Data.vi" "Auto Arm Fast"(TRUE ("Lift Down Fast")) -> ()
              n734 = call <vilib>:"WPI_RobotDriveDelayAndUpdateSafety.vi"("Delay (s)"=0.5, "RobotDriveDevRef"=w1574) -> ("RobotDriveDevRef 2"=w1573:T2)  [unwired: 8 in, 1 out]
            }
            frame #4 {
              n735 = global write "Robot Global Data.vi" "Intake Speed Override"(1.0 ("Arm Angle to Turn to")) -> ()
              n736 = call "Auto Drive XY Left Automatic.vi"("RobotDriveDevRef In"=w1580, "Angle Offset"=30.0, "Distance (in)"=70.0) -> ()  [unwired: 12 in, 1 out]
              n737 = global write "Robot Global Data.vi" "Intake Pistons"(WPI_SolenoidValue."On" ("Intake Pistons")) -> ()
              n738 = global write "Robot Global Data.vi" "Arm Angle to Turn to"(0.0 ("Arm Angle to Turn to")) -> ()
              n739 = global write "Robot Global Data.vi" "Lift Height to rase to (in)"(0.0 ("Arm Angle to Turn to")) -> ()
            }
          }
        }
        frame 10 {
          n740 = flat-sequence {
            tunnel: w1583 -> [w1585]
            tunnel: [w1584] -> w1582
            tunnel: w1582 -> [w1589]
            frame #0 {
              n741 = call "Auto Drive XY Left Automatic.vi"("RobotDriveDevRef In"=w1585, "Movement"=1.0, "Distance (in)"=-416.0, "Motor Output Range Y"=cluster{"output high":dbl, "output low":dbl} {"output high"=0.7, "output low"=-0.9}) -> ("RobotDriveDevRef Out"=w1584:T2)  [unwired: 11 in]
            }
            frame #1 {
              n742 = global write "Robot Global Data.vi" "Arm Angle to Turn to"(0.0 ("Arm Angle to Turn to")) -> ()
              n743 = global write "Robot Global Data.vi" "Lift Height to rase to (in)"(0.0 ("Arm Angle to Turn to")) -> ()
              n744 = call "Auto Drive XY Left Automatic.vi"("RobotDriveDevRef In"=w1589, "Distance (in)"=30.0) -> ()  [unwired: 13 in, 1 out]
            }
          }
        }
        frame 11 {
          n745 = flat-sequence {
            tunnel: w1595 -> [w1600]
            tunnel: [w1597] -> w1594
            tunnel: w1594 -> [w1607]
            tunnel: [w1601] -> w1593
            tunnel: w1593 -> [w1609]
            frame #0 {
              n746 = call "Auto Drive XY Left Automatic.vi"("RobotDriveDevRef In"=w1600, "Movement"=1.0, "Distance (in)"=-600.0, "Motor Output Range Y"=cluster{"output high":dbl, "output low":dbl} {"output high"=0.85, "output low"=-0.95}) -> ("RobotDriveDevRef Out"=w1597:T2)  [unwired: 11 in]
            }
            frame #1 {
              n747 = global write "Robot Global Data.vi" "Intake Speed Override"(-0.5 ("Arm Angle to Turn to")) -> ()
              n748 = call "Auto Drive XY Left Automatic.vi"("RobotDriveDevRef In"=w1607, "Movement"=2.0, "Distance (in)"=150.0, "Time to Settle (ms)"=u32 150, "Motor Output Range Y"=cluster{"output high":dbl, "output low":dbl} {"output high"=0.75, "output low"=-0.7}) -> ("RobotDriveDevRef Out"=w1601:T2)  [unwired: 10 in]
            }
            frame #2 {
              n749 = global write "Robot Global Data.vi" "Arm Angle to Turn to"(0.0 ("Arm Angle to Turn to")) -> ()
              n750 = global write "Robot Global Data.vi" "Lift Height to rase to (in)"(0.0 ("Arm Angle to Turn to")) -> ()
              n751 = call "Auto Drive XY Left Automatic.vi"("RobotDriveDevRef In"=w1609, "Distance (in)"=-20.0) -> ()  [unwired: 13 in, 1 out]
              n752 = global write "Robot Global Data.vi" "Intake Pistons"(WPI_SolenoidValue."Off" ("Intake Pistons")) -> ()
            }
          }
        }
        frame 12 {
          n753 = flat-sequence {
            tunnel: w1615 -> [w1621]
            tunnel: [w1618] -> w1614
            tunnel: w1614 -> [w1627]
            tunnel: [w1623] -> w1613
            tunnel: w1613 -> [w1632]
            frame #0 {
              n754 = call "Auto Drive XY Left Automatic.vi"("RobotDriveDevRef In"=w1621, "Movement"=1.0, "Distance (in)"=-170.0, "Time to Settle (ms)"=u32 10, "Motor Output Range Y"=cluster{"output high":dbl, "output low":dbl} {"output high"=0.7, "output low"=-0.95}) -> ("RobotDriveDevRef Out"=w1618:T2)  [unwired: 10 in]
            }
            frame #1 {
              n755 = global write "Robot Global Data.vi" "Intake Speed Override"(-0.5 ("Intake Speed Override")) -> ()
              n756 = call "Auto Drive XY Left Automatic.vi"("RobotDriveDevRef In"=w1627, "Movement"=2.0, "Distance (in)"=300.0, "Time to Settle (ms)"=u32 100) -> ("RobotDriveDevRef Out"=w1623:T2)  [unwired: 11 in]
            }
            frame #2 {
              n757 = global write "Robot Global Data.vi" "Intake Pistons"(WPI_SolenoidValue."Off" ("Intake Pistons")) -> ()
              n758 = call "Auto Drive XY Left Automatic.vi"("RobotDriveDevRef In"=w1632, "Angle Offset"=90.0, "Movement"=3.0, "Motor Output Range X"=cluster{"output high":dbl, "output low":dbl} {"output high"=0.9, "output low"=-0.9}, "Distance (in)"=-160.0, "Motor Output Range Y"=cluster{"output high":dbl, "output low":dbl} {"output high"=0.7, "output low"=-0.9}) -> ()  [unwired: 9 in, 1 out]
            }
          }
        }
        frame 13 {
          n759 = flat-sequence {
            tunnel: w1639 -> [w1645]
            tunnel: [w1642] -> w1638
            tunnel: w1638 -> [w1651]
            tunnel: [w1648] -> w1637
            tunnel: w1637 -> [w1655]
            tunnel: [w1654] -> w1636
            tunnel: w1636 -> [w1663]
            tunnel: [w1657] -> w1635
            tunnel: w1635 -> [_]
            frame #0 {
              n760 = call "Auto Drive XY Left Automatic.vi"("RobotDriveDevRef In"=w1645, "Movement"=1.0, "Motor Output Range X"=cluster{"output high":dbl, "output low":dbl} {"output high"=0.8, "output low"=-0.8}, "Distance (in)"=-310.0, "Motor Output Range Y"=cluster{"output high":dbl, "output low":dbl} {"output high"=0.7, "output low"=-0.8}) -> ("RobotDriveDevRef Out"=w1642:T2)  [unwired: 10 in]
            }
            frame #1 {
              n761 = global write "Robot Global Data.vi" "Lift Height to rase to (in)"(60.0 ("Arm Angle to Turn to")) -> ()
              n762 = global write "Robot Global Data.vi" "Intake Speed Override"(0.0 ("Arm Angle to Turn to")) -> ()
              n763 = global write "Robot Global Data.vi" "Arm Angle to Turn to"(7000.0 ("Arm Angle to Turn to")) -> ()
              n764 = call "Auto Drive X.vi"("Angle to Turn (Deg)"=90.0 ("Distance (in)"), "RobotDriveDevRef In"=w1651) -> ("RobotDriveDevRef Out"=w1648:T2)  [unwired: 9 in]
            }
            frame #2 {
              n765 = global write "Robot Global Data.vi" "Intake Pistons"(WPI_SolenoidValue."Off" ("Intake Pistons")) -> ()
              n766 = call "Auto Drive XY Left Automatic.vi"("RobotDriveDevRef In"=w1655, "Distance (in)"=-20.0, "Motor Output Range Y"=cluster{"output high":dbl, "output low":dbl} {"output high"=0.6, "output low"=-0.6}) -> ("RobotDriveDevRef Out"=w1654:T2)  [unwired: 12 in]
            }
            frame #3 {
              n767 = global write "Robot Global Data.vi" "Intake Speed Override"(-0.6 ("Intake Speed Override")) -> ()
              n768 = global write "Robot Global Data.vi" "Intake Pistons"(WPI_SolenoidValue."Off" ("Intake Pistons")) -> ()
              n769 = call "Auto Drive XY Left Automatic.vi"("RobotDriveDevRef In"=w1663, "Movement"=3.0, "Distance (in)"=8.0, "Motor Output Range Y"=cluster{"output high":dbl, "output low":dbl} {"output high"=0.6, "output low"=-0.6}) -> ("RobotDriveDevRef Out"=w1657:T2)  [unwired: 11 in]
            }
            frame #4 {
              n770 = global write "Robot Global Data.vi" "Lift Height to rase to (in)"(0.0 ("Arm Angle to Turn to")) -> ()
              n771 = global write "Robot Global Data.vi" "Arm Angle to Turn to"(5000.0 ("Arm Angle to Turn to")) -> ()
            }
          }
        }
      }
    }
    frame "Right Automatic New Old" {
      # "-1 -  Drive Past Baseline, something went wrong\n1   - Close Switch, Close Scale\n2   - Close Switch, Close Switch\n3   - Far Switch,      Far Scale\n4   - Far Switch,      Far Switch\n5   - Drive Forward and turn\n6   - Close Scale,    Close Scale\n7   - Close Switch\n8   - Close Scale\n9   - Far Scale,         Far Scale\n10 - Far Scale\n11 - Far Switch\n12 - Close Switch, Far Scale"
      # "1   - Close Switch, Close Scale\n2   - Close Switch, Close Switch\n3   - Far Switch,      Far Scale\n4   - Far Switch,      Far Switch\n5   - Drive Forward and turn\n6   - Close Scale,    Close Scale\n7   - Close Switch\n8   - Close Scale\n9   - Far Scale,         Far Scale\n10 - Far Scale\n11 - Far Switch\n12 - Close Switch, Far Scale"
      n772 = global read "Robot Global Data.vi" "Switch Position"() -> (w1837:string)
      n773 = global read "Robot Global Data.vi" "Scale Position"() -> (w1846:string)
      n774 = global read "Robot Global Data.vi" "Do Not Cross Field"() -> (w1850:bool)
      n775 = global read "Robot Global Data.vi" "Attempt 2 Cube"() -> (w1851:bool)
      n776 = call <vilib>:"WPI_RobotDriveDelayAndUpdateSafety.vi"("Delay (s)"=0.125, "RobotDriveDevRef"=w1854) -> ("RobotDriveDevRef 2"=w1848:T2)  [unwired: 8 in, 1 out]
      n777 = global read "Robot Global Data.vi" "Focus Switch"() -> (w1852:bool)
      n778 = Equal?(x=w1837, y="L") -> (x = y?=w1836:bool)
      n779 = Select(t="R" ("y"), s=w1836, f="L" ("y")) -> (s? t:f=w1835:string)
      n780 = Equal?(x=w1846, y="R") -> (x = y?=w1844:bool)
      n781 = Select(t="L" ("y"), s=w1844, f="R" ("y")) -> (s? t:f=w1841:string)
      n782 = case shown="True" w1852 {
        tunnel: w1851 -> [w2153 w2210]
        tunnel: w1850 -> [w2152 w2209]
        tunnel: w1835 -> [w2151 w2208]
        tunnel: w1841 -> [w2150 w2207]
        tunnel: [w2149 w2206] -> w1849
        frame True {
          n783 = case shown="False" w2153 {
            tunnel: w2152 -> [w2157 w2183]
            tunnel: w2151 -> [w2156 w2182]
            tunnel: w2150 -> [w2155 w2181]
            tunnel: [w2154 w2180] -> w2149
            frame True {
              n784 = case shown="False" w2157 {
                tunnel: w2156 -> [w2160 w2171]
                tunnel: w2155 -> [w2159 w2170]
                tunnel: [w2158 w2169] -> w2154
                frame True {
                  n785 = case shown="\"L\"" w2160 {
                    tunnel: w2159 -> [w2162 w2166]
                    tunnel: [w2161 w2165] -> w2158
                    frame "L" {
                      n786 = case shown="\"R\", Default" w2162 {
                        tunnel: [7 1] -> w2161
                        frame "R", Default {
                          # "2"
                        }
                        frame "L" {
                        }
                      }
                    }
                    frame "R", Default {
                      n787 = case shown="\"L\"" w2166 {
                        tunnel: [5 6] -> w2165
                        frame "R", Default {
                        }
                        frame "L" {
                        }
                      }
                    }
                  }
                }
                frame False {
                  n788 = case shown="\"R\", Default" w2171 {
                    tunnel: w2170 -> [w2173 w2177]
                    tunnel: [w2172 w2176] -> w2169
                    frame "L" {
                      n789 = case shown="\"L\"" w2173 {
                        tunnel: [12 1] -> w2172
                        frame "R", Default {
                        }
                        frame "L" {
                        }
                      }
                    }
                    frame "R", Default {
                      n790 = case shown="\"L\"" w2177 {
                        tunnel: [3 11] -> w2176
                        frame "R", Default {
                        }
                        frame "L" {
                          # "4"
                        }
                      }
                    }
                  }
                }
              }
            }
            frame False {
              n791 = case shown="False" w2183 {
                tunnel: w2182 -> [w2186 w2197]
                tunnel: w2181 -> [w2185 w2196]
                tunnel: [w2184 w2195] -> w2180
                frame True {
                  n792 = case shown="\"L\"" w2186 {
                    tunnel: w2185 -> [w2188 w2192]
                    tunnel: [w2187 w2191] -> w2184
                    frame "L" {
                      n793 = case shown="\"R\", Default" w2188 {
                        tunnel: [7 7] -> w2187
                        frame "R", Default {
                        }
                        frame "L" {
                        }
                      }
                    }
                    frame "R", Default {
                      n794 = case shown="\"R\", Default" w2192 {
                        tunnel: [5 8] -> w2191
                        frame "R", Default {
                        }
                        frame "L" {
                        }
                      }
                    }
                  }
                }
                frame False {
                  n795 = case shown="\"R\", Default" w2197 {
                    tunnel: w2196 -> [w2199 w2203]
                    tunnel: [w2198 w2202] -> w2195
                    frame "L" {
                      n796 = case shown="\"L\"" w2199 {
                        tunnel: [7 7] -> w2198
                        frame "R", Default {
                        }
                        frame "L" {
                        }
                      }
                    }
                    frame "R", Default {
                      n797 = case shown="\"R\", Default" w2203 {
                        tunnel: [11 11] -> w2202
                        frame "R", Default {
                        }
                        frame "L" {
                        }
                      }
                    }
                  }
                }
              }
            }
          }
        }
        frame False {
          n798 = case shown="False" w2210 {
            tunnel: w2209 -> [w2214 w2240]
            tunnel: w2208 -> [w2213 w2239]
            tunnel: w2207 -> [w2212 w2238]
            tunnel: [w2211 w2237] -> w2206
            frame True {
              n799 = case shown="False" w2214 {
                tunnel: w2213 -> [w2217 w2228]
                tunnel: w2212 -> [w2216 w2227]
                tunnel: [w2215 w2226] -> w2211
                frame True {
                  n800 = case shown="\"L\"" w2217 {
                    tunnel: w2216 -> [w2219 w2223]
                    tunnel: [w2218 w2222] -> w2215
                    frame "L" {
                      n801 = case shown="\"R\", Default" w2219 {
                        tunnel: [7 6] -> w2218
                        frame "R", Default {
                          # "2"
                        }
                        frame "L" {
                        }
                      }
                    }
                    frame "R", Default {
                      n802 = case shown="\"L\"" w2223 {
                        tunnel: [5 6] -> w2222
                        frame "R", Default {
                        }
                        frame "L" {
                        }
                      }
                    }
                  }
                }
                frame False {
                  n803 = case shown="\"R\", Default" w2228 {
                    tunnel: w2227 -> [w2230 w2234]
                    tunnel: [w2229 w2233] -> w2226
                    frame "L" {
                      n804 = case shown="\"R\", Default" w2230 {
                        tunnel: [9 6] -> w2229
                        frame "R", Default {
                        }
                        frame "L" {
                        }
                      }
                    }
                    frame "R", Default {
                      n805 = case shown="\"R\", Default" w2234 {
                        tunnel: [9 6] -> w2233
                        frame "R", Default {
                        }
                        frame "L" {
                        }
                      }
                    }
                  }
                }
              }
            }
            frame False {
              n806 = case shown="False" w2240 {
                tunnel: w2239 -> [w2243 w2254]
                tunnel: w2238 -> [w2242 w2253]
                tunnel: [w2241 w2252] -> w2237
                frame True {
                  n807 = case shown="\"R\", Default" w2243 {
                    tunnel: w2242 -> [w2245 w2249]
                    tunnel: [w2244 w2248] -> w2241
                    frame "L" {
                      n808 = case shown="\"L\"" w2245 {
                        tunnel: [7 8] -> w2244
                        frame "R", Default {
                        }
                        frame "L" {
                        }
                      }
                    }
                    frame "R", Default {
                      n809 = case shown="\"L\"" w2249 {
                        tunnel: [5 8] -> w2248
                        frame "R", Default {
                        }
                        frame "L" {
                        }
                      }
                    }
                  }
                }
                frame False {
                  n810 = case shown="\"L\"" w2254 {
                    tunnel: w2253 -> [w2256 w2260]
                    tunnel: [w2255 w2259] -> w2252
                    frame "L" {
                      n811 = case shown="\"R\", Default" w2256 {
                        tunnel: [10 8] -> w2255
                        frame "R", Default {
                        }
                        frame "L" {
                        }
                      }
                    }
                    frame "R", Default {
                      n812 = case shown="\"R\", Default" w2260 {
                        tunnel: [10 8] -> w2259
                        frame "R", Default {
                        }
                        frame "L" {
                        }
                      }
                    }
                  }
                }
              }
            }
          }
        }
      }
      n813 = global write "Robot Global Data.vi" "Auto Running"(w1849) -> ()
      n814 = global read "Robot Global Data.vi" "Auto Running"() -> (w1847:dbl)
      n815 = case shown="1" w1847 {
        tunnel: w1848 -> [w1856 w1860 w1891 w1930 w1957 w1984 w1993 w2026 w2048 w2063 w2097 w2109 w2129]
        frame -1, Default {
          n816 = call "Auto Drive XY Left Automatic.vi"("RobotDriveDevRef In"=w1856, "Distance (in)"=-150.0) -> ()  [unwired: 13 in, 1 out]
        }
        frame 1 {
          n817 = flat-sequence {
            tunnel: w1860 -> [w1866]
            tunnel: [w1863] -> w1859
            tunnel: w1859 -> [w1872]
            tunnel: [w1868] -> w1858
            tunnel: w1858 -> [w1877]
            tunnel: [w1876] -> w1857
            tunnel: w1857 -> [w1884]
            frame #0 {
              n818 = call "Auto Drive XY Left Automatic.vi"("RobotDriveDevRef In"=w1866, "Movement"=1.0, "Distance (in)"=-170.0, "Time to Settle (ms)"=u32 10, "Motor Output Range Y"=cluster{"output high":dbl, "output low":dbl} {"output high"=0.7, "output low"=-0.75}) -> ("RobotDriveDevRef Out"=w1863:T2)  [unwired: 10 in]
            }
            frame #1 {
              n819 = global write "Robot Global Data.vi" "Intake Speed Override"(-0.5 ("Intake Speed Override")) -> ()
              n820 = call "Auto Drive XY Left Automatic.vi"("RobotDriveDevRef In"=w1872, "Movement"=2.0, "Distance (in)"=300.0, "Time to Settle (ms)"=u32 50) -> ("RobotDriveDevRef Out"=w1868:T2)  [unwired: 11 in]
            }
            frame #2 {
              n821 = global write "Robot Global Data.vi" "Intake Pistons"(WPI_SolenoidValue."Off" ("Intake Pistons")) -> ()
              n822 = call "Auto Drive XY Left Automatic.vi"("RobotDriveDevRef In"=w1877, "Movement"=3.0, "Distance (in)"=-55.0, "Time to Settle (ms)"=u32 500, "Motor Output Range Y"=cluster{"output high":dbl, "output low":dbl} {"output high"=0.7, "output low"=-0.8}) -> ("RobotDriveDevRef Out"=w1876:T2)  [unwired: 10 in]
            }
            frame #3 {
              n823 = global write "Robot Global Data.vi" "Intake Speed Override"(-0.3 ("Arm Angle to Turn to")) -> ()
              n824 = call "Auto Drive XY Left Automatic.vi"("RobotDriveDevRef In"=w1884, "Distance (in)"=20.0) -> ()  [unwired: 13 in, 1 out]
              n825 = global write "Robot Global Data.vi" "Lift Height to rase to (in)"(0.0 ("Arm Angle to Turn to")) -> ()
              n826 = global write "Robot Global Data.vi" "Arm Angle to Turn to"(0.0 ("Arm Angle to Turn to")) -> ()
            }
          }
        }
        frame 2 {
          n827 = flat-sequence {
            tunnel: w1891 -> [w1897]
            tunnel: [w1894] -> w1890
            tunnel: w1890 -> [w1903]
            tunnel: [w1899] -> w1889
            tunnel: w1889 -> [w1909]
            tunnel: [w1908] -> w1887
            tunnel: w1887 -> [w1913]
            tunnel: [w1912] -> w1886
            tunnel: w1886 -> [w1915]
            tunnel: [w1914] -> w1885
            tunnel: w1885 -> [w1918]
            tunnel: [w1919] -> w1888
            tunnel: w1888 -> [w1924]
            frame #0 {
              n828 = call "Auto Drive XY Left Automatic.vi"("RobotDriveDevRef In"=w1897, "Movement"=1.0, "Distance (in)"=-170.0, "Time to Settle (ms)"=u32 10, "Motor Output Range Y"=cluster{"output high":dbl, "output low":dbl} {"output high"=0.7, "output low"=-0.75}) -> ("RobotDriveDevRef Out"=w1894:T2)  [unwired: 10 in]
            }
            frame #1 {
              n829 = global write "Robot Global Data.vi" "Intake Speed Override"(-0.5 ("Intake Speed Override")) -> ()
              n830 = call "Auto Drive XY Left Automatic.vi"("RobotDriveDevRef In"=w1903, "Movement"=2.0, "Distance (in)"=300.0, "Time to Settle (ms)"=u32 50) -> ("RobotDriveDevRef Out"=w1899:T2)  [unwired: 11 in]
            }
            frame #2 {
              n831 = call <vilib>:"WPI_RobotDriveDelayAndUpdateSafety.vi"("Delay (s)"=1.0, "RobotDriveDevRef"=w1909) -> ("RobotDriveDevRef 2"=w1908:T2)  [unwired: 8 in, 1 out]
              n832 = global write "Robot Global Data.vi" "Lift Height to rase to (in)"(40.0 ("Arm Angle to Turn to")) -> ()
              n833 = global write "Robot Global Data.vi" "Arm Angle to Turn to"(500.0 ("Arm Angle to Turn to")) -> ()
              n834 = global write "Robot Global Data.vi" "Intake Pistons"(WPI_SolenoidValue."Off" ("Intake Pistons")) -> ()
            }
            frame #3 {
              n835 = call-poly <vilib>:"WPI_RobotDriveArcadeDrive.vi"("Y axis value"=0.6, "X axis value"=0.0, "RobotDriveDevRef"=w1913) -> ("RobotDriveDevRef"=w1912:T2)  [unwired: 6 in, 2 out]
            }
            frame #4 {
              n836 = call <vilib>:"WPI_RobotDriveDelayAndUpdateSafety.vi"("Delay (s)"=0.25, "RobotDriveDevRef"=w1915) -> ("RobotDriveDevRef 2"=w1914:T2)  [unwired: 8 in, 1 out]
            }
            frame #5 {
              n837 = call <vilib>:"WPI_RobotDriveDelayAndUpdateSafety.vi"("Delay (s)"=1.0, "RobotDriveDevRef"=w1918) -> ("RobotDriveDevRef 2"=w1919:T2)  [unwired: 8 in, 1 out]
              n838 = global write "Robot Global Data.vi" "Intake Speed Override"(-0.8 ("Arm Angle to Turn to")) -> ()
            }
            frame #6 {
              n839 = global write "Robot Global Data.vi" "Intake Speed Override"(0.0 ("Intake Speed Override")) -> ()
              n840 = global write "Robot Global Data.vi" "Lift Height to rase to (in)"(0.0 ("Arm Angle to Turn to")) -> ()
              n841 = global write "Robot Global Data.vi" "Arm Angle to Turn to"(0.0 ("Arm Angle to Turn to")) -> ()
              n842 = call "Auto Drive XY Left Automatic.vi"("RobotDriveDevRef In"=w1924, "Movement"=3.0, "Distance (in)"=-30.0) -> ()  [unwired: 12 in, 1 out]
            }
          }
        }
        frame 3 {
          n843 = flat-sequence {
            tunnel: w1930 -> [w1935]
            tunnel: [w1932] -> w1929
            tunnel: w1929 -> [w1942]
            tunnel: [w1939] -> w1928
            tunnel: w1928 -> [w1945]
            tunnel: [w1944] -> w1927
            tunnel: w1927 -> [w1951]
            frame #0 {
              n844 = call "Auto Drive XY Left Automatic.vi"("RobotDriveDevRef In"=w1935, "Movement"=1.0, "Distance (in)"=-1000.0, "Motor Output Range Y"=cluster{"output high":dbl, "output low":dbl} {"output high"=0.85, "output low"=-0.95}) -> ("RobotDriveDevRef Out"=w1932:T2)  [unwired: 11 in]
            }
            frame #1 {
              n845 = global write "Robot Global Data.vi" "Intake Speed Override"(-0.5 ("Arm Angle to Turn to")) -> ()
              n846 = call "Auto Drive XY Left Automatic.vi"("RobotDriveDevRef In"=w1942, "Movement"=2.0, "Distance (in)"=150.0, "Time to Settle (ms)"=u32 150, "Motor Output Range Y"=cluster{"output high":dbl, "output low":dbl} {"output high"=0.75, "output low"=-0.7}) -> ("RobotDriveDevRef Out"=w1939:T2)  [unwired: 10 in]
            }
            frame #2 {
              n847 = call "Auto Drive XY Left Automatic.vi"("RobotDriveDevRef In"=w1945, "Movement"=3.0, "Distance (in)"=-60.0) -> ("RobotDriveDevRef Out"=w1944:T2)  [unwired: 12 in]
              n848 = global write "Robot Global Data.vi" "Intake Pistons"(WPI_SolenoidValue."Off" ("Intake Pistons")) -> ()
            }
            frame #3 {
              n849 = call "Auto Drive XY Left Automatic.vi"("RobotDriveDevRef In"=w1951, "Distance (in)"=25.0) -> ()  [unwired: 13 in, 1 out]
              n850 = global write "Robot Global Data.vi" "Intake Speed Override"(0.0 ("Arm Angle to Turn to")) -> ()
              n851 = global write "Robot Global Data.vi" "Lift Height to rase to (in)"(0.0 ("Arm Angle to Turn to")) -> ()
              n852 = global write "Robot Global Data.vi" "Arm Angle to Turn to"(0.0 ("Arm Angle to Turn to")) -> ()
            }
          }
        }
        frame 4 {
          n853 = flat-sequence {
            tunnel: w1957 -> [w1962]
            tunnel: [w1959] -> w1956
            tunnel: w1956 -> [w1969]
            tunnel: [w1966] -> w1955
            tunnel: w1955 -> [w1975]
            tunnel: [w1974] -> w1954
            tunnel: w1954 -> [w1979]
            tunnel: [w1978] -> w1953
            tunnel: w1953 -> [w1982]
            frame #0 {
              n854 = call "Auto Drive XY Left Automatic.vi"("RobotDriveDevRef In"=w1962, "Movement"=1.0, "Distance (in)"=-1000.0, "Motor Output Range Y"=cluster{"output high":dbl, "output low":dbl} {"output high"=0.85, "output low"=-0.95}) -> ("RobotDriveDevRef Out"=w1959:T2)  [unwired: 11 in]
            }
            frame #1 {
              n855 = global write "Robot Global Data.vi" "Intake Speed Override"(-0.5 ("Arm Angle to Turn to")) -> ()
              n856 = call "Auto Drive XY Left Automatic.vi"("RobotDriveDevRef In"=w1969, "Movement"=2.0, "Distance (in)"=150.0, "Time to Settle (ms)"=u32 150, "Motor Output Range Y"=cluster{"output high":dbl, "output low":dbl} {"output high"=0.75, "output low"=-0.7}) -> ("RobotDriveDevRef Out"=w1966:T2)  [unwired: 10 in]
            }
            frame #2 {
              n857 = call <vilib>:"WPI_RobotDriveDelayAndUpdateSafety.vi"("Delay (s)"=0.5, "RobotDriveDevRef"=w1975) -> ("RobotDriveDevRef 2"=w1974:T2)  [unwired: 8 in, 1 out]
              n858 = global write "Robot Global Data.vi" "Lift Height to rase to (in)"(30.0 ("Arm Angle to Turn to")) -> ()
              n859 = global write "Robot Global Data.vi" "Arm Angle to Turn to"(500.0 ("Arm Angle to Turn to")) -> ()
              n860 = global write "Robot Global Data.vi" "Intake Pistons"(WPI_SolenoidValue."Off" ("Intake Pistons")) -> ()
            }
            frame #3 {
              n861 = call <vilib>:"WPI_RobotDriveDelayAndUpdateSafety.vi"("Delay (s)"=1.0, "RobotDriveDevRef"=w1979) -> ("RobotDriveDevRef 2"=w1978:T2)  [unwired: 8 in, 1 out]
              n862 = global write "Robot Global Data.vi" "Intake Speed Override"(1.0 ("Arm Angle to Turn to")) -> ()
            }
            frame #4 {
              n863 = global write "Robot Global Data.vi" "Arm Angle to Turn to"(0.0 ("Arm Angle to Turn to")) -> ()
              n864 = global write "Robot Global Data.vi" "Lift Height to rase to (in)"(0.0 ("Arm Angle to Turn to")) -> ()
              n865 = call "Auto Drive XY Left Automatic.vi"("RobotDriveDevRef In"=w1982, "Distance (in)"=30.0) -> ()  [unwired: 13 in, 1 out]
            }
          }
        }
        frame 5 {
          n866 = flat-sequence {
            tunnel: w1984 -> [w1987]
            frame #0 {
              n867 = call "Auto Drive XY Left Automatic.vi"("RobotDriveDevRef In"=w1987, "Movement"=1.0, "Distance (in)"=-250.0) -> ()  [unwired: 12 in, 1 out]
            }
            frame #1 {
              n868 = global write "Robot Global Data.vi" "Lift Height to rase to (in)"(0.0 ("Arm Angle to Turn to")) -> ()
              n869 = global write "Robot Global Data.vi" "Arm Angle to Turn to"(0.0 ("Arm Angle to Turn to")) -> ()
            }
          }
        }
        frame 6 {
          n870 = flat-sequence {
            tunnel: w1993 -> [w1999]
            tunnel: [w1996] -> w1992
            tunnel: w1992 -> [w2009]
            tunnel: [w2004] -> w1991
            tunnel: w1991 -> [w2015]
            tunnel: [w2010] -> w1990
            tunnel: w1990 -> [w2021]
            frame #0 {
              n871 = call "Auto Drive XY Right Automatic.vi"("RobotDriveDevRef In"=w1999, "Movement"=1.0, "Motor Output Range X"=cluster{"output high":dbl, "output low":dbl} {"output high"=0.8, "output low"=-0.8}, "Distance (in)"=-270.0, "Motor Output Range Y"=cluster{"output high":dbl, "output low":dbl} {"output high"=0.7, "output low"=-0.8}) -> ("RobotDriveDevRef Out"=w1996:T2)  [unwired: 10 in]
            }
            frame #1 {
              n872 = global write "Robot Global Data.vi" "Lift Height to rase to (in)"(0.0 ("Arm Angle to Turn to")) -> ()
              n873 = global write "Robot Global Data.vi" "Intake Speed Override"(-0.5 ("Arm Angle to Turn to")) -> ()
              n874 = global write "Robot Global Data.vi" "Arm Angle to Turn to"(0.0 ("Arm Angle to Turn to")) -> ()
              n875 = global write "Robot Global Data.vi" "Auto Arm Fast"(TRUE ("Lift Down Fast")) -> ()
              n876 = global write "Robot Global Data.vi" "Lift Down Fast"(TRUE ("Lift Down Fast")) -> ()
              n877 = call "Auto Drive XY Right Automatic.vi"("RobotDriveDevRef In"=w2009, "Angle Offset"=100.0, "Movement"=2.0, "Distance (in)"=77.0) -> ("RobotDriveDevRef Out"=w2004:T2)  [unwired: 11 in]
            }
            frame #2 {
              n878 = global write "Robot Global Data.vi" "Auto Arm Fast"(FALSE ("Lift Down Fast")) -> ()
              n879 = global write "Robot Global Data.vi" "Lift Down Fast"(FALSE ("Lift Down Fast")) -> ()
              n880 = call "Auto Drive XY Right Automatic.vi"("RobotDriveDevRef In"=w2015, "Movement"=3.0, "Distance (in)"=-65.0) -> ("RobotDriveDevRef Out"=w2010:T2)  [unwired: 12 in]
              n881 = global write "Robot Global Data.vi" "Intake Pistons"(WPI_SolenoidValue."Off" ("Intake Pistons")) -> ()
            }
            frame #3 {
              n882 = global write "Robot Global Data.vi" "Lift Height to rase to (in)"(0.0 ("Arm Angle to Turn to")) -> ()
              n883 = global write "Robot Global Data.vi" "Intake Speed Override"(1.0 ("Intake Speed Override")) -> ()
              n884 = global write "Robot Global Data.vi" "Arm Angle to Turn to"(0.0 ("Arm Angle to Turn to")) -> ()
              n885 = global write "Robot Global Data.vi" "Intake Pistons"(WPI_SolenoidValue."On" ("Intake Pistons")) -> ()
              n886 = call "Auto Drive XY Right Automatic.vi"("RobotDriveDevRef In"=w2021, "Angle Offset"=45.0, "Distance (in)"=70.0) -> ()  [unwired: 12 in, 1 out]
            }
          }
        }
        frame 7 {
          n887 = flat-sequence {
            tunnel: [w2029] -> w2027
            tunnel: w2026 -> [w2028]
            tunnel: w2027 -> [w2035]
            tunnel: [w2034] -> w2025
            tunnel: w2025 -> [w2044]
            tunnel: [w2043] -> w2024
            tunnel: [w2046] -> _
            tunnel: w2024 -> [w2046]
            frame #0 {
              n888 = call "Auto Drive XY Left Automatic.vi"("RobotDriveDevRef In"=w2028, "Movement"=1.0, "Distance (in)"=-170.0, "Time to Settle (ms)"=u32 10, "Motor Output Range Y"=cluster{"output high":dbl, "output low":dbl} {"output high"=0.7, "output low"=-0.75}) -> ("RobotDriveDevRef Out"=w2029:T2)  [unwired: 10 in]
            }
            frame #1 {
              n889 = global write "Robot Global Data.vi" "Intake Speed Override"(-0.5 ("Intake Speed Override")) -> ()
              n890 = call "Auto Drive XY Left Automatic.vi"("RobotDriveDevRef In"=w2035, "Movement"=2.0, "Distance (in)"=300.0, "Time to Settle (ms)"=u32 50) -> ("RobotDriveDevRef Out"=w2034:T2)  [unwired: 11 in]
            }
            frame #2 {
              n891 = call "Auto Drive XY Left Automatic.vi"("RobotDriveDevRef In"=w2044, "Angle Offset"=-90.0, "Distance (in)"=-70.0) -> ("RobotDriveDevRef Out"=w2043:T2)  [unwired: 12 in]
              n892 = global write "Robot Global Data.vi" "Intake Pistons"(WPI_SolenoidValue."Off" ("Intake Pistons")) -> ()
            }
            frame #3 {
              n893 = global write "Robot Global Data.vi" "Intake Speed Override"(0.0 ("Intake Speed Override")) -> ()
            }
          }
        }
        frame 8 {
          n894 = flat-sequence {
            tunnel: w2048 -> [w2049]
            tunnel: [w2050] -> w2047
            tunnel: w2047 -> [w2055]
            frame #0 {
              n895 = call "Auto Drive XY Left Automatic.vi"("RobotDriveDevRef In"=w2049, "Movement"=1.0, "Motor Output Range X"=cluster{"output high":dbl, "output low":dbl} {"output high"=0.8, "output low"=-0.8}, "Distance (in)"=-270.0, "Motor Output Range Y"=cluster{"output high":dbl, "output low":dbl} {"output high"=0.7, "output low"=-0.8}) -> ("RobotDriveDevRef Out"=w2050:T2)  [unwired: 10 in]
            }
            frame #1 {
              n896 = global write "Robot Global Data.vi" "Arm Angle to Turn to"(0.0 ("Arm Angle to Turn to")) -> ()
              n897 = global write "Robot Global Data.vi" "Lift Height to rase to (in)"(0.0 ("Arm Angle to Turn to")) -> ()
              n898 = call "Auto Drive XY Left Automatic.vi"("RobotDriveDevRef In"=w2055, "Distance (in)"=30.0) -> ()  [unwired: 13 in, 1 out]
            }
          }
        }
        frame 9 {
          n899 = flat-sequence {
            tunnel: w2063 -> [w2068]
            tunnel: [w2065] -> w2062
            tunnel: w2062 -> [w2075]
            tunnel: [w2074] -> w2061
            tunnel: w2061 -> [w2082]
            tunnel: [w2081] -> w2060
            tunnel: w2060 -> [w2088]
            tunnel: [w2087] -> w2059
            tunnel: w2059 -> [w2094]
            frame #0 {
              n900 = call "Auto Drive XY Left Automatic.vi"("RobotDriveDevRef In"=w2068, "Movement"=1.0, "Distance (in)"=-406.0, "Motor Output Range Y"=cluster{"output high":dbl, "output low":dbl} {"output high"=0.7, "output low"=-0.9}) -> ("RobotDriveDevRef Out"=w2065:T2)  [unwired: 11 in]
            }
            frame #1 {
              n901 = global write "Robot Global Data.vi" "Intake Speed Override"(-0.1 ("Arm Angle to Turn to")) -> ()
              n902 = call "Auto Drive XY Left Automatic.vi"("RobotDriveDevRef In"=w2075, "Angle Offset"=10.0, "Movement"=2.0, "Distance (in)"=80.0, "Motor Output Range Y"=cluster{"output high":dbl, "output low":dbl} {"output high"=0.6, "output low"=-0.7}) -> ("RobotDriveDevRef Out"=w2074:T2)  [unwired: 10 in]
              n903 = global write "Robot Global Data.vi" "Lift Down Fast"(TRUE ("Lift Down Fast")) -> ()
              n904 = global write "Robot Global Data.vi" "Auto Arm Fast"(TRUE ("Lift Down Fast")) -> ()
            }
            frame #2 {
              n905 = global write "Robot Global Data.vi" "Intake Pistons"(WPI_SolenoidValue."Off" ("Intake Pistons")) -> ()
              n906 = global write "Robot Global Data.vi" "Auto Arm Fast"(FALSE ("Lift Down Fast")) -> ()
              n907 = call "Auto Drive XY Left Automatic.vi"("RobotDriveDevRef In"=w2082, "Angle Offset"=-7.0, "Movement"=3.0, "Distance (in)"=-53.0) -> ("RobotDriveDevRef Out"=w2081:T2)  [unwired: 11 in]
            }
            frame #3 {
              n908 = global write "Robot Global Data.vi" "Lift Height to rase to (in)"(0.0 ("Arm Angle to Turn to")) -> ()
              n909 = global write "Robot Global Data.vi" "Arm Angle to Turn to"(0.0 ("Arm Angle to Turn to")) -> ()
              n910 = global write "Robot Global Data.vi" "Auto Arm Fast"(TRUE ("Lift Down Fast")) -> ()
              n911 = call <vilib>:"WPI_RobotDriveDelayAndUpdateSafety.vi"("Delay (s)"=0.5, "RobotDriveDevRef"=w2088) -> ("RobotDriveDevRef 2"=w2087:T2)  [unwired: 8 in, 1 out]
            }
            frame #4 {
              n912 = global write "Robot Global Data.vi" "Intake Speed Override"(1.0 ("Arm Angle to Turn to")) -> ()
              n913 = call "Auto Drive XY Left Automatic.vi"("RobotDriveDevRef In"=w2094, "Angle Offset"=30.0, "Distance (in)"=70.0) -> ()  [unwired: 12 in, 1 out]
              n914 = global write "Robot Global Data.vi" "Intake Pistons"(WPI_SolenoidValue."On" ("Intake Pistons")) -> ()
            }
          }
        }
        frame 10 {
          n915 = flat-sequence {
            tunnel: w2097 -> [w2099]
            tunnel: [w2098] -> w2096
            tunnel: w2096 -> [w2103]
            frame #0 {
              n916 = call "Auto Drive XY Left Automatic.vi"("RobotDriveDevRef In"=w2099, "Movement"=1.0, "Distance (in)"=-406.0, "Motor Output Range Y"=cluster{"output high":dbl, "output low":dbl} {"output high"=0.7, "output low"=-0.9}) -> ("RobotDriveDevRef Out"=w2098:T2)  [unwired: 11 in]
            }
            frame #1 {
              n917 = global write "Robot Global Data.vi" "Arm Angle to Turn to"(0.0 ("Arm Angle to Turn to")) -> ()
              n918 = global write "Robot Global Data.vi" "Lift Height to rase to (in)"(0.0 ("Arm Angle to Turn to")) -> ()
              n919 = call "Auto Drive XY Left Automatic.vi"("RobotDriveDevRef In"=w2103, "Distance (in)"=30.0) -> ()  [unwired: 13 in, 1 out]
            }
          }
        }
        frame 11 {
          n920 = flat-sequence {
            tunnel: w2109 -> [w2114]
            tunnel: [w2111] -> w2108
            tunnel: w2108 -> [w2121]
            tunnel: [w2115] -> w2107
            tunnel: w2107 -> [w2123]
            frame #0 {
              n921 = call "Auto Drive XY Left Automatic.vi"("RobotDriveDevRef In"=w2114, "Movement"=1.0, "Distance (in)"=-1000.0, "Motor Output Range Y"=cluster{"output high":dbl, "output low":dbl} {"output high"=0.85, "output low"=-0.95}) -> ("RobotDriveDevRef Out"=w2111:T2)  [unwired: 11 in]
            }
            frame #1 {
              n922 = global write "Robot Global Data.vi" "Intake Speed Override"(-0.5 ("Arm Angle to Turn to")) -> ()
              n923 = call "Auto Drive XY Left Automatic.vi"("RobotDriveDevRef In"=w2121, "Movement"=2.0, "Distance (in)"=150.0, "Time to Settle (ms)"=u32 150, "Motor Output Range Y"=cluster{"output high":dbl, "output low":dbl} {"output high"=0.75, "output low"=-0.7}) -> ("RobotDriveDevRef Out"=w2115:T2)  [unwired: 10 in]
            }
            frame #2 {
              n924 = global write "Robot Global Data.vi" "Arm Angle to Turn to"(0.0 ("Arm Angle to Turn to")) -> ()
              n925 = global write "Robot Global Data.vi" "Lift Height to rase to (in)"(0.0 ("Arm Angle to Turn to")) -> ()
              n926 = call "Auto Drive XY Left Automatic.vi"("RobotDriveDevRef In"=w2123, "Distance (in)"=-20.0) -> ()  [unwired: 13 in, 1 out]
              n927 = global write "Robot Global Data.vi" "Intake Pistons"(WPI_SolenoidValue."Off" ("Intake Pistons")) -> ()
            }
          }
        }
        frame 12 {
          n928 = flat-sequence {
            tunnel: w2129 -> [w2135]
            tunnel: [w2132] -> w2128
            tunnel: w2128 -> [w2141]
            tunnel: [w2137] -> w2127
            tunnel: w2127 -> [w2146]
            frame #0 {
              n929 = call "Auto Drive XY Left Automatic.vi"("RobotDriveDevRef In"=w2135, "Movement"=1.0, "Distance (in)"=-170.0, "Time to Settle (ms)"=u32 10, "Motor Output Range Y"=cluster{"output high":dbl, "output low":dbl} {"output high"=0.7, "output low"=-0.95}) -> ("RobotDriveDevRef Out"=w2132:T2)  [unwired: 10 in]
            }
            frame #1 {
              n930 = global write "Robot Global Data.vi" "Intake Speed Override"(-0.5 ("Intake Speed Override")) -> ()
              n931 = call "Auto Drive XY Left Automatic.vi"("RobotDriveDevRef In"=w2141, "Movement"=2.0, "Distance (in)"=300.0, "Time to Settle (ms)"=u32 50) -> ("RobotDriveDevRef Out"=w2137:T2)  [unwired: 11 in]
            }
            frame #2 {
              n932 = global write "Robot Global Data.vi" "Intake Pistons"(WPI_SolenoidValue."Off" ("Intake Pistons")) -> ()
              n933 = call "Auto Drive XY Left Automatic.vi"("RobotDriveDevRef In"=w2146, "Angle Offset"=90.0, "Movement"=3.0, "Motor Output Range X"=cluster{"output high":dbl, "output low":dbl} {"output high"=0.9, "output low"=-0.9}, "Distance (in)"=-160.0, "Motor Output Range Y"=cluster{"output high":dbl, "output low":dbl} {"output high"=0.7, "output low"=-0.9}) -> ()  [unwired: 9 in, 1 out]
            }
          }
        }
      }
    }
    frame "Right Switch" {
      n934 = call <vilib>:"WPI_RobotDriveDelayAndUpdateSafety.vi"("Delay (s)"=0.125, "RobotDriveDevRef"=w2265) -> ("RobotDriveDevRef 2"=w2263:T2)  [unwired: 8 in, 1 out]
      n935 = case shown="\"R\"" w2264 {
        tunnel: w2263 -> [w2267 w2295]
        frame "L", Default {
          n936 = flat-sequence {
            tunnel: w2267 -> [w2276]
            tunnel: [w2273] -> w2270
            tunnel: w2270 -> [w2282]
            tunnel: [w2278] -> w2269
            tunnel: w2269 -> [w2287]
            tunnel: [w2286] -> w2268
            tunnel: w2268 -> [w2294]
            frame #0 {
              n937 = call "Auto Drive XY Right Automatic.vi"("RobotDriveDevRef In"=w2276, "Movement"=1.0, "Distance (in)"=-170.0, "Time to Settle (ms)"=u32 10, "Motor Output Range Y"=cluster{"output high":dbl, "output low":dbl} {"output high"=0.7, "output low"=-0.75}) -> ("RobotDriveDevRef Out"=w2273:T2)  [unwired: 10 in]
            }
            frame #1 {
              n938 = global write "Robot Global Data.vi" "Intake Speed Override"(-0.5 ("Intake Speed Override")) -> ()
              n939 = call "Auto Drive XY Right Automatic.vi"("RobotDriveDevRef In"=w2282, "Movement"=2.0, "Distance (in)"=300.0, "Time to Settle (ms)"=u32 100) -> ("RobotDriveDevRef Out"=w2278:T2)  [unwired: 11 in]
            }
            frame #2 {
              n940 = global write "Robot Global Data.vi" "Intake Pistons"(WPI_SolenoidValue."Off" ("Intake Pistons")) -> ()
              n941 = call "Auto Drive XY Right Automatic.vi"("RobotDriveDevRef In"=w2287, "Movement"=3.0, "Distance (in)"=-55.0, "Time to Settle (ms)"=u32 500, "Motor Output Range Y"=cluster{"output high":dbl, "output low":dbl} {"output high"=0.7, "output low"=-0.8}) -> ("RobotDriveDevRef Out"=w2286:T2)  [unwired: 10 in]
            }
            frame #3 {
              n942 = global write "Robot Global Data.vi" "Intake Speed Override"(-0.3 ("Arm Angle to Turn to")) -> ()
              n943 = call "Auto Drive XY Right Automatic.vi"("RobotDriveDevRef In"=w2294, "Distance (in)"=20.0) -> ()  [unwired: 13 in, 1 out]
              n944 = global write "Robot Global Data.vi" "Lift Height to rase to (in)"(0.0 ("Arm Angle to Turn to")) -> ()
              n945 = global write "Robot Global Data.vi" "Arm Angle to Turn to"(0.0 ("Arm Angle to Turn to")) -> ()
            }
          }
        }
        frame "R" {
          n946 = flat-sequence {
            tunnel: w2295 -> [w2299]
            frame #0 {
              n947 = call "Auto Drive XY Right Automatic.vi"("RobotDriveDevRef In"=w2299, "Distance (in)"=-120.0, "Time to Settle (ms)"=u32 250, "Min Time (ms)"=u32 500) -> ()  [unwired: 11 in, 1 out]
            }
          }
        }
      }
    }
    frame "Center Switch Multi Cube" {
      n948 = call <vilib>:"WPI_RobotDriveDelayAndUpdateSafety.vi"("Delay (s)"=0.125, "RobotDriveDevRef"=w2301) -> ("RobotDriveDevRef 2"=w2300:T2)  [unwired: 8 in, 1 out]
      n949 = case shown="\"L\"" w2303 {
        tunnel: w2300 -> [w2308 w2359]
        frame "L" {
          n950 = flat-sequence {
            tunnel: w2308 -> [w2314]
            tunnel: [w2313] -> w2307
            tunnel: w2307 -> [w2327]
            tunnel: [w2326] -> w2306
            tunnel: w2306 -> [w2335]
            tunnel: [w2334] -> w2305
            tunnel: w2305 -> [w2338]
            tunnel: [w2337] -> w2304
            tunnel: w2304 -> [w2348]
            frame #0 {
              n951 = call "Auto Drive XY Center Switch.vi"("RobotDriveDevRef In"=w2314, "Movement"=1.0, "Distance (in)"=-200.0, "Min Time (ms)"=u32 250, "Motor Output Range Y"=cluster{"output high":dbl, "output low":dbl} {"output high"=0.7, "output low"=-0.9}) -> ("RobotDriveDevRef Out"=w2313:T2)  [unwired: 10 in]
            }
            frame #1 {
              n952 = global write "Robot Global Data.vi" "Lift Height to rase to (in)"(0.0 ("Lift Height to rase to (in)")) -> ()
              n953 = global write "Robot Global Data.vi" "Intake Speed Override"(-0.9 ("Intake Speed Override")) -> ()
              n954 = global write "Robot Global Data.vi" "Arm Angle to Turn to"(0.0 ("Lift Height to rase to (in)")) -> ()
              n955 = global write "Robot Global Data.vi" "Auto Arm Fast"(TRUE ("Auto Arm Fast")) -> ()
              n956 = global write "Robot Global Data.vi" "Intake Pistons"(WPI_SolenoidValue."On" ("Intake Pistons")) -> ()
              n957 = call "Auto Drive XY Center Switch.vi"("RobotDriveDevRef In"=w2327, "Angle Offset"=-115.0, "Movement"=2.0, "Distance (in)"=25.0, "Time to Settle (ms)"=u32 150, "Min Time (ms)"=u32 750, "Motor Output Range Y"=cluster{"output high":dbl, "output low":dbl} {"output high"=0.6, "output low"=-0.7}) -> ("RobotDriveDevRef Out"=w2326:T2)  [unwired: 8 in]
            }
            frame #2 {
              n958 = call "Auto Drive XY Center Switch.vi"("RobotDriveDevRef In"=w2335, "Angle Offset"=115.0, "Movement"=3.0, "Distance (in)"=-130.0, "Motor Output Range Y"=cluster{"output high":dbl, "output low":dbl} {"output high"=0.7, "output low"=-0.7}) -> ("RobotDriveDevRef Out"=w2334:T2)  [unwired: 10 in]
              n959 = global write "Robot Global Data.vi" "Auto Arm Fast"(FALSE ("Auto Arm Fast")) -> ()
              n960 = global write "Robot Global Data.vi" "Intake Pistons"(WPI_SolenoidValue."Off" ("Intake Pistons")) -> ()
            }
            frame #3 {
              n961 = global write "Robot Global Data.vi" "Lift Height to rase to (in)"(0.0 ("Lift Height to rase to (in)")) -> ()
              n962 = global write "Robot Global Data.vi" "Intake Speed Override"(-0.9 ("Intake Speed Override")) -> ()
              n963 = global write "Robot Global Data.vi" "Arm Angle to Turn to"(0.0 ("Lift Height to rase to (in)")) -> ()
              n964 = global write "Robot Global Data.vi" "Auto Arm Fast"(TRUE ("Auto Arm Fast")) -> ()
              n965 = global write "Robot Global Data.vi" "Intake Pistons"(WPI_SolenoidValue."On" ("Intake Pistons")) -> ()
              n966 = call "Auto Drive XY Center Switch.vi"("RobotDriveDevRef In"=w2338, "Angle Offset"=-115.0, "Movement"=2.0, "Distance (in)"=30.0, "Time to Settle (ms)"=u32 150, "Motor Output Range Y"=cluster{"output high":dbl, "output low":dbl} {"output high"=0.6, "output low"=-0.7}) -> ("RobotDriveDevRef Out"=w2337:T2)  [unwired: 9 in]
            }
            frame #4 {
              n967 = call "Auto Drive XY Center Switch.vi"("RobotDriveDevRef In"=w2348, "Angle Offset"=90.0, "Movement"=3.0, "Distance (in)"=-150.0, "Motor Output Range Y"=cluster{"output high":dbl, "output low":dbl} {"output high"=0.7, "output low"=-0.7}) -> ()  [unwired: 10 in, 1 out]
              n968 = global write "Robot Global Data.vi" "Auto Arm Fast"(FALSE ("Auto Arm Fast")) -> ()
              n969 = global write "Robot Global Data.vi" "Intake Pistons"(WPI_SolenoidValue."Off" ("Intake Pistons")) -> ()
            }
          }
        }
        frame "R", Default {
          n970 = flat-sequence {
            tunnel: w2359 -> [w2365]
            tunnel: [w2364] -> w2358
            tunnel: w2358 -> [w2376]
            tunnel: [w2375] -> w2357
            tunnel: w2357 -> [w2384]
            tunnel: [w2383] -> w2356
            tunnel: w2356 -> [w2386]
            tunnel: [w2385] -> w2355
            tunnel: w2355 -> [w2396]
            frame #0 {
              n971 = call "Auto Drive XY Center Switch.vi"("RobotDriveDevRef In"=w2365, "Movement"=1.0, "Distance (in)"=-200.0, "Min Time (ms)"=u32 250, "Motor Output Range Y"=cluster{"output high":dbl, "output low":dbl} {"output high"=0.7, "output low"=-0.9}) -> ("RobotDriveDevRef Out"=w2364:T2)  [unwired: 10 in]
            }
            frame #1 {
              n972 = global write "Robot Global Data.vi" "Lift Height to rase to (in)"(0.0 ("Lift Height to rase to (in)")) -> ()
              n973 = global write "Robot Global Data.vi" "Intake Speed Override"(-0.9 ("Intake Speed Override")) -> ()
              n974 = global write "Robot Global Data.vi" "Arm Angle to Turn to"(0.0 ("Lift Height to rase to (in)")) -> ()
              n975 = global write "Robot Global Data.vi" "Auto Arm Fast"(TRUE ("Auto Arm Fast")) -> ()
              n976 = global write "Robot Global Data.vi" "Intake Pistons"(WPI_SolenoidValue."On" ("Intake Pistons")) -> ()
              n977 = call "Auto Drive XY Center Switch.vi"("RobotDriveDevRef In"=w2376, "Angle Offset"=115.0, "Movement"=2.0, "Distance (in)"=90.0, "Motor Output Range Y"=cluster{"output high":dbl, "output low":dbl} {"output high"=0.6, "output low"=-0.7}) -> ("RobotDriveDevRef Out"=w2375:T2)  [unwired: 10 in]
            }
            frame #2 {
              n978 = call "Auto Drive XY Center Switch.vi"("RobotDriveDevRef In"=w2384, "Angle Offset"=-115.0, "Movement"=3.0, "Distance (in)"=-90.0, "Motor Output Range Y"=cluster{"output high":dbl, "output low":dbl} {"output high"=0.7, "output low"=-0.7}) -> ("RobotDriveDevRef Out"=w2383:T2)  [unwired: 10 in]
              n979 = global write "Robot Global Data.vi" "Auto Arm Fast"(FALSE ("Auto Arm Fast")) -> ()
              n980 = global write "Robot Global Data.vi" "Intake Pistons"(WPI_SolenoidValue."Off" ("Intake Pistons")) -> ()
            }
            frame #3 {
              n981 = global write "Robot Global Data.vi" "Lift Height to rase to (in)"(0.0 ("Lift Height to rase to (in)")) -> ()
              n982 = global write "Robot Global Data.vi" "Intake Speed Override"(-0.2 ("Intake Speed Override")) -> ()
              n983 = global write "Robot Global Data.vi" "Arm Angle to Turn to"(0.0 ("Lift Height to rase to (in)")) -> ()
              n984 = global write "Robot Global Data.vi" "Auto Arm Fast"(TRUE ("Auto Arm Fast")) -> ()
              n985 = global write "Robot Global Data.vi" "Intake Pistons"(WPI_SolenoidValue."On" ("Intake Pistons")) -> ()
              n986 = call "Auto Drive XY Center Switch.vi"("RobotDriveDevRef In"=w2386, "Angle Offset"=145.0, "Movement"=2.0, "Distance (in)"=90.0, "Motor Output Range Y"=cluster{"output high":dbl, "output low":dbl} {"output high"=0.6, "output low"=-0.7}) -> ("RobotDriveDevRef Out"=w2385:T2)  [unwired: 10 in]
            }
            frame #4 {
              n987 = call "Auto Drive XY Center Switch.vi"("RobotDriveDevRef In"=w2396, "Angle Offset"=-45.0, "Movement"=4.0, "Distance (in)"=-140.0, "Motor Output Range Y"=cluster{"output high":dbl, "output low":dbl} {"output high"=0.7, "output low"=-0.7}) -> ()  [unwired: 10 in, 1 out]
              n988 = global write "Robot Global Data.vi" "Auto Arm Fast"(FALSE ("Auto Arm Fast")) -> ()
              n989 = global write "Robot Global Data.vi" "Intake Pistons"(WPI_SolenoidValue."Off" ("Intake Pistons")) -> ()
            }
          }
        }
      }
    }
    frame "Basic Left" {
      n990 = case shown="\"L\"" w2403 {
        tunnel: w2404 -> [w2406 w2460]
        frame "R", Default {
          n991 = flat-sequence {
            tunnel: w2406 -> [w2408]
            tunnel: [w2407] -> w2405
            tunnel: w2405 -> [w2434]
            frame #0 {
              n992 = Tick Count (ms)() -> (millisecond timer value=w2409:u32)
              n993 = global read "Robot Global Data.vi" "Left Drive Encoder Distance"() -> (w2410:dbl)
              n994 = while {
                tunnel: w2408 -> [w2423]
                tunnel: w2410 -> [w2414]
                tunnel: w2409 -> [w2412]
                tunnel: [w2411] -> w2407
                stop <- w2416 stop-if-true
                n995 = global read "Robot Global Data.vi" "Left Drive Encoder Distance"() -> (w2415:dbl)
                n996 = global read "Robot Global Data.vi" "Left Drive Encoder Stopped"() -> (w2419:bool)
                n997 = Subtract(x=w2415, y=w2414) -> (x-y=w2413:dbl)
                n998 = call-poly <vilib>:"PID.vi"("output range"=cluster{"output high":dbl, "output low":dbl} {"output high"=0.7, "output low"=-0.7}, "PID gains"=T8 {"proportional gain (Kc)"=0.07, "integral time (Ti, min)"=0.0, "derivative time (Td, min)"=0.0} ("PID gains 4"), "process variable"=w2413, "setpoint"=200.0) -> ("output"=w2420:dbl)  [unwired: 6 in, 1 out]
                n999 = feedback #9(w2412) -> (w2417:u32)
                n1000 = case shown="True" w2419 {
                  tunnel: w2417 -> [_ w2432]
                  tunnel: [w2428 w2432] -> w2418
                  tunnel: [FALSE w2429] -> w2416
                  frame False {
                    n1001 = Tick Count (ms)() -> (millisecond timer value=w2428:u32)
                  }
                  frame True {
                    n1002 = Tick Count (ms)() -> (millisecond timer value=w2433:u32)
                    n1003 = Subtract(x=w2433, y=w2432) -> (x-y=w2431:u32)
                    n1004 = Greater?(x=w2431, y=u32 50) -> (0:w2429:bool)
                  }
                }
                n1005 = feedback-in #9(w2418) -> ()
                n1006 = Negate(x=w2420) -> (-x=w2421:dbl)
                n1007 = call-poly <vilib>:"WPI_RobotDriveArcadeDrive.vi"("Y axis value"=w2421, "X axis value"=0.0, "RobotDriveDevRef"=w2423) -> ("RobotDriveDevRef"=w2411:T2)  [unwired: 6 in, 2 out]
              }
            }
            frame #1 {
              n1008 = Tick Count (ms)() -> (millisecond timer value=w2435:u32)
              n1009 = global write "Robot Global Data.vi" "Arm Manual Speed"(0.0 ("Arm Manual Speed")) -> ()
              n1010 = global read "Robot Global Data.vi" "Continuos Yaw"() -> (w2436:dbl)
              n1011 = while {
                tunnel: w2434 -> [w2449]
                tunnel: w2436 -> [w2443]
                tunnel: w2435 -> [w2441]
                tunnel: [w2438] -> _
                stop <- w2445 stop-if-true
                n1012 = global read "Robot Global Data.vi" "Left Drive Encoder Stopped"() -> (w2448:bool)
                n1013 = global read "Robot Global Data.vi" "Continuos Yaw"() -> (w2444:dbl)
                n1014 = Subtract(x=w2444, y=w2443) -> (x-y=w2442:dbl)
                n1015 = call-poly <vilib>:"PID.vi"("output range"=cluster{"output high":dbl, "output low":dbl} {"output high"=0.7, "output low"=-0.7}, "PID gains"=T8 {"proportional gain (Kc)"=0.05, "integral time (Ti, min)"=0.0, "derivative time (Td, min)"=0.0} ("PID gains 5"), "process variable"=w2442, "setpoint"=90.0) -> ("output"=w2440:dbl)  [unwired: 6 in, 1 out]
                n1016 = feedback #10(w2441) -> (w2446:u32)
                n1017 = case shown="True" w2448 {
                  tunnel: w2446 -> [_ w2458]
                  tunnel: [w2454 w2458] -> w2447
                  tunnel: [FALSE w2455] -> w2445
                  frame False {
                    n1018 = Tick Count (ms)() -> (millisecond timer value=w2454:u32)
                  }
                  frame True {
                    n1019 = Tick Count (ms)() -> (millisecond timer value=w2459:u32)
                    n1020 = Subtract(x=w2459, y=w2458) -> (x-y=w2457:u32)
                    n1021 = Greater?(x=w2457, y=u32 50) -> (0:w2455:bool)
                  }
                }
                n1022 = feedback-in #10(w2447) -> ()
                n1023 = call-poly <vilib>:"WPI_RobotDriveArcadeDrive.vi"("Y axis value"=0.0, "X axis value"=w2440, "RobotDriveDevRef"=w2449) -> ("RobotDriveDevRef"=w2438:T2)  [unwired: 6 in, 2 out]
              }
            }
          }
        }
        frame "L" {
          n1024 = flat-sequence {
            tunnel: w2460 -> [w2469]
            tunnel: [w2465] -> w2464
            tunnel: w2464 -> [w2499]
            tunnel: [w2498] -> w2463
            tunnel: w2463 -> [w2530]
            tunnel: [w2525] -> w2462
            tunnel: w2462 -> [w2562]
            tunnel: [w2561] -> w2461
            tunnel: w2461 -> [_]
            frame #0 {
              n1025 = Tick Count (ms)() -> (millisecond timer value=w2467:u32)
              n1026 = global read "Robot Global Data.vi" "Left Drive Encoder Distance"() -> (w2468:dbl)
              n1027 = while {
                tunnel: w2469 -> [w2488]
                tunnel: w2468 -> [w2480]
                tunnel: w2467 -> [w2474]
                tunnel: [w2478] -> w2465
                stop <- w2472 stop-if-true
                n1028 = global read "Robot Global Data.vi" "Auto Scale Drive Forward Distance"() -> (w2470:dbl)
                n1029 = global read "Robot Global Data.vi" "Left Drive Encoder Distance"() -> (w2481:dbl)
                n1030 = global read "Robot Global Data.vi" "Left Drive Encoder Stopped"() -> (w2484:bool)
                n1031 = Tick Count (ms)() -> (millisecond timer value=w2477:u32)
                n1032 = Subtract(x=w2481, y=w2480) -> (x-y=w2479:dbl)
                n1033 = Subtract(x=w2477, y=w2474) -> (x-y=w2476:u32)
                n1034 = call-poly <vilib>:"PID.vi"("output range"=cluster{"output high":dbl, "output low":dbl} {"output high"=0.7, "output low"=-0.7}, "PID gains"=T8 {"proportional gain (Kc)"=0.07, "integral time (Ti, min)"=0.0, "derivative time (Td, min)"=0.0}, "process variable"=w2479, "setpoint"=w2470) -> ("output"=w2485:dbl)  [unwired: 6 in, 1 out]
                n1035 = Greater?(x=w2476, y=u32 250) -> (0:w2471:bool)
                n1036 = feedback #11(w2474) -> (w2482:u32)
                n1037 = case shown="True" w2484 {
                  tunnel: w2482 -> [_ w2496]
                  tunnel: [w2492 w2496] -> w2483
                  tunnel: [FALSE w2493] -> w2473
                  frame False {
                    n1038 = Tick Count (ms)() -> (millisecond timer value=w2492:u32)
                  }
                  frame True {
                    n1039 = Tick Count (ms)() -> (millisecond timer value=w2497:u32)
                    n1040 = Subtract(x=w2497, y=w2496) -> (x-y=w2495:u32)
                    n1041 = Greater?(x=w2495, y=u32 50) -> (0:w2493:bool)
                  }
                }
                n1042 = feedback-in #11(w2483) -> ()
                n1043 = Negate(x=w2485) -> (-x=w2486:dbl)
                n1044 = call-poly <vilib>:"WPI_RobotDriveArcadeDrive.vi"("Y axis value"=w2486, "X axis value"=0.0, "RobotDriveDevRef"=w2488) -> ("RobotDriveDevRef"=w2478:T2)  [unwired: 6 in, 2 out]
                n1045 = And(x=w2473, y=w2471) -> (x .and. y?=w2472:bool)
              }
              n1046 = global write "Robot Global Data.vi" "Arm Manual Speed"(0.2 ("Arm Manual Speed")) -> ()
            }
            frame #1 {
              n1047 = Tick Count (ms)() -> (millisecond timer value=w2500:u32)
              n1048 = global write "Robot Global Data.vi" "Arm Manual Speed"(0.0 ("Arm Manual Speed")) -> ()
              n1049 = global read "Robot Global Data.vi" "Continuos Yaw"() -> (w2501:dbl)
              n1050 = while {
                tunnel: w2499 -> [w2514]
                tunnel: w2501 -> [w2508]
                tunnel: w2500 -> [w2506]
                tunnel: [w2503] -> w2498
                stop <- w2510 stop-if-true
                n1051 = global read "Robot Global Data.vi" "Left Drive Encoder Stopped"() -> (w2513:bool)
                n1052 = global read "Robot Global Data.vi" "Continuos Yaw"() -> (w2509:dbl)
                n1053 = Subtract(x=w2509, y=w2508) -> (x-y=w2507:dbl)
                n1054 = call-poly <vilib>:"PID.vi"("output range"=cluster{"output high":dbl, "output low":dbl} {"output high"=0.7, "output low"=-0.7}, "PID gains"=T8 {"proportional gain (Kc)"=0.07, "integral time (Ti, min)"=0.0, "derivative time (Td, min)"=0.0} ("PID gains 2"), "process variable"=w2507, "setpoint"=90.0) -> ("output"=w2505:dbl)  [unwired: 6 in, 1 out]
                n1055 = feedback #12(w2506) -> (w2511:u32)
                n1056 = case shown="True" w2513 {
                  tunnel: w2511 -> [_ w2523]
                  tunnel: [w2519 w2523] -> w2512
                  tunnel: [FALSE w2520] -> w2510
                  frame False {
                    n1057 = Tick Count (ms)() -> (millisecond timer value=w2519:u32)
                  }
                  frame True {
                    n1058 = Tick Count (ms)() -> (millisecond timer value=w2524:u32)
                    n1059 = Subtract(x=w2524, y=w2523) -> (x-y=w2522:u32)
                    n1060 = Greater?(x=w2522, y=u32 50) -> (0:w2520:bool)
                  }
                }
                n1061 = feedback-in #12(w2512) -> ()
                n1062 = call-poly <vilib>:"WPI_RobotDriveArcadeDrive.vi"("Y axis value"=0.0, "X axis value"=w2505, "RobotDriveDevRef"=w2514) -> ("RobotDriveDevRef"=w2503:T2)  [unwired: 6 in, 2 out]
              }
            }
            frame #2 {
              n1063 = Tick Count (ms)() -> (millisecond timer value=w2529:u32)
              n1064 = global read "Robot Global Data.vi" "Left Drive Encoder Distance"() -> (w2531:dbl)
              n1065 = while {
                tunnel: w2530 -> [w2550]
                tunnel: w2531 -> [w2542]
                tunnel: w2529 -> [w2540]
                tunnel: [w2539] -> w2527
                tunnel: w2529 -> [w2535]
                stop <- w2534 stop-if-true
                n1066 = global read "Robot Global Data.vi" "Left Drive Encoder Distance"() -> (w2543:dbl)
                n1067 = global read "Robot Global Data.vi" "Left Drive Encoder Stopped"() -> (w2546:bool)
                n1068 = Subtract(x=w2543, y=w2542) -> (x-y=w2541:dbl)
                n1069 = Tick Count (ms)() -> (millisecond timer value=w2538:u32)
                n1070 = call-poly <vilib>:"PID.vi"("output range"=cluster{"output high":dbl, "output low":dbl} {"output high"=0.5, "output low"=-0.5}, "PID gains"=T8 {"proportional gain (Kc)"=0.07, "integral time (Ti, min)"=0.0, "derivative time (Td, min)"=0.0} ("PID gains 3"), "process variable"=w2541, "setpoint"=-20.0) -> ("output"=w2547:dbl)  [unwired: 6 in, 1 out]
                n1071 = Subtract(x=w2538, y=w2535) -> (x-y=w2537:u32)
                n1072 = feedback #13(w2540) -> (w2544:u32)
                n1073 = case shown="True" w2546 {
                  tunnel: w2544 -> [_ w2559]
                  tunnel: [w2555 w2559] -> w2545
                  tunnel: [FALSE w2556] -> w2533
                  frame False {
                    n1074 = Tick Count (ms)() -> (millisecond timer value=w2555:u32)
                  }
                  frame True {
                    n1075 = Tick Count (ms)() -> (millisecond timer value=w2560:u32)
                    n1076 = Subtract(x=w2560, y=w2559) -> (x-y=w2558:u32)
                    n1077 = Greater?(x=w2558, y=u32 50) -> (0:w2556:bool)
                  }
                }
                n1078 = feedback-in #13(w2545) -> ()
                n1079 = Greater?(x=w2537, y=u32 2000) -> (0:w2532:bool)
                n1080 = Negate(x=w2547) -> (-x=w2548:dbl)
                n1081 = call-poly <vilib>:"WPI_RobotDriveArcadeDrive.vi"("Y axis value"=w2548, "X axis value"=0.0, "RobotDriveDevRef"=w2550) -> ("RobotDriveDevRef"=w2539:T2)  [unwired: 6 in, 2 out]
                n1082 = Or(x=w2533, y=w2532) -> (x .or. y?=w2534:bool)
              }
              n1083 = global write "Robot Global Data.vi" "Intake Speed Override"(0.5 ("Intake Speed Override")) -> ()
              n1084 = call <vilib>:"WPI_RobotDriveDelayAndUpdateSafety.vi"("Delay (s)"=0.0, "RobotDriveDevRef"=w2527) -> ("RobotDriveDevRef 2"=w2525:T2)  [unwired: 8 in, 1 out]
            }
            frame #3 {
              n1085 = global write "Robot Global Data.vi" "Lift Height to rase to (in)"(60.0 ("Intake Speed Override")) -> ()
              n1086 = call <vilib>:"WPI_RobotDriveDelayAndUpdateSafety.vi"("Delay (s)"=1.75, "RobotDriveDevRef"=w2562) -> ("RobotDriveDevRef 2"=w2561:T2)  [unwired: 8 in, 1 out]
              n1087 = global write "Robot Global Data.vi" "Intake Speed Override"(0.0 ("Intake Speed Override")) -> ()
              n1088 = global write "Robot Global Data.vi" "Arm Angle to Turn to"(35.0 ("Intake Speed Override")) -> ()
              n1089 = global write "Robot Global Data.vi" "Arm Manual Control"(FALSE ("Arm Manual Control")) -> ()
            }
            frame #4 {
              n1090 = global write "Robot Global Data.vi" "Intake Speed Override"(-4.0 ("Intake Speed Override")) -> ()
            }
          }
        }
      }
    }
    frame "Basic Left Subvi" {
      n1091 = case shown="\"L\"" w2569 {
        tunnel: w2570 -> [w2572 w2606]
        frame "R", Default {
          n1092 = flat-sequence {
            tunnel: w2572 -> [w2574]
            tunnel: [w2573] -> w2571
            tunnel: w2571 -> [w2580]
            frame #0 {
              n1093 = call "Auto Drive Y.vi"("PID Gains"=T8 {"proportional gain (Kc)"=0.07, "integral time (Ti, min)"=0.0, "derivative time (Td, min)"=0.0} ("PID gains 4"), "Min Time (ms)"=u32 250, "Time to Settle (ms)"=u32 50, "Distance (in)"=200.0, "Motor Output Range"=cluster{"output high":dbl, "output low":dbl} {"output high"=0.7, "output low"=-0.7} ("output range"), "RobotDriveDevRef In"=w2574) -> ("RobotDriveDevRef Out"=w2573:T2)  [unwired: 5 in]
            }
            frame #1 {
              n1094 = Tick Count (ms)() -> (millisecond timer value=w2581:u32)
              n1095 = global write "Robot Global Data.vi" "Arm Manual Speed"(0.0 ("Arm Manual Speed")) -> ()
              n1096 = global read "Robot Global Data.vi" "Continuos Yaw"() -> (w2582:dbl)
              n1097 = while {
                tunnel: w2580 -> [w2595]
                tunnel: w2582 -> [w2589]
                tunnel: w2581 -> [w2587]
                tunnel: [w2584] -> _
                stop <- w2591 stop-if-true
                n1098 = global read "Robot Global Data.vi" "Left Drive Encoder Stopped"() -> (w2594:bool)
                n1099 = global read "Robot Global Data.vi" "Continuos Yaw"() -> (w2590:dbl)
                n1100 = Subtract(x=w2590, y=w2589) -> (x-y=w2588:dbl)
                n1101 = call-poly <vilib>:"PID.vi"("output range"=cluster{"output high":dbl, "output low":dbl} {"output high"=0.7, "output low"=-0.7}, "PID gains"=T8 {"proportional gain (Kc)"=0.05, "integral time (Ti, min)"=0.0, "derivative time (Td, min)"=0.0} ("PID gains 5"), "process variable"=w2588, "setpoint"=90.0) -> ("output"=w2586:dbl)  [unwired: 6 in, 1 out]
                n1102 = feedback #14(w2587) -> (w2592:u32)
                n1103 = case shown="True" w2594 {
                  tunnel: w2592 -> [_ w2604]
                  tunnel: [w2600 w2604] -> w2593
                  tunnel: [FALSE w2601] -> w2591
                  frame False {
                    n1104 = Tick Count (ms)() -> (millisecond timer value=w2600:u32)
                  }
                  frame True {
                    n1105 = Tick Count (ms)() -> (millisecond timer value=w2605:u32)
                    n1106 = Subtract(x=w2605, y=w2604) -> (x-y=w2603:u32)
                    n1107 = Greater?(x=w2603, y=u32 50) -> (0:w2601:bool)
                  }
                }
                n1108 = feedback-in #14(w2593) -> ()
                n1109 = call-poly <vilib>:"WPI_RobotDriveArcadeDrive.vi"("Y axis value"=0.0, "X axis value"=w2586, "RobotDriveDevRef"=w2595) -> ("RobotDriveDevRef"=w2584:T2)  [unwired: 6 in, 2 out]
              }
            }
          }
        }
        frame "L" {
          n1110 = flat-sequence {
            tunnel: w2606 -> [w2618]
            tunnel: [w2617] -> w2610
            tunnel: w2610 -> [w2627]
            tunnel: [w2626] -> w2609
            tunnel: w2609 -> [w2629]
            tunnel: [w2630] -> w2608
            tunnel: w2608 -> [w2639]
            tunnel: [w2638] -> w2607
            tunnel: w2607 -> [_]
            frame #0 {
              n1111 = global write "Robot Global Data.vi" "Arm Manual Speed"(0.2 ("Arm Manual Speed")) -> ()
              n1112 = call "Auto Drive Y.vi"("PID Gains"=T8 {"proportional gain (Kc)"=0.07, "integral time (Ti, min)"=0.0, "derivative time (Td, min)"=0.0}, "Max Time (ms)"=u32 15000, "Min Time (ms)"=u32 250, "Time to Settle (ms)"=u32 50, "Distance (in)"=15.0, "Motor Output Range"=cluster{"output high":dbl, "output low":dbl} {"output high"=0.7, "output low"=-0.7}, "RobotDriveDevRef In"=w2618) -> ("RobotDriveDevRef Out"=w2617:T2)  [unwired: 4 in]
            }
            frame #1 {
              n1113 = global write "Robot Global Data.vi" "Arm Manual Speed"(0.0 ("Arm Manual Speed")) -> ()
              n1114 = call "Auto Drive X.vi"("PID Gains"=T8 {"proportional gain (Kc)"=0.05, "integral time (Ti, min)"=0.0, "derivative time (Td, min)"=0.0}, "Settling Time (ms)"=u32 50, "Max Time (ms)"=u32 15000, "Min Time (ms)"=u32 250, "Angle to Turn (Deg)"=90.0, "Motor Output Range"=cluster{"output high":dbl, "output low":dbl} {"output high"=0.7, "output low"=-0.7}, "RobotDriveDevRef In"=w2627) -> ("RobotDriveDevRef Out"=w2626:T2)  [unwired: 4 in]
            }
            frame #2 {
              n1115 = global write "Robot Global Data.vi" "Intake Speed Override"(0.5 ("Intake Speed Override")) -> ()
              n1116 = call "Auto Drive Y.vi"("PID Gains"=T8 {"proportional gain (Kc)"=0.07, "integral time (Ti, min)"=0.0, "derivative time (Td, min)"=0.0}, "Max Time (ms)"=u32 2000, "Min Time (ms)"=u32 250, "Time to Settle (ms)"=u32 50, "Distance (in)"=-20.0, "Motor Output Range"=cluster{"output high":dbl, "output low":dbl} {"output high"=0.5, "output low"=-0.5}, "RobotDriveDevRef In"=w2629) -> ("RobotDriveDevRef Out"=w2630:T2)  [unwired: 4 in]
            }
            frame #3 {
              n1117 = global write "Robot Global Data.vi" "Intake Speed Override"(0.0 ("Intake Speed Override")) -> ()
              n1118 = global write "Robot Global Data.vi" "Arm Manual Control"(FALSE ("Arm Manual Control")) -> ()
              n1119 = global write "Robot Global Data.vi" "Lift Height to rase to (in)"(60.0 ("Intake Speed Override")) -> ()
              n1120 = global write "Robot Global Data.vi" "Arm Angle to Turn to"(80.0 ("Intake Speed Override")) -> ()
              n1121 = call <vilib>:"WPI_RobotDriveDelayAndUpdateSafety.vi"("Delay (s)"=1.75, "RobotDriveDevRef"=w2639) -> ("RobotDriveDevRef 2"=w2638:T2)  [unwired: 8 in, 1 out]
            }
            frame #4 {
              n1122 = global write "Robot Global Data.vi" "Intake Speed Override"(-4.0 ("Intake Speed Override")) -> ()
            }
          }
        }
      }
    }
    frame "Basic Right" {
      n1123 = case shown="\"R\", Default" w2646 {
        tunnel: w2647 -> [w2648 w2758]
        frame "R", Default {
          n1124 = flat-sequence {
            tunnel: w2648 -> [w2657]
            tunnel: [w2653] -> w2652
            tunnel: w2652 -> [w2687]
            tunnel: [w2686] -> w2651
            tunnel: w2651 -> [w2718]
            tunnel: [w2713] -> w2650
            tunnel: w2650 -> [w2750]
            tunnel: [w2749] -> w2649
            tunnel: w2649 -> [_]
            frame #0 {
              n1125 = Tick Count (ms)() -> (millisecond timer value=w2655:u32)
              n1126 = global read "Robot Global Data.vi" "Left Drive Encoder Distance"() -> (w2656:dbl)
              n1127 = while {
                tunnel: w2657 -> [w2676]
                tunnel: w2656 -> [w2668]
                tunnel: w2655 -> [w2662]
                tunnel: [w2666] -> w2653
                stop <- w2660 stop-if-true
                n1128 = global read "Robot Global Data.vi" "Auto Scale Drive Forward Distance"() -> (w2658:dbl)
                n1129 = global read "Robot Global Data.vi" "Left Drive Encoder Distance"() -> (w2669:dbl)
                n1130 = global read "Robot Global Data.vi" "Left Drive Encoder Stopped"() -> (w2672:bool)
                n1131 = Tick Count (ms)() -> (millisecond timer value=w2665:u32)
                n1132 = Subtract(x=w2669, y=w2668) -> (x-y=w2667:dbl)
                n1133 = Subtract(x=w2665, y=w2662) -> (x-y=w2664:u32)
                n1134 = call-poly <vilib>:"PID.vi"("output range"=cluster{"output high":dbl, "output low":dbl} {"output high"=0.7, "output low"=-0.7}, "PID gains"=T8 {"proportional gain (Kc)"=0.07, "integral time (Ti, min)"=0.0, "derivative time (Td, min)"=0.0}, "process variable"=w2667, "setpoint"=w2658) -> ("output"=w2673:dbl)  [unwired: 6 in, 1 out]
                n1135 = Greater?(x=w2664, y=u32 250) -> (0:w2659:bool)
                n1136 = feedback #15(w2662) -> (w2670:u32)
                n1137 = case shown="True" w2672 {
                  tunnel: w2670 -> [_ w2684]
                  tunnel: [w2680 w2684] -> w2671
                  tunnel: [FALSE w2681] -> w2661
                  frame False {
                    n1138 = Tick Count (ms)() -> (millisecond timer value=w2680:u32)
                  }
                  frame True {
                    n1139 = Tick Count (ms)() -> (millisecond timer value=w2685:u32)
                    n1140 = Subtract(x=w2685, y=w2684) -> (x-y=w2683:u32)
                    n1141 = Greater?(x=w2683, y=u32 50) -> (0:w2681:bool)
                  }
                }
                n1142 = feedback-in #15(w2671) -> ()
                n1143 = Negate(x=w2673) -> (-x=w2674:dbl)
                n1144 = call-poly <vilib>:"WPI_RobotDriveArcadeDrive.vi"("Y axis value"=w2674, "X axis value"=0.0, "RobotDriveDevRef"=w2676) -> ("RobotDriveDevRef"=w2666:T2)  [unwired: 6 in, 2 out]
                n1145 = And(x=w2661, y=w2659) -> (x .and. y?=w2660:bool)
              }
              n1146 = global write "Robot Global Data.vi" "Arm Manual Speed"(0.2 ("Arm Manual Speed")) -> ()
            }
            frame #1 {
              n1147 = Tick Count (ms)() -> (millisecond timer value=w2688:u32)
              n1148 = global write "Robot Global Data.vi" "Arm Manual Speed"(0.0 ("Arm Manual Speed")) -> ()
              n1149 = global read "Robot Global Data.vi" "Continuos Yaw"() -> (w2689:dbl)
              n1150 = while {
                tunnel: w2687 -> [w2702]
                tunnel: w2689 -> [w2696]
                tunnel: w2688 -> [w2694]
                tunnel: [w2691] -> w2686
                stop <- w2698 stop-if-true
                n1151 = global read "Robot Global Data.vi" "Left Drive Encoder Stopped"() -> (w2701:bool)
                n1152 = global read "Robot Global Data.vi" "Continuos Yaw"() -> (w2697:dbl)
                n1153 = Subtract(x=w2697, y=w2696) -> (x-y=w2695:dbl)
                n1154 = call-poly <vilib>:"PID.vi"("output range"=cluster{"output high":dbl, "output low":dbl} {"output high"=0.7, "output low"=-0.7}, "PID gains"=T8 {"proportional gain (Kc)"=0.07, "integral time (Ti, min)"=0.0, "derivative time (Td, min)"=0.0} ("PID gains 2"), "process variable"=w2695, "setpoint"=-90.0) -> ("output"=w2693:dbl)  [unwired: 6 in, 1 out]
                n1155 = feedback #16(w2694) -> (w2699:u32)
                n1156 = case shown="True" w2701 {
                  tunnel: w2699 -> [_ w2711]
                  tunnel: [w2707 w2711] -> w2700
                  tunnel: [FALSE w2708] -> w2698
                  frame False {
                    n1157 = Tick Count (ms)() -> (millisecond timer value=w2707:u32)
                  }
                  frame True {
                    n1158 = Tick Count (ms)() -> (millisecond timer value=w2712:u32)
                    n1159 = Subtract(x=w2712, y=w2711) -> (x-y=w2710:u32)
                    n1160 = Greater?(x=w2710, y=u32 50) -> (0:w2708:bool)
                  }
                }
                n1161 = feedback-in #16(w2700) -> ()
                n1162 = call-poly <vilib>:"WPI_RobotDriveArcadeDrive.vi"("Y axis value"=0.0, "X axis value"=w2693, "RobotDriveDevRef"=w2702) -> ("RobotDriveDevRef"=w2691:T2)  [unwired: 6 in, 2 out]
              }
            }
            frame #2 {
              n1163 = Tick Count (ms)() -> (millisecond timer value=w2717:u32)
              n1164 = global read "Robot Global Data.vi" "Left Drive Encoder Distance"() -> (w2719:dbl)
              n1165 = while {
                tunnel: w2718 -> [w2738]
                tunnel: w2719 -> [w2730]
                tunnel: w2717 -> [w2728]
                tunnel: [w2727] -> w2715
                tunnel: w2717 -> [w2723]
                stop <- w2722 stop-if-true
                n1166 = global read "Robot Global Data.vi" "Left Drive Encoder Distance"() -> (w2731:dbl)
                n1167 = global read "Robot Global Data.vi" "Left Drive Encoder Stopped"() -> (w2734:bool)
                n1168 = Subtract(x=w2731, y=w2730) -> (x-y=w2729:dbl)
                n1169 = Tick Count (ms)() -> (millisecond timer value=w2726:u32)
                n1170 = call-poly <vilib>:"PID.vi"("output range"=cluster{"output high":dbl, "output low":dbl} {"output high"=0.5, "output low"=-0.5}, "PID gains"=T8 {"proportional gain (Kc)"=0.07, "integral time (Ti, min)"=0.0, "derivative time (Td, min)"=0.0} ("PID gains 3"), "process variable"=w2729, "setpoint"=-20.0) -> ("output"=w2735:dbl)  [unwired: 6 in, 1 out]
                n1171 = Subtract(x=w2726, y=w2723) -> (x-y=w2725:u32)
                n1172 = feedback #17(w2728) -> (w2732:u32)
                n1173 = case shown="True" w2734 {
                  tunnel: w2732 -> [_ w2747]
                  tunnel: [w2743 w2747] -> w2733
                  tunnel: [FALSE w2744] -> w2721
                  frame False {
                    n1174 = Tick Count (ms)() -> (millisecond timer value=w2743:u32)
                  }
                  frame True {
                    n1175 = Tick Count (ms)() -> (millisecond timer value=w2748:u32)
                    n1176 = Subtract(x=w2748, y=w2747) -> (x-y=w2746:u32)
                    n1177 = Greater?(x=w2746, y=u32 50) -> (0:w2744:bool)
                  }
                }
                n1178 = feedback-in #17(w2733) -> ()
                n1179 = Greater?(x=w2725, y=u32 2000) -> (0:w2720:bool)
                n1180 = Negate(x=w2735) -> (-x=w2736:dbl)
                n1181 = call-poly <vilib>:"WPI_RobotDriveArcadeDrive.vi"("Y axis value"=w2736, "X axis value"=0.0, "RobotDriveDevRef"=w2738) -> ("RobotDriveDevRef"=w2727:T2)  [unwired: 6 in, 2 out]
                n1182 = Or(x=w2721, y=w2720) -> (x .or. y?=w2722:bool)
              }
              n1183 = global write "Robot Global Data.vi" "Intake Speed Override"(0.5 ("Intake Speed Override")) -> ()
              n1184 = call <vilib>:"WPI_RobotDriveDelayAndUpdateSafety.vi"("Delay (s)"=0.0, "RobotDriveDevRef"=w2715) -> ("RobotDriveDevRef 2"=w2713:T2)  [unwired: 8 in, 1 out]
            }
            frame #3 {
              n1185 = global write "Robot Global Data.vi" "Lift Height to rase to (in)"(60.0 ("Intake Speed Override")) -> ()
              n1186 = call <vilib>:"WPI_RobotDriveDelayAndUpdateSafety.vi"("Delay (s)"=1.75, "RobotDriveDevRef"=w2750) -> ("RobotDriveDevRef 2"=w2749:T2)  [unwired: 8 in, 1 out]
              n1187 = global write "Robot Global Data.vi" "Intake Speed Override"(0.0 ("Intake Speed Override")) -> ()
              n1188 = global write "Robot Global Data.vi" "Arm Angle to Turn to"(35.0 ("Intake Speed Override")) -> ()
              n1189 = global write "Robot Global Data.vi" "Arm Manual Control"(FALSE ("Arm Manual Control")) -> ()
            }
            frame #4 {
              n1190 = global write "Robot Global Data.vi" "Intake Speed Override"(-4.0 ("Intake Speed Override")) -> ()
            }
          }
        }
        frame "L" {
          n1191 = flat-sequence {
            tunnel: w2758 -> [w2761]
            tunnel: [w2760] -> w2757
            tunnel: w2757 -> [w2800]
            frame #0 {
              n1192 = Tick Count (ms)() -> (millisecond timer value=w2762:u32)
              n1193 = global read "Robot Global Data.vi" "Encoders to use"() -> (w2759:u16)
              n1194 = case shown="1" w2759 {
                tunnel: [_ w2764 w2765] -> w2763
                frame 0, Default {
                }
                frame 1 {
                  n1195 = global read "Robot Global Data.vi" "Right Drive Encoder Distance"() -> (w2764:dbl)
                }
                frame 2 {
                  n1196 = global read "Robot Global Data.vi" "Left Drive Encoder Distance"() -> (w2765:dbl)
                }
              }
              n1197 = while {
                tunnel: w2761 -> [w2785]
                tunnel: w2763 -> [w2779]
                tunnel: w2762 -> [w2773]
                tunnel: [w2777] -> w2760
                stop <- w2771 stop-if-true
                n1198 = Tick Count (ms)() -> ()  [unwired: 1 out]
                n1199 = global read "Robot Global Data.vi" "Encoders to use"() -> (w2769:u16)
                n1200 = case shown="1" w2769 {
                  tunnel: [_ w2791 w2792] -> w2768
                  frame 0, Default {
                  }
                  frame 1 {
                    n1201 = global read "Robot Global Data.vi" "Right Drive Encoder Distance"() -> (w2791:dbl)
                  }
                  frame 2 {
                    n1202 = global read "Robot Global Data.vi" "Left Drive Encoder Distance"() -> (w2792:dbl)
                  }
                }
                n1203 = global read "Robot Global Data.vi" "Encoders to use"() -> (w2767:u16)
                n1204 = case shown="2" w2767 {
                  tunnel: [_ w2789 w2790] -> w2766
                  frame 0, Default {
                  }
                  frame 1 {
                    n1205 = global read "Robot Global Data.vi" "Right Drive Encoder Stopped"() -> (w2789:bool)
                  }
                  frame 2 {
                    n1206 = global read "Robot Global Data.vi" "Left Drive Encoder Stopped"() -> (w2790:bool)
                  }
                }
                n1207 = Subtract(x=w2768, y=w2779) -> (x-y=w2778:dbl)
                n1208 = Tick Count (ms)() -> (millisecond timer value=w2776:u32)
                n1209 = call-poly <vilib>:"PID.vi"("output range"=cluster{"output high":dbl, "output low":dbl} {"output high"=0.7, "output low"=-0.7}, "PID gains"=T8 {"proportional gain (Kc)"=0.07, "integral time (Ti, min)"=0.0, "derivative time (Td, min)"=0.0} ("PID gains 4"), "process variable"=w2778, "setpoint"=200.0) -> ("output"=w2782:dbl)  [unwired: 6 in, 1 out]
                n1210 = Subtract(x=w2776, y=w2773) -> (x-y=w2775:u32)
                n1211 = feedback #18(w2773) -> (w2780:u32)
                n1212 = case shown="True" w2766 {
                  tunnel: w2780 -> [_ w2798]
                  tunnel: [w2794 w2798] -> w2781
                  tunnel: [FALSE w2795] -> w2772
                  frame False {
                    n1213 = Tick Count (ms)() -> (millisecond timer value=w2794:u32)
                  }
                  frame True {
                    n1214 = Tick Count (ms)() -> (millisecond timer value=w2799:u32)
                    n1215 = Subtract(x=w2799, y=w2798) -> (x-y=w2797:u32)
                    n1216 = Greater?(x=w2797, y=u32 100) -> (0:w2795:bool)
                  }
                }
                n1217 = feedback-in #18(w2781) -> ()
                n1218 = Negate(x=w2782) -> (-x=w2783:dbl)
                n1219 = Greater?(x=w2775, y=u32 1000) -> (0:w2770:bool)
                n1220 = call-poly <vilib>:"WPI_RobotDriveArcadeDrive.vi"("Y axis value"=w2783, "X axis value"=0.0, "RobotDriveDevRef"=w2785) -> ("RobotDriveDevRef"=w2777:T2)  [unwired: 6 in, 2 out]
                n1221 = And(x=w2772, y=w2770) -> (x .and. y?=w2771:bool)
              }
            }
            frame #1 {
              n1222 = Tick Count (ms)() -> (millisecond timer value=w2801:u32)
              n1223 = global write "Robot Global Data.vi" "Arm Manual Speed"(0.0 ("Arm Manual Speed")) -> ()
              n1224 = global read "Robot Global Data.vi" "Continuos Yaw"() -> (w2802:dbl)
              n1225 = while {
                tunnel: w2800 -> [w2816]
                tunnel: w2802 -> [w2811]
                tunnel: w2801 -> [w2809]
                tunnel: [w2806] -> _
                stop <- w2813 stop-if-true
                n1226 = global read "Robot Global Data.vi" "Continuos Yaw"() -> (w2812:dbl)
                n1227 = global read "Robot Global Data.vi" "Encoders to use"() -> (w2805:u16)
                n1228 = case shown="2" w2805 {
                  tunnel: [_ w2820 w2821] -> w2804
                  frame 0, Default {
                  }
                  frame 1 {
                    n1229 = global read "Robot Global Data.vi" "Right Drive Encoder Stopped"() -> (w2820:bool)
                  }
                  frame 2 {
                    n1230 = global read "Robot Global Data.vi" "Left Drive Encoder Stopped"() -> (w2821:bool)
                  }
                }
                n1231 = Subtract(x=w2812, y=w2811) -> (x-y=w2810:dbl)
                n1232 = call-poly <vilib>:"PID.vi"("output range"=cluster{"output high":dbl, "output low":dbl} {"output high"=0.7, "output low"=-0.7}, "PID gains"=T8 {"proportional gain (Kc)"=0.05, "integral time (Ti, min)"=0.0, "derivative time (Td, min)"=0.0} ("PID gains 5"), "process variable"=w2810, "setpoint"=-90.0) -> ("output"=w2808:dbl)  [unwired: 6 in, 1 out]
                n1233 = feedback #19(w2809) -> (w2814:u32)
                n1234 = case shown="True" w2804 {
                  tunnel: w2814 -> [_ w2827]
                  tunnel: [w2823 w2827] -> w2815
                  tunnel: [FALSE w2824] -> w2813
                  frame False {
                    n1235 = Tick Count (ms)() -> (millisecond timer value=w2823:u32)
                  }
                  frame True {
                    n1236 = Tick Count (ms)() -> (millisecond timer value=w2828:u32)
                    n1237 = Subtract(x=w2828, y=w2827) -> (x-y=w2826:u32)
                    n1238 = Greater?(x=w2826, y=u32 100) -> (0:w2824:bool)
                  }
                }
                n1239 = feedback-in #19(w2815) -> ()
                n1240 = call-poly <vilib>:"WPI_RobotDriveArcadeDrive.vi"("Y axis value"=0.0, "X axis value"=w2808, "RobotDriveDevRef"=w2816) -> ("RobotDriveDevRef"=w2806:T2)  [unwired: 6 in, 2 out]
              }
            }
          }
        }
      }
    }
  }
